vi "Monitor-BNET01.vi"() -> ()   [LabVIEW 2013]
uses:
  <vilib>/Utility/miscctls.llb/LVPoint32TypeDef.ctl
  data/ControlCAN.dll
panel:
  out "数据保存":bool
  out "强制操作":bool
  out "参数生成":bool
  out "参数配置":bool
  in  "保存间隔(S)":T1(ring)=enum."0.2"
  out "文件序号":u32
  out "dup path":path
  out "开始保存":bool
  out "BMS供电电压":dbl
  out "字符串":string="         （菜单可更改CAN设置)请连接CAN设备-------->"
  out "CAN初始化成功":bool
  out "CP":u8
  out "CC":dbl
  out "CC2":dbl
  out "AI1":dbl
  out "AI2":dbl
  out "平均电流":dbl
  out "外总压":dbl
  out "从板个数":u8
  out "Life":string="0"
  out "DO2":bool
  out "DO1":bool
  out "DI4":bool
  out "DI3":bool
  out "DI2":bool
  out "DI1":bool
  out "总正":bool
  out "总负":bool
  out "预充":bool
  out "充电":bool
  out "风机":bool
  out "加热":bool
  in  "总电压进度":u16(ring)
  in  "总电流进度":u16(ring)
  out "VCI_Receive 2":T2={"ID"=67604736, "TimeStamp"=193019994, "TimeFlag"=1, "SendType"=0, "RemoteFlag"=0, "ExternFlag"=1, "DataLen"=8, "Data1"=1, "Data2"=0, "Data3"=0, "Data4"=85, "Data5"=59, "Data6"=0, "Data7"=0, "Data8"=30, "Rsv1"=0, "Rsv2"=0, "Rsv3"=0}
  in  "动作保持时间":dbl=100000.0
  in  "故障信息":bool caption="查看高压板监控"
  in  "系统信息":bool caption="查看高压板监控"
  out "温度个数":i32
  out "大小":i32
  out "X标尺.刻度值[]":dbl[](array[numeric])
  out "坐标 2":T3 caption="坐标"
  in  "充电信息":bool caption="查看高压板监控"
  out "CAN 操作结果":bool=TRUE
  out "充电继电器 2":u16(ring) caption="风机继电器" items=["未闭合", "闭合", "故障", "保留"]
  out "加热继电器":u16(ring) caption="预充电继电器" items=["未闭合", "闭合", "故障", "保留"]
  in  "单箱信息":bool caption="查看高压板监控"
  in  "单板信息 3":bool caption="查看高压板监控"
  in  "诊断标定":bool caption="查看高压板监控"
  in  "电压温度":bool caption="查看高压板监控"
  in  "数据刷新":bool caption="全部监控"
  in  "保存数据 3":bool caption="全部监控"
  in  "CAN连接":bool caption="启动CAN"
  in  "参数设置":bool caption="启动CAN"
  in  "退出":bool caption="全部监控"
  in  "帮助":bool caption="全部监控"
  in  "Life超时":i32
  in  "模拟发送":bool
  out "充电超时2":i32
  out "充电超时1":i32
  out "P_IsInternal_B":bool
  in  "判定3":bool=TRUE
  in  "计数 2":i32
  in  "计数1":i32=26826
  out "电池故障4 4":u8
  out "电池故障3 4":u8
  out "电池故障2 4":u8
  out "电池故障 5":u8
  in  "数值":i32
  out "继电器状态":string[][](array[string])=[["", "", "", "", "", "", "", "", "", "", "", "", "", "", "", "", "", "", "", "", "", "", "", "", "", "", "", "", "", "", "0"], ["", "", "", "", "", "", "", "", "", "", "", "", "", "", "", "", "", "", "", "", "", "", "", "", "", "", "", "", "", "", "0"]]
  out "从板参数":T4(array[cluster])=[{"总电压"=0.0, "总电流"=0.0, "外总压"=0.0, "平均电流"=0.0, "SOC"=60.0, "SOH"=60.0, "最高电压"=0.0, "位置"=0.0, "最低电压"=0.0, "位置"=0.0, "压差"=0.0, "最高温度"=0.0, "位置"=0.0, "最低温度"=0.0, "位置"=0.0, "最大内阻"=0.0, "位置"=0.0, "最小内阻"=0.0, "位置"=0.0, "故障信息"="", "协议版本号"="", "应用类型"="", "波特率"="", "协议是否公开"="", "电池运行状态"="", "电池充满标志位"="", "Life:"=25.0}, {"总电压"=0.0, "总电流"=0.0, "外总压"=0.0, "平均电流"=0.0, "SOC"=60.0, "SOH"=60.0, "最高电压"=0.0, "位置"=0.0, "最低电压"=0.0, "位置"=0.0, "压差"=0.0, "最高温度"=0.0, "位置"=0.0, "最低温度"=0.0, "位置"=0.0, "最大内阻"=0.0, "位置"=0.0, "最小内阻"=0.0, "位置"=0.0, "故障信息"="", "协议版本号"="", "应用类型"="", "波特率"="", "协议是否公开"="", "电池运行状态"="", "电池充满标志位"="", "Life:"=25.0}, {"总电压"=0.0, "总电流"=0.0, "外总压"=0.0, "平均电流"=0.0, "SOC"=60.0, "SOH"=60.0, "最高电压"=0.0, "位置"=0.0, "最低电压"=0.0, "位置"=0.0, "压差"=0.0, "最高温度"=0.0, "位置"=0.0, "最低温度"=0.0, "位置"=0.0, "最大内阻"=0.0, "位置"=0.0, "最小内阻"=0.0, "位置"=0.0, "故障信息"="", "协议版本号"="", "应用类型"="", "波特率"="", "协议是否公开"="", "电池运行状态"="", "电池充满标志位"="", "Life:"=25.0}, {"总电压"=0.0, "总电流"=0.0, "外总压"=0.0, "平均电流"=0.0, "SOC"=60.0, "SOH"=60.0, "最高电压"=0.0, "位置"=0.0, "最低电压"=0.0, "位置"=0.0, "压差"=0.0, "最高温度"=0.0, "位置"=0.0, "最低温度"=0.0, "位置"=0.0, "最大内阻"=0.0, "位置"=0.0, "最小内阻"=0.0, "位置"=0.0, "故障信息"="", "协议版本号"="", "应用类型"="", "波特率"="", "协议是否公开"="", "电池运行状态"="", "电池充满标志位"="", "Life:"=25.0}, {"总电压"=0.0, "总电流"=0.0, "外总压"=0.0, "平均电流"=0.0, "SOC"=60.0, "SOH"=60.0, "最高电压"=0.0, "位置"=0.0, "最低电压"=0.0, "位置"=0.0, "压差"=0.0, "最高温度"=0.0, "位置"=0.0, "最低温度"=0.0, "位置"=0.0, "最大内阻"=0.0, "位置"=0.0, "最小内阻"=0.0, "位置"=0.0, "故障信息"="", "协议版本号"="", "应用类型"="", "波特率"="", "协议是否公开"="", "电池运行状态"="", "电池充满标志位"="", "Life:"=25.0}, {"总电压"=0.0, "总电流"=0.0, "外总压"=0.0, "平均电流"=0.0, "SOC"=60.0, "SOH"=60.0, "最高电压"=0.0, "位置"=0.0, "最低电压"=0.0, "位置"=0.0, "压差"=0.0, "最高温度"=0.0, "位置"=0.0, "最低温度"=0.0, "位置"=0.0, "最大内阻"=0.0, "位置"=0.0, "最小内阻"=0.0, "位置"=0.0, "故障信息"="", "协议版本号"="", "应用类型"="", "波特率"="", "协议是否公开"="", "电池运行状态"="", "电池充满标志位"="", "Life:"=25.0}, {"总电压"=0.0, "总电流"=0.0, "外总压"=0.0, "平均电流"=0.0, "SOC"=60.0, "SOH"=60.0, "最高电压"=0.0, "位置"=0.0, "最低电压"=0.0, "位置"=0.0, "压差"=0.0, "最高温度"=0.0, "位置"=0.0, "最低温度"=0.0, "位置"=0.0, "最大内阻"=0.0, "位置"=0.0, "最小内阻"=0.0, "位置"=0.0, "故障信息"="", "协议版本号"="", "应用类型"="", "波特率"="", "协议是否公开"="", "电池运行状态"="", "电池充满标志位"="", "Life:"=25.0}, {"总电压"=0.0, "总电流"=0.0, "外总压"=0.0, "平均电流"=0.0, "SOC"=60.0, "SOH"=60.0, "最高电压"=0.0, "位置"=0.0, "最低电压"=0.0, "位置"=0.0, "压差"=0.0, "最高温度"=0.0, "位置"=0.0, "最低温度"=0.0, "位置"=0.0, "最大内阻"=0.0, "位置"=0.0, "最小内阻"=0.0, "位置"=0.0, "故障信息"="", "协议版本号"="", "应用类型"="", "波特率"="", "协议是否公开"="", "电池运行状态"="", "电池充满标志位"="", "Life:"=25.0}, {"总电压"=0.0, "总电流"=0.0, "外总压"=0.0, "平均电流"=0.0, "SOC"=60.0, "SOH"=60.0, "最高电压"=0.0, "位置"=0.0, "最低电压"=0.0, "位置"=0.0, "压差"=0.0, "最高温度"=0.0, "位置"=0.0, "最低温度"=0.0, "位置"=0.0, "最大内阻"=0.0, "位置"=0.0, "最小内阻"=0.0, "位置"=0.0, "故障信息"="", "协议版本号"="", "应用类型"="", "波特率"="", "协议是否公开"="", "电池运行状态"="", "电池充满标志位"="", "Life:"=25.0}, {"总电压"=0.0, "总电流"=0.0, "外总压"=0.0, "平均电流"=0.0, "SOC"=60.0, "SOH"=60.0, "最高电压"=0.0, "位置"=0.0, "最低电压"=0.0, "位置"=0.0, "压差"=0.0, "最高温度"=0.0, "位置"=0.0, "最低温度"=0.0, "位置"=0.0, "最大内阻"=0.0, "位置"=0.0, "最小内阻"=0.0, "位置"=0.0, "故障信息"="", "协议版本号"="", "应用类型"="", "波特率"="", "协议是否公开"="", "电池运行状态"="", "电池充满标志位"="", "Life:"=25.0}, {"总电压"=0.0, "总电流"=0.0, "外总压"=0.0, "平均电流"=0.0, "SOC"=60.0, "SOH"=60.0, "最高电压"=0.0, "位置"=0.0, "最低电压"=0.0, "位置"=0.0, "压差"=0.0, "最高温度"=0.0, "位置"=0.0, "最低温度"=0.0, "位置"=0.0, "最大内阻"=0.0, "位置"=0.0, "最小内阻"=0.0, "位置"=0.0, "故障信息"="", "协议版本号"="", "应用类型"="", "波特率"="", "协议是否公开"="", "电池运行状态"="", "电池充满标志位"="", "Life:"=25.0}, {"总电压"=0.0, "总电流"=0.0, "外总压"=0.0, "平均电流"=0.0, "SOC"=60.0, "SOH"=60.0, "最高电压"=0.0, "位置"=0.0, "最低电压"=0.0, "位置"=0.0, "压差"=0.0, "最高温度"=0.0, "位置"=0.0, "最低温度"=0.0, "位置"=0.0, "最大内阻"=0.0, "位置"=0.0, "最小内阻"=0.0, "位置"=0.0, "故障信息"="", "协议版本号"="", "应用类型"="", "波特率"="", "协议是否公开"="", "电池运行状态"="", "电池充满标志位"="", "Life:"=25.0}, {"总电压"=0.0, "总电流"=0.0, "外总压"=0.0, "平均电流"=0.0, "SOC"=60.0, "SOH"=60.0, "最高电压"=0.0, "位置"=0.0, "最低电压"=0.0, "位置"=0.0, "压差"=0.0, "最高温度"=0.0, "位置"=0.0, "最低温度"=0.0, "位置"=0.0, "最大内阻"=0.0, "位置"=0.0, "最小内阻"=0.0, "位置"=0.0, "故障信息"="", "协议版本号"="", "应用类型"="", "波特率"="", "协议是否公开"="", "电池运行状态"="", "电池充满标志位"="", "Life:"=25.0}, {"总电压"=0.0, "总电流"=0.0, "外总压"=0.0, "平均电流"=0.0, "SOC"=60.0, "SOH"=60.0, "最高电压"=0.0, "位置"=0.0, "最低电压"=0.0, "位置"=0.0, "压差"=0.0, "最高温度"=0.0, "位置"=0.0, "最低温度"=0.0, "位置"=0.0, "最大内阻"=0.0, "位置"=0.0, "最小内阻"=0.0, "位置"=0.0, "故障信息"="", "协议版本号"="", "应用类型"="", "波特率"="", "协议是否公开"="", "电池运行状态"="", "电池充满标志位"="", "Life:"=25.0}, {"总电压"=0.0, "总电流"=0.0, "外总压"=0.0, "平均电流"=0.0, "SOC"=60.0, "SOH"=60.0, "最高电压"=0.0, "位置"=0.0, "最低电压"=0.0, "位置"=0.0, "压差"=0.0, "最高温度"=0.0, "位置"=0.0, "最低温度"=0.0, "位置"=0.0, "最大内阻"=0.0, "位置"=0.0, "最小内阻"=0.0, "位置"=0.0, "故障信息"="", "协议版本号"="", "应用类型"="", "波特率"="", "协议是否公开"="", "电池运行状态"="", "电池充满标志位"="", "Life:"=25.0}, {"总电压"=0.0, "总电流"=0.0, "外总压"=0.0, "平均电流"=0.0, "SOC"=60.0, "SOH"=60.0, "最高电压"=0.0, "位置"=0.0, "最低电压"=0.0, "位置"=0.0, "压差"=0.0, "最高温度"=0.0, "位置"=0.0, "最低温度"=0.0, "位置"=0.0, "最大内阻"=0.0, "位置"=0.0, "最小内阻"=0.0, "位置"=0.0, "故障信息"="", "协议版本号"="", "应用类型"="", "波特率"="", "协议是否公开"="", "电池运行状态"="", "电池充满标志位"="", "Life:"=25.0}, {"总电压"=0.0, "总电流"=0.0, "外总压"=0.0, "平均电流"=0.0, "SOC"=60.0, "SOH"=60.0, "最高电压"=0.0, "位置"=0.0, "最低电压"=0.0, "位置"=0.0, "压差"=0.0, "最高温度"=0.0, "位置"=0.0, "最低温度"=0.0, "位置"=0.0, "最大内阻"=0.0, "位置"=0.0, "最小内阻"=0.0, "位置"=0.0, "故障信息"="", "协议版本号"="", "应用类型"="", "波特率"="", "协议是否公开"="", "电池运行状态"="", "电池充满标志位"="", "Life:"=25.0}, {"总电压"=0.0, "总电流"=0.0, "外总压"=0.0, "平均电流"=0.0, "SOC"=60.0, "SOH"=60.0, "最高电压"=0.0, "位置"=0.0, "最低电压"=0.0, "位置"=0.0, "压差"=0.0, "最高温度"=0.0, "位置"=0.0, "最低温度"=0.0, "位置"=0.0, "最大内阻"=0.0, "位置"=0.0, "最小内阻"=0.0, "位置"=0.0, "故障信息"="", "协议版本号"="", "应用类型"="", "波特率"="", "协议是否公开"="", "电池运行状态"="", "电池充满标志位"="", "Life:"=25.0}, {"总电压"=0.0, "总电流"=0.0, "外总压"=0.0, "平均电流"=0.0, "SOC"=60.0, "SOH"=60.0, "最高电压"=0.0, "位置"=0.0, "最低电压"=0.0, "位置"=0.0, "压差"=0.0, "最高温度"=0.0, "位置"=0.0, "最低温度"=0.0, "位置"=0.0, "最大内阻"=0.0, "位置"=0.0, "最小内阻"=0.0, "位置"=0.0, "故障信息"="", "协议版本号"="", "应用类型"="", "波特率"="", "协议是否公开"="", "电池运行状态"="", "电池充满标志位"="", "Life:"=25.0}, {"总电压"=0.0, "总电流"=0.0, "外总压"=0.0, "平均电流"=0.0, "SOC"=60.0, "SOH"=60.0, "最高电压"=0.0, "位置"=0.0, "最低电压"=0.0, "位置"=0.0, "压差"=0.0, "最高温度"=0.0, "位置"=0.0, "最低温度"=0.0, "位置"=0.0, "最大内阻"=0.0, "位置"=0.0, "最小内阻"=0.0, "位置"=0.0, "故障信息"="", "协议版本号"="", "应用类型"="", "波特率"="", "协议是否公开"="", "电池运行状态"="", "电池充满标志位"="", "Life:"=25.0}, {"总电压"=0.0, "总电流"=0.0, "外总压"=0.0, "平均电流"=0.0, "SOC"=60.0, "SOH"=60.0, "最高电压"=0.0, "位置"=0.0, "最低电压"=0.0, "位置"=0.0, "压差"=0.0, "最高温度"=0.0, "位置"=0.0, "最低温度"=0.0, "位置"=0.0, "最大内阻"=0.0, "位置"=0.0, "最小内阻"=0.0, "位置"=0.0, "故障信息"="", "协议版本号"="", "应用类型"="", "波特率"="", "协议是否公开"="", "电池运行状态"="", "电池充满标志位"="", "Life:"=25.0}, {"总电压"=0.0, "总电流"=0.0, "外总压"=0.0, "平均电流"=0.0, "SOC"=60.0, "SOH"=60.0, "最高电压"=0.0, "位置"=0.0, "最低电压"=0.0, "位置"=0.0, "压差"=0.0, "最高温度"=0.0, "位置"=0.0, "最低温度"=0.0, "位置"=0.0, "最大内阻"=0.0, "位置"=0.0, "最小内阻"=0.0, "位置"=0.0, "故障信息"="", "协议版本号"="", "应用类型"="", "波特率"="", "协议是否公开"="", "电池运行状态"="", "电池充满标志位"="", "Life:"=25.0}, {"总电压"=0.0, "总电流"=0.0, "外总压"=0.0, "平均电流"=0.0, "SOC"=60.0, "SOH"=60.0, "最高电压"=0.0, "位置"=0.0, "最低电压"=0.0, "位置"=0.0, "压差"=0.0, "最高温度"=0.0, "位置"=0.0, "最低温度"=0.0, "位置"=0.0, "最大内阻"=0.0, "位置"=0.0, "最小内阻"=0.0, "位置"=0.0, "故障信息"="", "协议版本号"="", "应用类型"="", "波特率"="", "协议是否公开"="", "电池运行状态"="", "电池充满标志位"="", "Life:"=25.0}, {"总电压"=0.0, "总电流"=0.0, "外总压"=0.0, "平均电流"=0.0, "SOC"=60.0, "SOH"=60.0, "最高电压"=0.0, "位置"=0.0, "最低电压"=0.0, "位置"=0.0, "压差"=0.0, "最高温度"=0.0, "位置"=0.0, "最低温度"=0.0, "位置"=0.0, "最大内阻"=0.0, "位置"=0.0, "最小内阻"=0.0, "位置"=0.0, "故障信息"="", "协议版本号"="", "应用类型"="", "波特率"="", "协议是否公开"="", "电池运行状态"="", "电池充满标志位"="", "Life:"=25.0}, {"总电压"=0.0, "总电流"=0.0, "外总压"=0.0, "平均电流"=0.0, "SOC"=60.0, "SOH"=60.0, "最高电压"=0.0, "位置"=0.0, "最低电压"=0.0, "位置"=0.0, "压差"=0.0, "最高温度"=0.0, "位置"=0.0, "最低温度"=0.0, "位置"=0.0, "最大内阻"=0.0, "位置"=0.0, "最小内阻"=0.0, "位置"=0.0, "故障信息"="", "协议版本号"="", "应用类型"="", "波特率"="", "协议是否公开"="", "电池运行状态"="", "电池充满标志位"="", "Life:"=25.0}, {"总电压"=0.0, "总电流"=0.0, "外总压"=0.0, "平均电流"=0.0, "SOC"=60.0, "SOH"=60.0, "最高电压"=0.0, "位置"=0.0, "最低电压"=0.0, "位置"=0.0, "压差"=0.0, "最高温度"=0.0, "位置"=0.0, "最低温度"=0.0, "位置"=0.0, "最大内阻"=0.0, "位置"=0.0, "最小内阻"=0.0, "位置"=0.0, "故障信息"="", "协议版本号"="", "应用类型"="", "波特率"="", "协议是否公开"="", "电池运行状态"="", "电池充满标志位"="", "Life:"=25.0}, {"总电压"=0.0, "总电流"=0.0, "外总压"=0.0, "平均电流"=0.0, "SOC"=60.0, "SOH"=60.0, "最高电压"=0.0, "位置"=0.0, "最低电压"=0.0, "位置"=0.0, "压差"=0.0, "最高温度"=0.0, "位置"=0.0, "最低温度"=0.0, "位置"=0.0, "最大内阻"=0.0, "位置"=0.0, "最小内阻"=0.0, "位置"=0.0, "故障信息"="", "协议版本号"="", "应用类型"="", "波特率"="", "协议是否公开"="", "电池运行状态"="", "电池充满标志位"="", "Life:"=25.0}, {"总电压"=0.0, "总电流"=0.0, "外总压"=0.0, "平均电流"=0.0, "SOC"=60.0, "SOH"=60.0, "最高电压"=0.0, "位置"=0.0, "最低电压"=0.0, "位置"=0.0, "压差"=0.0, "最高温度"=0.0, "位置"=0.0, "最低温度"=0.0, "位置"=0.0, "最大内阻"=0.0, "位置"=0.0, "最小内阻"=0.0, "位置"=0.0, "故障信息"="", "协议版本号"="", "应用类型"="", "波特率"="", "协议是否公开"="", "电池运行状态"="", "电池充满标志位"="", "Life:"=25.0}, {"总电压"=0.0, "总电流"=0.0, "外总压"=0.0, "平均电流"=0.0, "SOC"=60.0, "SOH"=60.0, "最高电压"=0.0, "位置"=0.0, "最低电压"=0.0, "位置"=0.0, "压差"=0.0, "最高温度"=0.0, "位置"=0.0, "最低温度"=0.0, "位置"=0.0, "最大内阻"=0.0, "位置"=0.0, "最小内阻"=0.0, "位置"=0.0, "故障信息"="", "协议版本号"="", "应用类型"="", "波特率"="", "协议是否公开"="", "电池运行状态"="", "电池充满标志位"="", "Life:"=25.0}, {"总电压"=0.0, "总电流"=0.0, "外总压"=0.0, "平均电流"=0.0, "SOC"=60.0, "SOH"=60.0, "最高电压"=0.0, "位置"=0.0, "最低电压"=0.0, "位置"=0.0, "压差"=0.0, "最高温度"=0.0, "位置"=0.0, "最低温度"=0.0, "位置"=0.0, "最大内阻"=0.0, "位置"=0.0, "最小内阻"=0.0, "位置"=0.0, "故障信息"="", "协议版本号"="", "应用类型"="", "波特率"="", "协议是否公开"="", "电池运行状态"="", "电池充满标志位"="", "Life:"=25.0}, {"总电压"=0.0, "总电流"=0.0, "外总压"=0.0, "平均电流"=0.0, "SOC"=60.0, "SOH"=60.0, "最高电压"=0.0, "位置"=0.0, "最低电压"=0.0, "位置"=0.0, "压差"=0.0, "最高温度"=0.0, "位置"=0.0, "最低温度"=0.0, "位置"=0.0, "最大内阻"=0.0, "位置"=0.0, "最小内阻"=0.0, "位置"=0.0, "故障信息"="", "协议版本号"="", "应用类型"="", "波特率"="", "协议是否公开"="", "电池运行状态"="", "电池充满标志位"="", "Life:"=25.0}] {"SOH" scale=0.0..100.0 scale format="%#.0f"; "SOC" scale=0.0..100.0 scale format="%#.0f"}
  out "总电压(V)":dbl
  out "正级继电器":u16(ring) caption="总正继电器" items=["未闭合", "闭合", "故障", "保留"]
  out "状态":bool=TRUE
  out "SOH":sgl(slide) scale=0.0..100.0 scale format="%#.1f"
  out "充电继电器":u16(ring)=1 items=["未闭合", "闭合", "故障", "保留"]
  out "预充继电器":u16(ring) caption="预充电继电器" items=["未闭合", "闭合", "故障", "保留"]
  out "负级继电器":u16(ring) caption="总极继电器" items=["未闭合", "闭合", "故障", "保留"]
  out "LIFE":string
  out "故障信息概况":string="存在故障"
  out "BMS时间":string="2015-10-28 15:35:59" caption="BMS:"
  out "电池系统绝缘状态":string="正常"
  out "SOC":dbl(slide) scale=0.0..100.0 scale format="%0.1f%%"
  out "从板个数":dbl=3.0
  out "保存时间输入(ms)":dbl=1000.0
  out "保存数据":bool
  out "SOC(红)":sgl(slide)=100.0 caption="SOC" scale=0.0..100.0 scale format="%#_6f"
  out "SOC(黄)":sgl(slide)=100.0 caption="SOC" scale=0.0..100.0 scale format="%#.1f"
  in  "图表选项卡":enum32{"次要参数", "单体电压", "单体温度", "单体内阻"}(tab)
  out "次要参数":T5={"最高单体电压"=0.0, "最高电压位置"=0.0, "最低单体电压"=0.0, "最低电压位置"=0.0, "压差"=0.0, "最高单体温度"=0.0, "最高温度位置"=0.0, "最低单体温度"=0.0, "最低温度位置"=0.0, "温差"=0.0, "最高单体内阻"=0.0, "最高内阻位置"=0.0, "最低单体内阻"=0.0, "最低内阻位置"=0.0, "总内阻"=0.0, "协议是否公开"="Not public", "协议版本号"="V0.0", "应用类型"="", "波特率"="500Kps"} {"总内阻" format="%#.0f"; "最低内阻位置" format="%#.0f"; "最低单体内阻" format="%#.2f"; "最高内阻位置" format="%#.2f"; "最高单体内阻" format="%#.2f"; "温差" format="%#.0f"; "最低温度位置" format="%#.0f"; "最低单体温度" format="%#.0f"; "最高温度位置" format="%#.0f"; "最高单体温度" format="%#.0f"; "压差" format="%.3f"; "最低电压位置" format="%#.0f"; "最低单体电压" format="%.3f"; "最高电压位置" format="%#.3f"; "最高单体电压" format="%.3f"}
  out "System XY Graph":cluster{i32[], dbl[]}(graph)
  in  "1:":dbl caption="103"
  out "System XY Graph 3":cluster{i32[], dbl[]}(graph)
  in  "1: 2":dbl caption="11"
  out "XY图":cluster{i32[], dbl[]}(graph)
  out "Life:":dbl=25.0
  out "E-U_baud":u32(ring)=393223 items=["0x060007--500Kbps"=393223, "0x1C0008--250Kbps"=1835016, "0x1C0011--125Kbps"=1835025, "0x160023--100Kbps"=1441827, "0x1C002C--50Kbps"=1835052, "0x1600B3--20Kbps"=1441971, "0x1C00E0--10Kbps"=1835232, "0x1C01C1--5Kbps"=1835457]
  out "上电状态":T6={"主板"=TRUE, "高压板"=TRUE, "1"=FALSE, "2"=FALSE, "3"=FALSE, "4"=TRUE, "5"=FALSE, "6"=FALSE, "7"=TRUE, "8"=FALSE, "9"=FALSE, "10"=FALSE, "11"=FALSE, "12"=FALSE, "13"=FALSE, "14"=FALSE, "15"=FALSE, "16"=FALSE, "17"=FALSE, "18"=FALSE, "19"=FALSE, "20"=FALSE, "21"=FALSE, "22"=FALSE, "23"=FALSE, "24"=FALSE, "25"=FALSE}
  in  "自动识别CAN卡":bool
  in  "CAN卡类型":u32(ring)=21 items=["USBCAN1"=3, "USBCAN2"=4, "CAN_E_U"=20, "CAN_2E_U"=21]
  out "工作方式":u8(ring) items=["Normal", "Listen Only"]
  out "滤波方式":u8(ring) items=["Dual Filter", "Single Filter"]
  in  "波特率":u16(ring)=1 items=["250K", "500K"]
  in  "CAN端口":u16(ring) caption="端口" items=["0", "1"]
  in  "设备索引号":u16(ring) caption="索引号" items=["0", "1", "2", "3", "4", "5", "6", "7", "8", "9", "10", "11", "12", "13", "14", "15", ""]
  in  "选项卡控件 3":enum32{"选项卡 1", "选项卡 2"}(tab)
  in  "详细信息 4":bool caption="查看高压板监控"
  in  "中英文选择":enum32{"中文", "English"}(radio)
  in  "帮助 2":bool caption="全部监控"
  in  "保存数据 2":bool caption="全部监控"
  in  "启动CAN 2":bool caption="启动CAN"
  in  "界面刷新 2":bool caption="全部监控"
  in  "退出 2":bool caption="全部监控"
  in  "详细信息 3":bool caption="查看高压板监控"
  in  "诊断标定 3":bool caption="查看高压板监控"
  in  "参数设置 2":bool caption="启动CAN"
  out "外总压":dbl(knob) scale=0.0..800.0
  out "状态 2":string caption="状态"
  in  "主界面选项":T7(radio)
  out "总电流(A)":dbl
  out "系统运行模式":string="系统待命"
  in  "暂停 3":bool caption="温度暂停"
  in  "数值保存7":bool=TRUE
  out "充电超时4":i32
  out "充电超时3":i32
  in  "输出簇":T8
  out "电池故障 22":string="0A00000300000000"
  out "电池故障 21":string="000000000000000"
  out "电池故障 20":string="0000000000000000"
  out "电池故障 19":string="3BF0333000000000"
  out "状态":string caption="系统连接状态"
  out "上电状态":bool[](array[boolean])=[TRUE, TRUE, TRUE, TRUE, FALSE, FALSE, FALSE, FALSE, FALSE, FALSE, FALSE, FALSE, FALSE, FALSE, FALSE, FALSE, FALSE, FALSE, FALSE, FALSE, FALSE, FALSE, FALSE, FALSE, FALSE, FALSE, FALSE, FALSE, FALSE, FALSE, FALSE]
  out "数据位置":dbl[](array[numeric])
  out "输出数据":dbl[](array[numeric])
  in  "VCI_Receive":T2 {"Rsv3" max=0 format="%x"; "Rsv2" min=101 format="%x"; "Rsv1" format="%x"; "Data8" format="%x"; "Data7" format="%x"; "Data6" format="%x"; "Data5" format="%x"; "Data4" format="%x"; "Data3" format="%x"; "Data2" format="%x"; "Data1" format="%x"; "DataLen" format="%x"; "ExternFlag" format="%x"; "RemoteFlag" format="%x"; "SendType" format="%x"; "TimeFlag" format="%x"; "TimeStamp" format="%x"; "ID" format="%x"}
  out "VCI_CAN_OBJ_R":T9={"ID"=0, "TimeStamp"=0, "TimeFlag"=0, "SendType"=1, "RemoteFlag"=0, "ExternFlag"=0, "DataLen"=8, 0, 0, 0, 0, 0, 0, 0, 0, 0, 0, 0}
  out "CANStartup":bool
  # "监控上位机"
  # "PASS:1245"
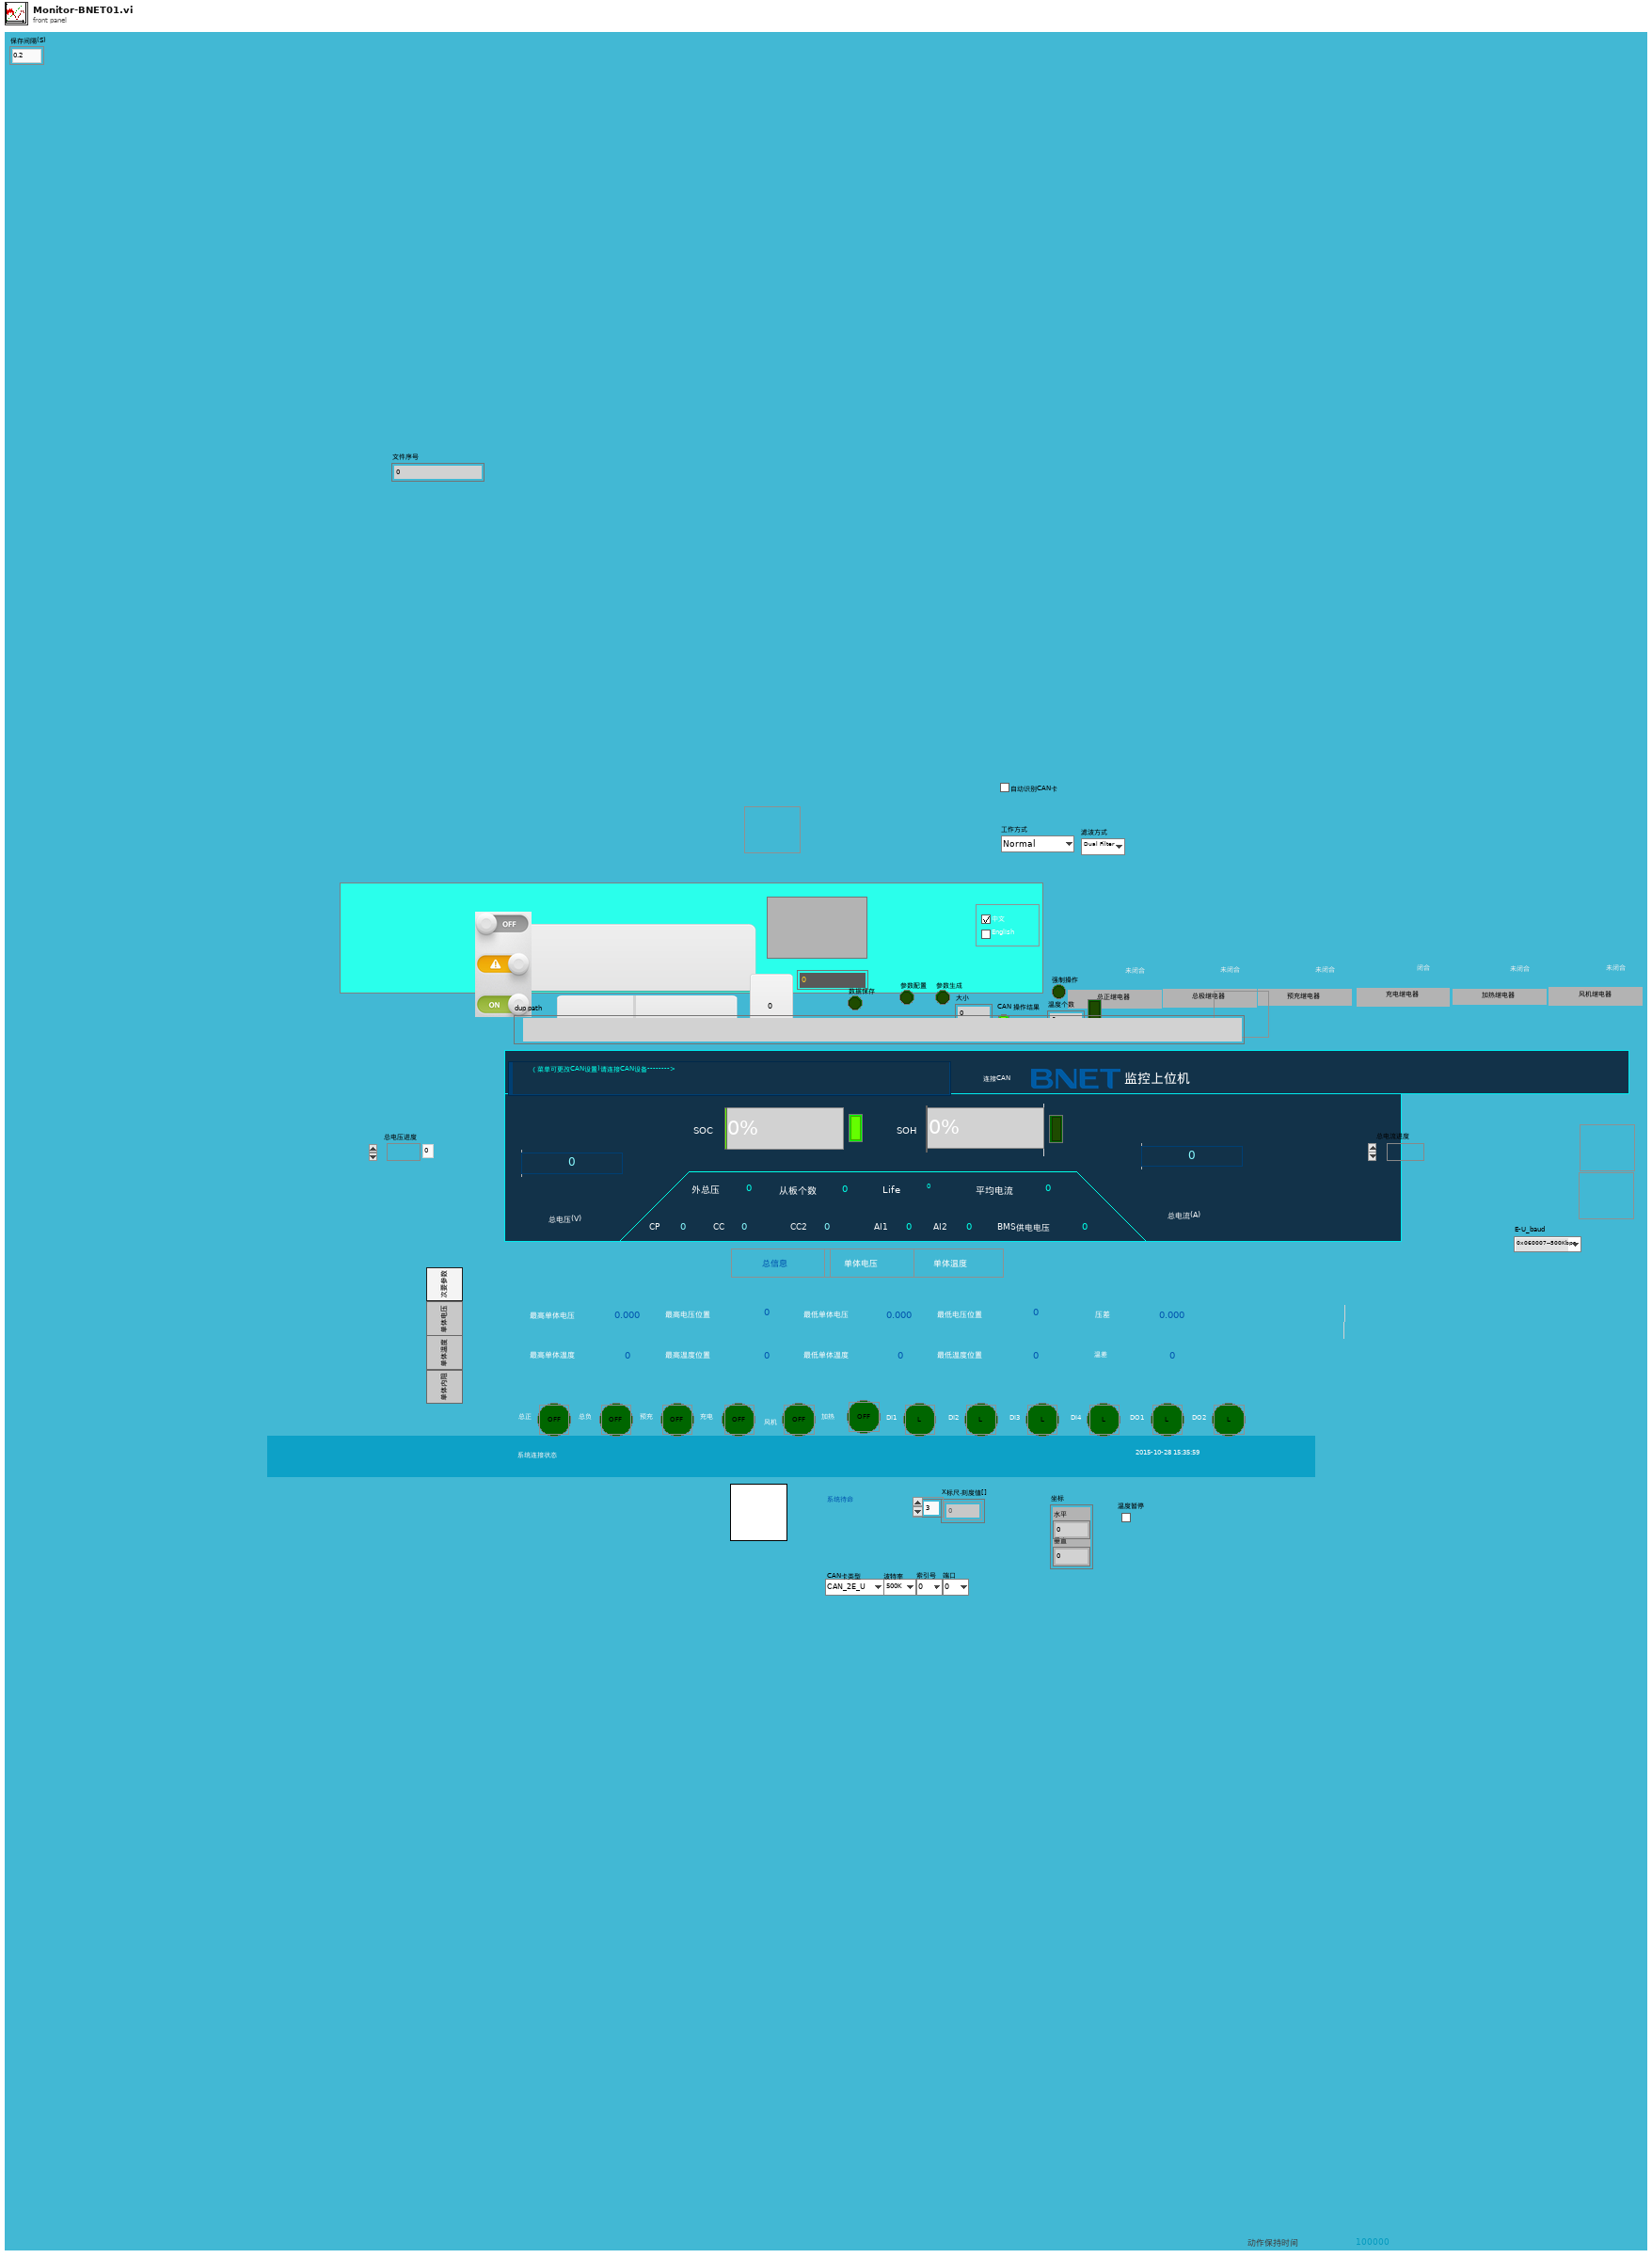
[diagram p1: front panel]
types:
  T1 = enum16{"0.1", "0.2", "0.3", "0.4", "0.5", "1", "2", "3", "4"}
  T2 = cluster{"ID":u32, "TimeStamp":u32, "TimeFlag":u8, "SendType":u8, "RemoteFlag":u8, "ExternFlag":u8, "DataLen":u8, "Data1":u8, "Data2":u8, "Data3":u8, "Data4":u8, "Data5":u8, "Data6":u8, "Data7":u8, "Data8":u8, "Rsv1":u8, "Rsv2":u8, "Rsv3":u8}
  T3 = typedef "LVPoint32TypeDef.ctl" = cluster{"Horizontal":i32, "Vertical":i32}
  T4 = cluster{"总电压":dbl, "总电流":dbl, "外总压":dbl, "平均电流":dbl, "SOC":dbl, "SOH":dbl, "最高电压":dbl, "位置":dbl, "最低电压":dbl, "位置":dbl, "压差":dbl, "最高温度":dbl, "位置":dbl, "最低温度":dbl, "位置":dbl, "最大内阻":dbl, "位置":dbl, "最小内阻":dbl, "位置":dbl, "故障信息":string, "协议版本号":string, "应用类型":string, "波特率":string, "协议是否公开":string, "电池运行状态":string, "电池充满标志位":string, "Life:":dbl}[]
  T5 = cluster{"最高单体电压":dbl, "最高电压位置":dbl, "最低单体电压":dbl, "最低电压位置":dbl, "压差":dbl, "最高单体温度":dbl, "最高温度位置":dbl, "最低单体温度":dbl, "最低温度位置":dbl, "温差":dbl, "最高单体内阻":dbl, "最高内阻位置":dbl, "最低单体内阻":dbl, "最低内阻位置":dbl, "总内阻":dbl, "协议是否公开":string, "协议版本号":string, "应用类型":string, "波特率":string}
  T6 = cluster{"主板":bool, "高压板":bool, "1":bool, "2":bool, "3":bool, "4":bool, "5":bool, "6":bool, "7":bool, "8":bool, "9":bool, "10":bool, "11":bool, "12":bool, "13":bool, "14":bool, "15":bool, "16":bool, "17":bool, "18":bool, "19":bool, "20":bool, "21":bool, "22":bool, "23":bool, "24":bool, "25":bool}
  T7 = enum32{"单选选项2 4", "单选选项2 5", "总信息卡", "单体电压卡", "单体温度卡"}
  T8 = cluster{"return type":u32, "pReceive":cluster{"ID":u32, "TimeStamp":u32, "TimeFlag":u8, "SendType":u8, "RemoteFlag":u8, "ExternFlag":u8, "DataLen":u8, u8, u8, u8, u8, u8, u8, u8, u8, u8, u8, u8}[]}
  T9 = cluster{"ID":u32, "TimeStamp":u32, "TimeFlag":u8, "SendType":u8, "RemoteFlag":u8, "ExternFlag":u8, "DataLen":u8, u8, u8, u8, u8, u8, u8, u8, u8, u8, u8, u8}
  T10 = enum32{"Invalid", "Standard", "Closed", "Hidden", "Minimized", "Maximized"}
  T11 = enum8{"Enabled", "Disabled", "Disabled and Grayed Out"}
  T12 = enum16{"5Kbps", "10Kbps", "20Kbps", "40Kbps", "50Kbps", "80Kbps", "100Kbps", "125Kbps", "200Kbps", "250Kbps", "400Kbps", "500Kbps", "666Kbps", "800Kbps", "1000Kbps"}
  T13 = enum32{"次要参数", "单体电压", "单体温度", "单体内阻", "总电压 总电流"}
  T14 = cluster{"打开CAN":bool, "初始化CAN":bool, "开始CAN":bool, "重启":bool, "关闭CAN":bool}
  T15 = typedef "LVBoundsTypeDef.ctl" = cluster{"Width":u32, "Height":u32}
  T16 = typedef "LVRectTypeDef.ctl" = cluster{"Left":i16, "Top":i16, "Right":i16, "Bottom":i16}
  T17 = cluster{"版本号":string, "应用类型":string, "波特率":string, "协议是否公开":string}
  T18 = cluster{"ID":u32, "TimeStamp":u32, "TimeFlag":u8, "SendType":u8, "RemoteFlag":u8, "ExternFlag":u8, "DataLen":u8, u8, u8, u8, u8, u8, u8, u8, u8, u8, u8, u8}[]
  T19 = cluster{"return type":u32, "pReceive":cluster{"ID":u32, "TimeStamp":u32, "TimeFlag":u8, "SendType":u8, "RemoteFlag":u8, "ExternFlag":u8, "DataLen":u8, "1":u8, "2":u8, "3":u8, "4":u8, "5":u8, "6":u8, "7":u8, "8":u8, "9":u8, "10":u8, "11":u8}[]}
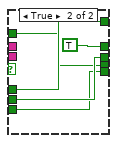
[diagram p2: hidden frame]
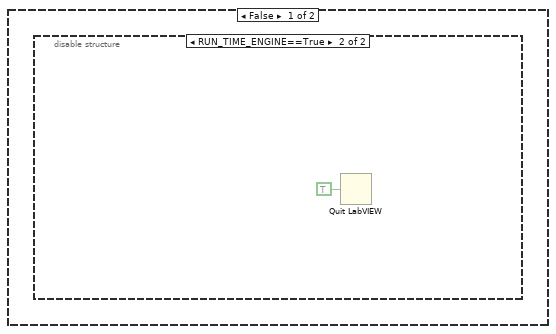
[diagram p3: hidden frame]
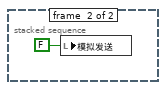
[diagram p6: hidden frame]
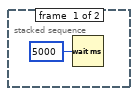
[diagram p9: hidden frame]
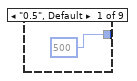
[diagram p10: hidden frame]
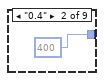
[diagram p11: hidden frame]
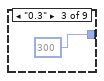
[diagram p12: hidden frame]
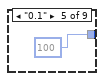
[diagram p13: hidden frame]
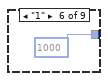
[diagram p14: hidden frame]
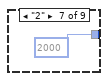
[diagram p15: hidden frame]
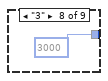
[diagram p16: hidden frame]
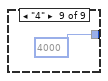
[diagram p17: hidden frame]
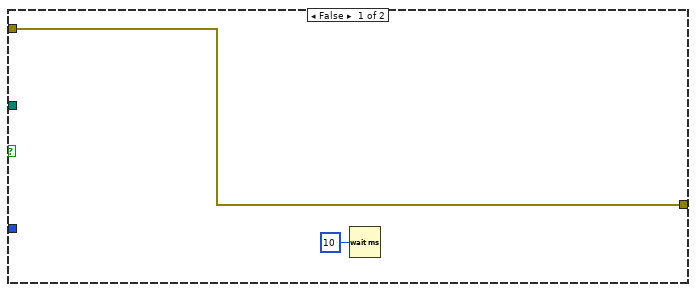
[diagram p19: hidden frame]
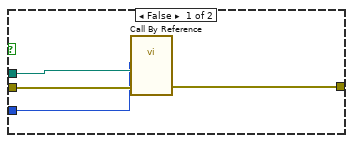
[diagram p20: hidden frame]
diagram:
  w21 = 0.0 ("外总压")
  w23 = 0.0 ("BMS供电电压")
  w48 = u32 16448250
  w49 = FALSE ("总正：")
  w50 = 0.0 ("CC")
  w51 = FALSE ("DI3")
  w53 = u16 0 ("总电压进度")
  n1 = stacked-sequence {
    frame #0 {
      w56 = u16 1 items=["250K", "500K"] ("波特率")
      w58 = u8 0 items=["Normal", "Listen Only"] ("工作方式")
      w59 = u16 0 items=["0", "1", "2", "3", "4", "5", "6", "7", "8", "9", "10", "11", "12", "13", "14", "15", ""] ("设备索引号")
      w62 = u16 0 items=["0", "1", "2", "3", "4", "5", "6", "7", "8", "9", "10", "11", "12", "13", "14", "15", ""] ("设备索引号")
      w60 = u16 0 items=["0", "1"] ("CAN端口")
      w63 = u32 393223 items=["0x060003--1000Kbps"=393219, "0x060004--800Kbps"=393220, "0x060007--500Kbps"=393223, "0x1C0008--250Kbps"=1835016, "0x1C0011--125Kbps"=1835025, "0x160023--100Kbps"=1441827, "0x1C002C--50Kbps"=1835052, "0x1600B3--20Kbps"=1441971, "0x1C00E0--10Kbps"=1835232, "0x1C01C1--5Kbps"=1835457] ("E-U_baud")
      w61 = u32 21 items=["PCI5121"=1, "PCI9810"=2, "USBCAN1"=3, "USBCAN2"=4, "PCI9820"=5, "PCI5110"=7, "CANLite(mini)"=8, "ISA9620"=9, "ISA5420"=10, "PC104CAN"=11, "DNP9810"=13, "PCI9840B"=14, "PC104C2"=15, "PCI9820I"=16, "pec9920"=18, "USBCAN_E_U"=20, "USBCAN_2E_U"=21] ("CAN卡类型")
      w64 = T11."Enabled" ("禁用")
      w77 = 0 ("索引")
      w65 = TRUE ("保存表头1")
      w66 = FALSE ("可见")
      n2 = global write "全局 1.vi" "保存停止"(w65) -> ()
      n3 = local write "数值保存7"(w65) -> ()
      n4 = local write "判定3"(w65) -> ()
      n5 = global write "EV05全局变量1.vi" "退出"(w65) -> ()
      n6 = local write "CAN卡类型"(w61) -> ()
      n7 = global write "EV05全局变量1.vi" "CAN卡类型"(w61) -> ()
      n8 = global write "EV05全局变量1.vi" "存储语言"(cluster{"English":bool, "中文":bool} {"English"=TRUE, "中文"=FALSE} ("存储语言")) -> ()
      n9 = property on="SOC" class="Slide (严格)"("Visible"=w65) -> ()  [unwired: 2 in, 2 out]
      n10 = control-ref of="单选选项2 4"() -> (w68:refnum<vi>)
      n11 = control-ref of="单选选项2 5"() -> (w67:refnum<vi>)
      n12 = control-ref of="单体温度卡"() -> (w69:refnum<vi>)
      n13 = control-ref of="单体电压卡"() -> (w70:refnum<vi>)
      n14 = control-ref of="总信息卡"() -> (w71:refnum<vi>)
      n15 = property on="系统信息" class="Bool (严格)"("Disabled"=w64) -> ()  [unwired: 2 in, 2 out]
      n16 = property on="单箱信息" class="Bool (严格)"("Disabled"=w64) -> ()  [unwired: 2 in, 2 out]
      n17 = property on="诊断标定" class="Bool (严格)"("Disabled"=w64) -> ()  [unwired: 2 in, 2 out]
      n18 = property on="电压温度" class="Bool (严格)"("Disabled"=w64) -> ()  [unwired: 2 in, 2 out]
      n19 = property on="参数设置" class="Bool (严格)"("Disabled"=w64) -> ()  [unwired: 2 in, 2 out]
      n20 = Build Array(w71, w70, w69, w68, w67) -> (w76:refnum<vi>[])
      n21 = global write "EV05全局变量1.vi" "E-U_baud"(w63) -> ()
      n22 = global write "EV05全局变量1.vi" "波特率"(T12."500Kbps" ("波特率")) -> ()
      n23 = Delete From Array(array=w76, index=w77) -> (deleted portion=w74:refnum<vi>, array with subset deleted=w75:refnum<vi>[])  [unwired: 1 in]
      n24 = local write "主界面选项"(w77) -> ()
      n25 = local write "电池故障 5"(w64) -> ()
      n26 = local write "电池故障2 4"(w64) -> ()
      n27 = local write "电池故障3 4"(w64) -> ()
      n28 = local write "电池故障4 4"(w64) -> ()
      n29 = local write "计数 2"(w64) -> ()
      n30 = local write "图表选项卡"(enum32{"次要参数", "单体电压", "单体温度", "单体内阻"}."次要参数" ("图表选项卡")) -> ()
      n31 = for {
        tunnel: w75 -> [w82] mode=indexing
        tunnel: u32 16448250 -> [w81]
        n32 = property class="Bool (严格)"(reference=w82, "BoolText.TextColor"=w81) -> ()  [unwired: 1 in, 2 out]
      }
      n33 = global write "EV05全局变量1.vi" "设备索引号"(w62) -> ()
      n34 = global write "EV05全局变量1.vi" "CAN端口"(w60) -> ()
      n35 = property class="Bool (严格)"(reference=w74, "BoolText.TextColor"=u32 87470) -> ()  [unwired: 1 in, 2 out]
      n36 = local write "CAN端口"(w60) -> ()
      n37 = property on="详细信息 4" class="Bool (严格)"("Disabled"=w64) -> ()  [unwired: 2 in, 2 out]
      n38 = property on="详细信息 3" class="Bool (严格)"("Disabled"=w64) -> ()  [unwired: 2 in, 2 out]
      n39 = property on="诊断标定 3" class="Bool (严格)"("Disabled"=w64) -> ()  [unwired: 2 in, 2 out]
      n40 = property on="单板信息 3" class="Bool (严格)"("Disabled"=w64) -> ()  [unwired: 2 in, 2 out]
      n41 = local write "CAN初始化成功"(w66) -> ()
      n42 = local write "CAN连接"(w66) -> ()
      n43 = local write "退出"(w66) -> ()
      n44 = property on="单选选项2 4" class="Bool (严格)"("Visible"=w66) -> ()  [unwired: 2 in, 2 out]
      n45 = local write "Life超时"(w64) -> ()
      n46 = property on="SOC(黄)" class="Slide (严格)"("Visible"=w66) -> ()  [unwired: 2 in, 2 out]
      n47 = property on="SOC(红)" class="Slide (严格)"("Visible"=w66) -> ()  [unwired: 2 in, 2 out]
      n48 = local write "数值"(0 ("数值")) -> ()
      n49 = local write "工作方式"(w58) -> ()
      n50 = local write "设备索引号"(w59) -> ()
      n51 = local write "波特率"(w56) -> ()
      "保存数据" <- w66
      "状态 2" <- ""
      "充电超时1" <- w64
      "充电超时2" <- w64
      "充电超时3" <- w64
      "充电超时4" <- w64
    }
  }
  n52 = property on="字符串" class="Str"("Visible"=TRUE ("可见")) -> ()  [unwired: 2 in, 2 out]
  n53 = local write "动作保持时间"(100000.0 ("动作保持时间")) -> ()
  n54 = property on="故障信息" class="Bool (严格)"("BoolText.TextColor"=w48) -> ()  [unwired: 2 in, 2 out]
  n55 = property on="CAN连接" class="Bool (严格)"("BoolText.TextColor"=u32 16448250) -> ()  [unwired: 2 in, 2 out]
  n56 = property on="充电信息" class="Bool (严格)"("BoolText.TextColor"=w48) -> ()  [unwired: 2 in, 2 out]
  n57 = property on="诊断标定" class="Bool (严格)"("BoolText.TextColor"=w48) -> ()  [unwired: 2 in, 2 out]
  n58 = property on="单箱信息" class="Bool (严格)"("BoolText.TextColor"=w48) -> ()  [unwired: 2 in, 2 out]
  n59 = property on="电压温度" class="Bool (严格)"("BoolText.TextColor"=w48) -> ()  [unwired: 2 in, 2 out]
  n60 = property on="系统信息" class="Bool (严格)"("BoolText.TextColor"=w48) -> ()  [unwired: 2 in, 2 out]
  n61 = local write "DI3"(w51) -> ()
  n62 = local write "CP"(w50) -> ()
  n63 = local write "CC2"(w50) -> ()
  n64 = local write "DI2"(w51) -> ()
  n65 = local write "DI1"(w51) -> ()
  n66 = local write "AI1"(w50) -> ()
  n67 = local write "AI2"(w50) -> ()
  n68 = local write "DI4"(w51) -> ()
  n69 = local write "CC"(w50) -> ()
  n70 = local write "加热"(w51) -> ()
  n71 = local write "DO2"(w51) -> ()
  n72 = local write "风机"(w51) -> ()
  n73 = local write "DO1"(w51) -> ()
  n74 = Current VI's Path() -> (path=w16:path)
  n75 = Open VI Reference(vi path=w16) -> (vi reference=w13:refnum<vi>)  [unwired: 5 in, 1 out]
  n76 = invoke class="VI" method="FP.Open"(reference=w13, "Activate"=TRUE ("激活？"), "State"=T10."Hidden" ("状态")) -> (reference out=w12:refnum<vi>)  [unwired: 2 in, 4 out]
  n77 = local write "保存数据"(TRUE ("保存数据")) -> ()
  n78 = local write "总电流进度"(w53) -> ()
  n79 = local write "总电压进度"(w53) -> ()
  n80 = local write "总电流(A)"(w21) -> ()
  n81 = local write "平均电流"(w21) -> ()
  n82 = local write "外总压"(w21) -> ()
  n83 = local write "总电压(V)"(w21) -> ()
  n84 = local read "VCI_Receive"() -> (w37:T2)
  n85 = call-by-ref "?"() -> ("数据保存"=w1:bool, "强制操作"=w2:bool, "LicCode"=w5:string, "机器码"=w6:string, "参数生成"=w3:bool, "参数配置"=w4:bool, "鉴权通过"=w7:bool)  [unwired: 6 in, 2 out]
  n86 = Obtain Queue(name (unnamed)="数据1" ("名称（未命名）"), element data type="VCI_Receive") -> (queue out=w41:refnum<queue>, error out=w40:errorcluster)  [unwired: 3 in, 1 out]
  n87 = call <vilib>:"Application Directory.vi"() -> ("Application Directory"=w20:path)
  n88 = Obtain Queue(element data type="输出簇") -> (queue out=w39:refnum<queue>, error out=w33:errorcluster)  [unwired: 4 in, 1 out]
  n89 = Obtain Queue(name (unnamed)="数据2" ("名称（未命名）"), element data type=w37) -> (queue out=w43:refnum<queue>, error out=w42:errorcluster)  [unwired: 3 in, 1 out]
  n90 = local write "状态"("" ("状态")) -> ()
  n91 = case shown="假" w7 {
    tunnel: [w89 TRUE ("鉴权通过")] -> w18
    tunnel: [w88 w93] -> w11
    tunnel: [w87 w92] -> w10
    tunnel: [w86 w91] -> w9
    tunnel: [w85 w90] -> w8
    tunnel: w6 -> [w84 _]
    tunnel: w5 -> [w83 _]
    tunnel: w4 -> [_ w93]
    tunnel: w3 -> [_ w92]
    tunnel: w2 -> [_ w91]
    tunnel: w1 -> [_ w90]
    frame False {
      n92 = call-by-ref "?"("机器码 2"=w84, "注册码 2"=w83) -> ("鉴权通过"=w89:bool, "参数配置"=w88:bool, "参数生成"=w87:bool, "强制操作"=w86:bool, "数据保存"=w85:bool)  [unwired: 11 in, 2 out]
    }
    frame True {
    }
  }
  "参数配置" <- w11
  "参数生成" <- w10
  "强制操作" <- w9
  "数据保存" <- w8
  n93 = Build Path(base path=w20, name or relative path="History Data\\" ("名称或相对路径")) -> (appended path=w27:path)
  n94 = call "自适应屏幕分辨率.vi"() -> ()  [unwired: 16 in]
  n95 = call <vilib>:"Check if File or Folder Exists.vi"("error in (no error)"=errorcluster {"status"=FALSE, "code"=0, "source"=""}, "path"=w27) -> ("error out"=w25:errorcluster, "file or folder exists?"=w28:bool, "dup path"=w26:path)  [unwired: 7 in]
  n96 = property on="电池系统绝缘状态" class="Str"("Visible"=FALSE ("可见")) -> ()  [unwired: 2 in, 2 out]
  n97 = case shown="假" w28 {
    tunnel: w26 -> [w95 _]
    frame False {
      n98 = Create Folder(path (use dialog)=w95) -> ()  [unwired: 2 in, 3 out]
    }
    frame True {
    }
  }
  n99 = local write "外总压"(w23) -> ()
  n100 = local write "平均电流"(w23) -> ()
  n101 = local write "Life"("0" ("Life")) -> ()
  n102 = local write "BMS供电电压"(w23) -> ()
  n103 = local write "从板个数"(w23) -> ()
  n104 = case shown="真" w18 {
    tunnel: w43 -> [_ w121]
    tunnel: w42 -> [_ w120]
    tunnel: w41 -> [_ w114]
    tunnel: w40 -> [_ w113]
    tunnel: w39 -> [_ w112]
    tunnel: w33 -> [_ w106]
    tunnel: w26 -> [_ w105]
    tunnel: w25 -> [_ w104]
    tunnel: w12 -> [_ w101]
    frame False {
      n105 = disable-structure shown="RUN_TIME_ENGINE==True" {
        frame condition #0 (active) {
        }
        frame condition #1 {
          n106 = Quit LabVIEW(quit? (T)=TRUE ("退出？(T)")) -> ()
        }
      }
    }
    frame True {
      w108 = TRUE ("强制销毁？(F)")
      # "历史数据保存:\n1.数据保存：判定用户数据保存权限\n2.CAN初始化成功：CAN连接成功后允许数据保存\n3.允许保存数据：点击刷新后5秒内不保存数据控制\n4.开始保存：CAN连接成功5秒后开始保存数据控制"
      n107 = invoke class="VI" method="FP.Open"(reference=w101, "Activate"=TRUE ("激活？"), "State"=T10."Standard" ("状态")) -> ()  [unwired: 2 in, 5 out]
      n108 = local read "数据保存"() -> (w98:bool)
      n109 = case shown="真" w98 {
        tunnel: w105 -> [_ w129]
        tunnel: w104 -> [_ w128]
        frame False {
        }
        frame True {
          # "每点一次刷新后，停止保存数据5S，5S后继续运行"
          n110 = while {
            tunnel: w128 -> [w144]
            tunnel: w129 -> [w145]
            tunnel: [w143] -> _
            stop <- w130 stop-if-true
            # "计算保存BMU个数"
            n111 = local read "开始保存"() -> (w135:bool)
            n112 = local read "开始保存"() -> (w136:bool)
            n113 = local read "CAN初始化成功"() -> (w133:bool)
            n114 = global read "电池信息全局变量.vi" "允许保存数据"() -> (w131:bool)
            n115 = global read "从板全局变量.vi" "电池节数"() -> (w139:u8[])
            n116 = Not(x=w135) -> (.not. x?=w134:bool)
            n117 = Compound Arithmetic op=AND(w134, w133) -> (w132:bool)
            n118 = for {
              tunnel: w139 -> [w152] mode=indexing
              shift-right: [w148] -> w140
              shift-left: 0 -> [w149]
              i -> [w150]
              n119 = Not Equal To 0?(x=w152) -> (x != 0?=w151:bool)
              n120 = Select(t=w150, s=w151, f=w149) -> (s? t:f=w148:i32)
            }
            n121 = case shown="真" w132 {
              frame False {
              }
              frame True {
                n122 = stacked-sequence {
                  frame #0 {
                    n123 = Wait (ms)(milliseconds to wait=u32 5000 ("等待时间（毫秒）")) -> ()  [unwired: 1 out]
                  }
                  frame #1 {
                    n124 = local write "开始保存"(TRUE ("开始保存")) -> ()
                  }
                }
              }
            }
            n125 = Compound Arithmetic op=AND(w136, w133, w131) -> (w142:bool)
            n126 = Increment(x=w140) -> (x+1=w137:i32)
            n127 = case shown="真" w142 {
              tunnel: w145 -> [_ w170]
              tunnel: w144 -> [w164 w169]
              tunnel: [w164 w168] -> w143
              tunnel: w137 -> [_ w165]
              frame False {
                n128 = Wait (ms)(milliseconds to wait=u32 10 ("等待时间（毫秒）")) -> ()  [unwired: 1 out]
              }
              frame True {
                n129 = local read "dup path"() -> (w166:path)
                n130 = Empty String/Path?(string/path=w166) -> (empty?=w167:bool)
                n131 = case shown="假" w167 {
                  tunnel: w170 -> [_ w202]
                  tunnel: w166 -> [w175 _]
                  tunnel: w169 -> [w177 w199]
                  tunnel: [w176 w200] -> w168
                  tunnel: w165 -> [w171 w197]
                  frame False {
                    n132 = Get File Size(file=w175) -> (size (in bytes)=w174:i64)  [unwired: 1 in, 2 out]
                    n133 = Greater Or Equal?(x=w174, y=i64 30000000) -> (x >= y?=w172:bool)
                    n134 = case shown="真" w172 {
                      tunnel: w175 -> [w181 w196]
                      tunnel: w177 -> [w180 w182]
                      tunnel: [w179 w187] -> w176
                      tunnel: w171 -> [w178 w183]
                      frame False {
                        n135 = call-by-ref "?"("error in (no error)"=w180, "dup path"=w181, "从板个数"=w178) -> ("error out"=w179:errorcluster)  [unwired: 10 in, 2 out]
                      }
                      frame True {
                        n136 = local read "文件序号"() -> (w185:u32)
                        n137 = Path To String(path=w196) -> (string=w193:string)
                        n138 = Increment(x=w185) -> (x+1=w184:u32)
                        n139 = Number To Decimal String(number=w184) -> (decimal integer string=w192:string)  [unwired: 1 in]
                        n140 = local write "文件序号"(w184) -> ()
                        n141 = Concatenate Strings("_" ("字符串"), w192, ".csv" ("替换字符串(\"\")")) -> (w189:string)
                        n142 = Search and Replace String(replace all?=TRUE ("替换全部？(F)"), input string=w193, search string=".csv" ("搜索字符串"), replace string=w189) -> (result string=w188:string)  [unwired: 4 in, 3 out]
                        n143 = String To Path(string=w188) -> (path=w186:path)
                        n144 = local write "dup path"(w186) -> ()
                        n145 = call-by-ref "?"("error in (no error)"=w182, "file path"=w186, "从板数"=w183) -> ("error out"=w187:errorcluster)  [unwired: 10 in, 2 out]
                      }
                    }
                  }
                  frame True {
                    n146 = Get Date/Time String(date format (0)=enum16{"short", "long", "abbreviated"}."abbreviated" ("日期格式(0)"), want seconds? (F)=TRUE ("需要秒？(F)")) -> (date string=w207:string, time string=w206:string)  [unwired: 1 in]
                    n147 = Concatenate Strings(w207, w206) -> (w210:string)
                    n148 = local write "文件序号"(u32 0 ("文件序号")) -> ()
                    n149 = Search and Replace String(replace all?=TRUE ("替换全部？(F)"), input string=w210, search string=":" ("搜索字符串"), replace string="_" ("替换字符串(\"\")")) -> (result string=w205:string)  [unwired: 4 in, 3 out]
                    n150 = Concatenate Strings(w205, ".csv" ("字符串")) -> (w203:string)
                    n151 = Build Path(base path=w202, name or relative path=w203) -> (appended path=w201:path)
                    n152 = local write "dup path"(w201) -> ()
                    n153 = call "Create Title For CSV.vi"("error in (no error)"=w199, "file path"=w201, "从板数"=w197) -> ("error out"=w200:errorcluster)  [unwired: 8 in]
                  }
                }
              }
            }
            n154 = disable-structure shown="禁用" {
              frame Disabled {
                n155 = case shown="\"0.2\"" "保存间隔(S)" {
                  tunnel: [500 400 300 200 100 1000 2000 3000 4000] -> _
                  frame "0.5", Default {
                  }
                  frame "0.4" {
                  }
                  frame "0.3" {
                  }
                  frame "0.2" {
                  }
                  frame "0.1" {
                  }
                  frame "1" {
                  }
                  frame "2" {
                  }
                  frame "3" {
                  }
                  frame "4" {
                  }
                }
              }
              frame Enabled {
              }
            }
            n156 = Wait (ms)(milliseconds to wait=u32 1000 ("等待时间（毫秒）")) -> ()  [unwired: 1 out]
            n157 = local read "退出"() -> (w130:bool)
          }
        }
      }
      n158 = while {
        tunnel: [w1550] -> w97
        stop <- w1550 stop-if-true
        n159 = event shown="[24] \"诊断标定\", \"诊断标定 3\": 值改变" {
          selector: _ -> [_ _ _ _ _ _ _ _ _ _ _ _ _ _ _ _ _ _ _ _ _ _ _ _ _ _ _]
          dyn-events: _ -> [_ _ _ _ _ _ _ _ _ _ _ _ _ _ _ _ _ _ _ _ _ _ _ _ _ _ _]
          timeout: 200 -> [_ _ _ _ _ _ _ _ _ _ _ _ _ _ _ _ _ _ _ _ _ _ _ _ _ _ _]
          tunnel: [_ _ _ _ _ _ _ _ _ _ _ _ _ _ _ _ _ _ _ _ _ _ _ _ _ w2485 w2494] -> w1550
          event "中英文选择": Value Change {
            n160 = event-data() -> ("NewVal"=w1552:enum32{"中文", "English"})  [unwired: 6 out]
            n161 = disable-structure shown="禁用" {
              disable-tunnel: w1552 -> [w1575 _]
              frame Disabled {
                n162 = global read "功能码全局.vi" "14"() -> (w1566:bool[])
                n163 = local read "数值"() -> (w1557:i32)
                n164 = control-ref of="负级继电器"() -> (w1595:refnum<vi>)
                n165 = control-ref of="充电继电器"() -> (w1593:refnum<vi>)
                n166 = control-ref of="正级继电器"() -> (w1596:refnum<vi>)
                n167 = control-ref of="预充继电器"() -> (w1594:refnum<vi>)
                n168 = Greater?(x=w1557, y=0) -> (0:w1565:bool)
                n169 = Index Array(array=w1566, index=6 ("索引")) -> (element=w1563:bool)
                n170 = And(x=w1565, y=w1563) -> (x .and. y?=w1564:bool)
                n171 = case shown="\"English\"" w1575 {
                  tunnel: [TRUE FALSE] -> w1574
                  tunnel: [FALSE TRUE] -> w1573
                  tunnel: [string[] ["正极继电器", "负极继电器", "预充电继电器", "充电继电器"] ("字符串[]") string[] ["POS_RLY", "NEG_RLY", "PRE_RLY", "CHG_RLY"] ("字符串[]")] -> w1598
                  tunnel: [string[] ["未闭合", "闭合", "故障", "保留"] ("字符串[]") string[] ["OPEN", "CLOSE", "ERROR", "RSV"] ("字符串[]")] -> w1597
                  tunnel: ["故障信息概况" ("标题.文本") "Fault_Survey" ("标题.文本")] -> w1591
                  tunnel: ["无故障" ("标题.文本") "NO_Fault" ("标题.文本")] -> w1590
                  tunnel: ["电池系统绝缘状态" ("标题.文本") "ISO_Status" ("标题.文本")] -> w1589
                  tunnel: ["中间侧" ("标题.文本") "ISO_MID" ("标题.文本")] -> w1588
                  tunnel: ["BMS时钟" ("标题.文本") "BMS_Timer" ("标题.文本")] -> w1587
                  tunnel: ["电池系统初始检测" ("标题.文本") "Start_Test" ("标题.文本")] -> w1586
                  tunnel: ["系统运行模式" ("标题.文本") "Run_Mode" ("标题.文本")] -> w1585
                  tunnel: [string[] ["次要参数", "单体电压", "单体温度", "单体内阻", "参数曲线"] ("字符串[]") string[] ["Parameter_1", "Cells", "Temp", "Bat", "Parameter_2"] ("字符串[]")] -> w1583
                  tunnel: ["状态" ("标题.文本") "Status" ("标题.文本")] -> w1582
                  tunnel: [string[] ["最高单体电压", "最高电压位置", "最低单体电压", "最低电压位置", "压差", "最高单体温度", "最高温度位置", "最低单体温度", "最低温度位置", "温差", "最高单体内阻", "最高内阻位置", "最低单体内阻", "最低内阻位置", "总内阻", "协议是否公开", "协议版本号", "应用类型", "波特率"] ("字符串[]") string[] ["MaxV(V)", "MaxV_No.", "MinV(V)", "MinV_No.", "DiffV", "MaxT(℃)", "MaxT_No.", "MinT(℃)", "MinT_No.", "DiffT", "Max_Bat", "Max_Bat_No.", "Min_Bat", "Min_Bat_No.", "Total_Bat", "Protocol_Open", "Protocol_Ver", "Application_Type", "Baudrate"] ("字符串[]")] -> w1579
                  tunnel: ["总电压(V)" ("标题.文本") "SumV(V)" ("标题.文本")] -> w1577
                  tunnel: ["总电流(A)" ("标题.文本") "SumCurr(A)" ("标题.文本")] -> w1576
                  tunnel: w1564 -> [w1607 w1627]
                  tunnel: ["暂停" ("标题.文本") "Pause" ("标题.文本")] -> w1554
                  tunnel: ["幅值" ("标题.文本") "Amp" ("标题.文本")] -> w1553
                  frame "中文", Default {
                    n172 = Not(x=w1607) -> (.not. x?=w1606:bool)
                    n173 = property on="单箱信息" class="Bool (严格)"("Visible"=w1607) -> ()  [unwired: 2 in, 2 out]
                    n174 = property on="单板信息 3" class="Bool (严格)"("Visible"=w1606) -> ()  [unwired: 2 in, 2 out]
                  }
                  frame "English" {
                    (unwired) "Pause" ("标题.文本")
                    n175 = Not(x=w1627) -> (.not. x?=w1626:bool)
                    n176 = property on="单板信息 3" class="Bool (严格)"("Visible"=w1627) -> ()  [unwired: 2 in, 2 out]
                    n177 = property on="单箱信息" class="Bool (严格)"("Visible"=w1626) -> ()  [unwired: 2 in, 2 out]
                  }
                }
                n178 = control-ref of="次要参数"() -> (w1581:refnum<vi>)
                n179 = global write "全局 1.vi" "中英文选择"(w1575) -> ()
                n180 = control-ref of="总信息卡"() -> (w1572:refnum<vi>)
                n181 = control-ref of="单体电压卡"() -> (w1571:refnum<vi>)
                n182 = control-ref of="单体温度卡"() -> (w1570:refnum<vi>)
                n183 = control-ref of="单选选项2 4"() -> (w1569:refnum<vi>)
                n184 = Build Array(w1596, w1595, w1594, w1593) -> (w1592:refnum<vi>[])
                n185 = control-ref of="单选选项2 5"() -> (w1568:refnum<vi>)
                n186 = property class="Clust (严格)"(reference=w1581) -> ("Controls[]"=w1580:refnum<vi>[])  [unwired: 1 in, 2 out]
                n187 = for {
                  tunnel: w1598 -> [w1605] mode=indexing
                  tunnel: w1597 -> [w1604]
                  tunnel: w1592 -> [w1603] mode=indexing
                  n188 = property class="Ring (严格)"(reference=w1603, "Caption.Text"=w1605, "Strings []"=w1604) -> ()  [unwired: 1 in, 2 out]
                }
                n189 = Build Array(w1572, w1571, w1570, w1569, w1568) -> (w1584:refnum<vi>[])
                n190 = local read "中英文选择"() -> (w1555:enum32{"中文", "English"})
                n191 = for {
                  tunnel: w1584 -> [w1602] mode=indexing
                  tunnel: w1583 -> [w1601] mode=indexing
                  n192 = property class="Bool (严格)"(reference=w1602, "BoolText.Text"=w1601) -> ()  [unwired: 1 in, 2 out]
                }
                n193 = for {
                  tunnel: w1580 -> [w1600] mode=indexing
                  tunnel: w1579 -> [w1599] mode=indexing
                  n194 = property class="Ctl"(reference=w1600, "Caption.Text"=w1599) -> ()  [unwired: 1 in, 2 out]
                }
                n195 = global write "中英文全局.vi" "中英文选择"(w1555) -> ()
                n196 = property on="故障信息概况" class="Str"("Caption.Text"=w1591, "Text.Text"=w1590) -> ()  [unwired: 2 in, 2 out]
                n197 = property on="详细信息 3" class="Bool (严格)"("Visible"=w1573) -> ()  [unwired: 2 in, 2 out]
                n198 = property on="诊断标定 3" class="Bool (严格)"("Visible"=w1573) -> ()  [unwired: 2 in, 2 out]
                n199 = property on="界面刷新 2" class="Bool (严格)"("Visible"=w1573) -> ()  [unwired: 2 in, 2 out]
                n200 = global read "功能码全局.vi" "主板监控预留1"() -> (w1561:bool[])
                n201 = property on="详细信息 4" class="Bool (严格)"("Visible"=w1573) -> ()  [unwired: 2 in, 2 out]
                n202 = property on="启动CAN 2" class="Bool (严格)"("Visible"=w1573) -> ()  [unwired: 2 in, 2 out]
                n203 = property on="参数设置 2" class="Bool (严格)"("Visible"=w1573) -> ()  [unwired: 2 in, 2 out]
                n204 = property on="退出 2" class="Bool (严格)"("Visible"=w1573) -> ()  [unwired: 2 in, 2 out]
                n205 = property on="帮助 2" class="Bool (严格)"("Visible"=w1573) -> ()  [unwired: 2 in, 2 out]
                n206 = property on="状态" class="Str"("Caption.Text"=w1582) -> ()  [unwired: 2 in, 2 out]
                n207 = property on="电池系统绝缘状态" class="Str"("Caption.Text"=w1589, "Text.Text"=w1588) -> ()  [unwired: 2 in, 2 out]
                n208 = property on="系统运行模式" class="Str"("Caption.Text"=w1585, "Text.Text"=w1586) -> ()  [unwired: 2 in, 2 out]
                n209 = property on="BMS时间" class="Str"("Caption.Text"=w1587) -> ()  [unwired: 2 in, 2 out]
                n210 = property on="总电压(V)" class="DigNum (严格)"("Caption.Text"=w1577) -> ()  [unwired: 2 in, 2 out]
                n211 = property on="总电流(A)" class="DigNum (严格)"("Caption.Text"=w1576) -> ()  [unwired: 2 in, 2 out]
                n212 = Index Array(array=w1561, index=7 ("索引")) -> (element=w1558:bool)
                n213 = property on="系统信息" class="Bool (严格)"("Visible"=w1574) -> ()  [unwired: 2 in, 2 out]
                n214 = property on="CAN连接" class="Bool (严格)"("Visible"=w1574) -> ()  [unwired: 2 in, 2 out]
                n215 = property on="电压温度" class="Bool (严格)"("Visible"=w1574) -> ()  [unwired: 2 in, 2 out]
                n216 = property on="帮助" class="Bool (严格)"("Visible"=w1574) -> ()  [unwired: 2 in, 2 out]
                n217 = property on="退出" class="Bool (严格)"("Visible"=w1574) -> ()  [unwired: 2 in, 2 out]
                n218 = property on="参数设置" class="Bool (严格)"("Visible"=w1574) -> ()  [unwired: 2 in, 2 out]
                n219 = property on="诊断标定" class="Bool (严格)"("Visible"=w1574) -> ()  [unwired: 2 in, 2 out]
                n220 = property on="数据刷新" class="Bool (严格)"("Visible"=w1574) -> ()  [unwired: 2 in, 2 out]
                n221 = property on="System XY Graph" class="XYGraph (严格)"("YScale.NameLbl.Text"=w1553) -> ()  [unwired: 2 in, 2 out]
                n222 = And(x=w1574, y=w1558) -> (x .and. y?=w1560:bool)
                n223 = property on="暂停 3" class="Bool (严格)"("Caption.Text"=w1554) -> ()  [unwired: 2 in, 2 out]
                n224 = And(x=w1573, y=w1558) -> (x .and. y?=w1559:bool)
                n225 = property on="保存数据 2" class="Bool (严格)"("Visible"=w1559) -> ()  [unwired: 2 in, 2 out]
                n226 = property on="保存数据 3" class="Bool (严格)"("Visible"=w1560) -> ()  [unwired: 2 in, 2 out]
                n227 = local write "状态"(" " ("状态")) -> ()
              }
              frame Enabled {
              }
            }
          }
          event "界面刷新 2", "数据刷新": Value Change {
            n228 = event-data() -> ("NewVal"=w1646:bool)  [unwired: 6 out]
            n229 = case shown="真" w1646 {
              frame False {
              }
              frame True {
                w1653 = 0.0 ("CC")
                w1654 = FALSE ("DI3")
                w1655 = 0.0 ("外总压")
                w1656 = u16 0 ("总电压进度")
                w1658 = "" ("BMS时间")
                w1659 = 0.0 ("总电压")
                n230 = global write "电池信息全局变量.vi" "允许保存数据"(FALSE ("允许保存数据")) -> ()
                n231 = local write "总电压(V)"(w1659) -> ()
                n232 = local write "总电流(A)"(w1659) -> ()
                n233 = local write "SOH"(w1659) -> ()
                n234 = local write "SOC"(w1659) -> ()
                n235 = global write "电池信息全局变量.vi" "刷新计数"(0.0 ("刷新计数")) -> ()
                n236 = local write "SOC(黄)"(w1659) -> ()
                n237 = local write "SOC(红)"(w1659) -> ()
                n238 = local write "充电继电器"(w1659) -> ()
                n239 = local write "正级继电器"(w1659) -> ()
                n240 = local write "负级继电器"(w1659) -> ()
                n241 = global write "从板全局变量.vi" "电池节数"(u8[] [0, 0, 0, 0, 0, 0, 0, 0, 0, 0, 0, 0, 0, 0, 0, 0, 0, 0, 0, 0, 0, 0, 0, 0, 0, 0, 0, 0, 0, 0] ("电池节数")) -> ()
                n242 = global write "从板全局变量.vi" "温度个数"(u8[] [0, 0, 0, 0, 0, 0, 0, 0, 0, 0, 0, 0, 0, 0, 0, 0, 0, 0, 0, 0, 0, 0, 0, 0, 0, 0, 0, 0, 0, 0] ("温度个数")) -> ()
                n243 = global write "单体信息全局.vi" "单体数据"(dbl[][] [[0.0, 0.0, 0.0, 0.0, 0.0, 0.0, 0.0, 0.0, 0.0, 0.0, 0.0, 0.0, 0.0, 0.0, 0.0, 0.0, 0.0, 0.0, 0.0, 0.0, 0.0, 0.0, 0.0, 0.0, 0.0, 0.0, 0.0, 0.0, 0.0, 0.0, 0.0, 0.0, 0.0, 0.0, 0.0, 0.0, 0.0, 0.0, 0.0, 0.0, 0.0, 0.0, 0.0, 0.0, 0.0, 0.0, 0.0, 0.0, 0.0, 0.0, 0.0, 0.0, 0.0, 0.0, 0.0, 0.0, 0.0, 0.0, 0.0, 0.0, 0.0], [0.0, 0.0, 0.0, 0.0, 0.0, 0.0, 0.0, 0.0, 0.0, 0.0, 0.0, 0.0, 0.0, 0.0, 0.0, 0.0, 0.0, 0.0, 0.0, 0.0, 0.0, 0.0, 0.0, 0.0, 0.0, 0.0, 0.0, 0.0, 0.0, 0.0, 0.0, 0.0, 0.0, 0.0, 0.0, 0.0, 0.0, 0.0, 0.0, 0.0, 0.0, 0.0, 0.0, 0.0, 0.0, 0.0, 0.0, 0.0, 0.0, 0.0, 0.0, 0.0, 0.0, 0.0, 0.0, 0.0, 0.0, 0.0, 0.0, 0.0, 0.0], [0.0, 0.0, 0.0, 0.0, 0.0, 0.0, 0.0, 0.0, 0.0, 0.0, 0.0, 0.0, 0.0, 0.0, 0.0, 0.0, 0.0, 0.0, 0.0, 0.0, 0.0, 0.0, 0.0, 0.0, 0.0, 0.0, 0.0, 0.0, 0.0, 0.0, 0.0, 0.0, 0.0, 0.0, 0.0, 0.0, 0.0, 0.0, 0.0, 0.0, 0.0, 0.0, 0.0, 0.0, 0.0, 0.0, 0.0, 0.0, 0.0, 0.0, 0.0, 0.0, 0.0, 0.0, 0.0, 0.0, 0.0, 0.0, 0.0, 0.0, 0.0], [0.0, 0.0, 0.0, 0.0, 0.0, 0.0, 0.0, 0.0, 0.0, 0.0, 0.0, 0.0, 0.0, 0.0, 0.0, 0.0, 0.0, 0.0, 0.0, 0.0, 0.0, 0.0, 0.0, 0.0, 0.0, 0.0, 0.0, 0.0, 0.0, 0.0, 0.0, 0.0, 0.0, 0.0, 0.0, 0.0, 0.0, 0.0, 0.0, 0.0, 0.0, 0.0, 0.0, 0.0, 0.0, 0.0, 0.0, 0.0, 0.0, 0.0, 0.0, 0.0, 0.0, 0.0, 0.0, 0.0, 0.0, 0.0, 0.0, 0.0, 0.0], [0.0, 0.0, 0.0, 0.0, 0.0, 0.0, 0.0, 0.0, 0.0, 0.0, 0.0, 0.0, 0.0, 0.0, 0.0, 0.0, 0.0, 0.0, 0.0, 0.0, 0.0, 0.0, 0.0, 0.0, 0.0, 0.0, 0.0, 0.0, 0.0, 0.0, 0.0, 0.0, 0.0, 0.0, 0.0, 0.0, 0.0, 0.0, 0.0, 0.0, 0.0, 0.0, 0.0, 0.0, 0.0, 0.0, 0.0, 0.0, 0.0, 0.0, 0.0, 0.0, 0.0, 0.0, 0.0, 0.0, 0.0, 0.0, 0.0, 0.0, 0.0], [0.0, 0.0, 0.0, 0.0, 0.0, 0.0, 0.0, 0.0, 0.0, 0.0, 0.0, 0.0, 0.0, 0.0, 0.0, 0.0, 0.0, 0.0, 0.0, 0.0, 0.0, 0.0, 0.0, 0.0, 0.0, 0.0, 0.0, 0.0, 0.0, 0.0, 0.0, 0.0, 0.0, 0.0, 0.0, 0.0, 0.0, 0.0, 0.0, 0.0, 0.0, 0.0, 0.0, 0.0, 0.0, 0.0, 0.0, 0.0, 0.0, 0.0, 0.0, 0.0, 0.0, 0.0, 0.0, 0.0, 0.0, 0.0, 0.0, 0.0, 0.0], [0.0, 0.0, 0.0, 0.0, 0.0, 0.0, 0.0, 0.0, 0.0, 0.0, 0.0, 0.0, 0.0, 0.0, 0.0, 0.0, 0.0, 0.0, 0.0, 0.0, 0.0, 0.0, 0.0, 0.0, 0.0, 0.0, 0.0, 0.0, 0.0, 0.0, 0.0, 0.0, 0.0, 0.0, 0.0, 0.0, 0.0, 0.0, 0.0, 0.0, 0.0, 0.0, 0.0, 0.0, 0.0, 0.0, 0.0, 0.0, 0.0, 0.0, 0.0, 0.0, 0.0, 0.0, 0.0, 0.0, 0.0, 0.0, 0.0, 0.0, 0.0], [0.0, 0.0, 0.0, 0.0, 0.0, 0.0, 0.0, 0.0, 0.0, 0.0, 0.0, 0.0, 0.0, 0.0, 0.0, 0.0, 0.0, 0.0, 0.0, 0.0, 0.0, 0.0, 0.0, 0.0, 0.0, 0.0, 0.0, 0.0, 0.0, 0.0, 0.0, 0.0, 0.0, 0.0, 0.0, 0.0, 0.0, 0.0, 0.0, 0.0, 0.0, 0.0, 0.0, 0.0, 0.0, 0.0, 0.0, 0.0, 0.0, 0.0, 0.0, 0.0, 0.0, 0.0, 0.0, 0.0, 0.0, 0.0, 0.0, 0.0, 0.0], [0.0, 0.0, 0.0, 0.0, 0.0, 0.0, 0.0, 0.0, 0.0, 0.0, 0.0, 0.0, 0.0, 0.0, 0.0, 0.0, 0.0, 0.0, 0.0, 0.0, 0.0, 0.0, 0.0, 0.0, 0.0, 0.0, 0.0, 0.0, 0.0, 0.0, 0.0, 0.0, 0.0, 0.0, 0.0, 0.0, 0.0, 0.0, 0.0, 0.0, 0.0, 0.0, 0.0, 0.0, 0.0, 0.0, 0.0, 0.0, 0.0, 0.0, 0.0, 0.0, 0.0, 0.0, 0.0, 0.0, 0.0, 0.0, 0.0, 0.0, 0.0], [0.0, 0.0, 0.0, 0.0, 0.0, 0.0, 0.0, 0.0, 0.0, 0.0, 0.0, 0.0, 0.0, 0.0, 0.0, 0.0, 0.0, 0.0, 0.0, 0.0, 0.0, 0.0, 0.0, 0.0, 0.0, 0.0, 0.0, 0.0, 0.0, 0.0, 0.0, 0.0, 0.0, 0.0, 0.0, 0.0, 0.0, 0.0, 0.0, 0.0, 0.0, 0.0, 0.0, 0.0, 0.0, 0.0, 0.0, 0.0, 0.0, 0.0, 0.0, 0.0, 0.0, 0.0, 0.0, 0.0, 0.0, 0.0, 0.0, 0.0, 0.0], [0.0, 0.0, 0.0, 0.0, 0.0, 0.0, 0.0, 0.0, 0.0, 0.0, 0.0, 0.0, 0.0, 0.0, 0.0, 0.0, 0.0, 0.0, 0.0, 0.0, 0.0, 0.0, 0.0, 0.0, 0.0, 0.0, 0.0, 0.0, 0.0, 0.0, 0.0, 0.0, 0.0, 0.0, 0.0, 0.0, 0.0, 0.0, 0.0, 0.0, 0.0, 0.0, 0.0, 0.0, 0.0, 0.0, 0.0, 0.0, 0.0, 0.0, 0.0, 0.0, 0.0, 0.0, 0.0, 0.0, 0.0, 0.0, 0.0, 0.0, 0.0], [0.0, 0.0, 0.0, 0.0, 0.0, 0.0, 0.0, 0.0, 0.0, 0.0, 0.0, 0.0, 0.0, 0.0, 0.0, 0.0, 0.0, 0.0, 0.0, 0.0, 0.0, 0.0, 0.0, 0.0, 0.0, 0.0, 0.0, 0.0, 0.0, 0.0, 0.0, 0.0, 0.0, 0.0, 0.0, 0.0, 0.0, 0.0, 0.0, 0.0, 0.0, 0.0, 0.0, 0.0, 0.0, 0.0, 0.0, 0.0, 0.0, 0.0, 0.0, 0.0, 0.0, 0.0, 0.0, 0.0, 0.0, 0.0, 0.0, 0.0, 0.0], [0.0, 0.0, 0.0, 0.0, 0.0, 0.0, 0.0, 0.0, 0.0, 0.0, 0.0, 0.0, 0.0, 0.0, 0.0, 0.0, 0.0, 0.0, 0.0, 0.0, 0.0, 0.0, 0.0, 0.0, 0.0, 0.0, 0.0, 0.0, 0.0, 0.0, 0.0, 0.0, 0.0, 0.0, 0.0, 0.0, 0.0, 0.0, 0.0, 0.0, 0.0, 0.0, 0.0, 0.0, 0.0, 0.0, 0.0, 0.0, 0.0, 0.0, 0.0, 0.0, 0.0, 0.0, 0.0, 0.0, 0.0, 0.0, 0.0, 0.0, 0.0], [0.0, 0.0, 0.0, 0.0, 0.0, 0.0, 0.0, 0.0, 0.0, 0.0, 0.0, 0.0, 0.0, 0.0, 0.0, 0.0, 0.0, 0.0, 0.0, 0.0, 0.0, 0.0, 0.0, 0.0, 0.0, 0.0, 0.0, 0.0, 0.0, 0.0, 0.0, 0.0, 0.0, 0.0, 0.0, 0.0, 0.0, 0.0, 0.0, 0.0, 0.0, 0.0, 0.0, 0.0, 0.0, 0.0, 0.0, 0.0, 0.0, 0.0, 0.0, 0.0, 0.0, 0.0, 0.0, 0.0, 0.0, 0.0, 0.0, 0.0, 0.0], [0.0, 0.0, 0.0, 0.0, 0.0, 0.0, 0.0, 0.0, 0.0, 0.0, 0.0, 0.0, 0.0, 0.0, 0.0, 0.0, 0.0, 0.0, 0.0, 0.0, 0.0, 0.0, 0.0, 0.0, 0.0, 0.0, 0.0, 0.0, 0.0, 0.0, 0.0, 0.0, 0.0, 0.0, 0.0, 0.0, 0.0, 0.0, 0.0, 0.0, 0.0, 0.0, 0.0, 0.0, 0.0, 0.0, 0.0, 0.0, 0.0, 0.0, 0.0, 0.0, 0.0, 0.0, 0.0, 0.0, 0.0, 0.0, 0.0, 0.0, 0.0], [0.0, 0.0, 0.0, 0.0, 0.0, 0.0, 0.0, 0.0, 0.0, 0.0, 0.0, 0.0, 0.0, 0.0, 0.0, 0.0, 0.0, 0.0, 0.0, 0.0, 0.0, 0.0, 0.0, 0.0, 0.0, 0.0, 0.0, 0.0, 0.0, 0.0, 0.0, 0.0, 0.0, 0.0, 0.0, 0.0, 0.0, 0.0, 0.0, 0.0, 0.0, 0.0, 0.0, 0.0, 0.0, 0.0, 0.0, 0.0, 0.0, 0.0, 0.0, 0.0, 0.0, 0.0, 0.0, 0.0, 0.0, 0.0, 0.0, 0.0, 0.0], [0.0, 0.0, 0.0, 0.0, 0.0, 0.0, 0.0, 0.0, 0.0, 0.0, 0.0, 0.0, 0.0, 0.0, 0.0, 0.0, 0.0, 0.0, 0.0, 0.0, 0.0, 0.0, 0.0, 0.0, 0.0, 0.0, 0.0, 0.0, 0.0, 0.0, 0.0, 0.0, 0.0, 0.0, 0.0, 0.0, 0.0, 0.0, 0.0, 0.0, 0.0, 0.0, 0.0, 0.0, 0.0, 0.0, 0.0, 0.0, 0.0, 0.0, 0.0, 0.0, 0.0, 0.0, 0.0, 0.0, 0.0, 0.0, 0.0, 0.0, 0.0], [0.0, 0.0, 0.0, 0.0, 0.0, 0.0, 0.0, 0.0, 0.0, 0.0, 0.0, 0.0, 0.0, 0.0, 0.0, 0.0, 0.0, 0.0, 0.0, 0.0, 0.0, 0.0, 0.0, 0.0, 0.0, 0.0, 0.0, 0.0, 0.0, 0.0, 0.0, 0.0, 0.0, 0.0, 0.0, 0.0, 0.0, 0.0, 0.0, 0.0, 0.0, 0.0, 0.0, 0.0, 0.0, 0.0, 0.0, 0.0, 0.0, 0.0, 0.0, 0.0, 0.0, 0.0, 0.0, 0.0, 0.0, 0.0, 0.0, 0.0, 0.0], [0.0, 0.0, 0.0, 0.0, 0.0, 0.0, 0.0, 0.0, 0.0, 0.0, 0.0, 0.0, 0.0, 0.0, 0.0, 0.0, 0.0, 0.0, 0.0, 0.0, 0.0, 0.0, 0.0, 0.0, 0.0, 0.0, 0.0, 0.0, 0.0, 0.0, 0.0, 0.0, 0.0, 0.0, 0.0, 0.0, 0.0, 0.0, 0.0, 0.0, 0.0, 0.0, 0.0, 0.0, 0.0, 0.0, 0.0, 0.0, 0.0, 0.0, 0.0, 0.0, 0.0, 0.0, 0.0, 0.0, 0.0, 0.0, 0.0, 0.0, 0.0], [0.0, 0.0, 0.0, 0.0, 0.0, 0.0, 0.0, 0.0, 0.0, 0.0, 0.0, 0.0, 0.0, 0.0, 0.0, 0.0, 0.0, 0.0, 0.0, 0.0, 0.0, 0.0, 0.0, 0.0, 0.0, 0.0, 0.0, 0.0, 0.0, 0.0, 0.0, 0.0, 0.0, 0.0, 0.0, 0.0, 0.0, 0.0, 0.0, 0.0, 0.0, 0.0, 0.0, 0.0, 0.0, 0.0, 0.0, 0.0, 0.0, 0.0, 0.0, 0.0, 0.0, 0.0, 0.0, 0.0, 0.0, 0.0, 0.0, 0.0, 0.0], [0.0, 0.0, 0.0, 0.0, 0.0, 0.0, 0.0, 0.0, 0.0, 0.0, 0.0, 0.0, 0.0, 0.0, 0.0, 0.0, 0.0, 0.0, 0.0, 0.0, 0.0, 0.0, 0.0, 0.0, 0.0, 0.0, 0.0, 0.0, 0.0, 0.0, 0.0, 0.0, 0.0, 0.0, 0.0, 0.0, 0.0, 0.0, 0.0, 0.0, 0.0, 0.0, 0.0, 0.0, 0.0, 0.0, 0.0, 0.0, 0.0, 0.0, 0.0, 0.0, 0.0, 0.0, 0.0, 0.0, 0.0, 0.0, 0.0, 0.0, 0.0], [0.0, 0.0, 0.0, 0.0, 0.0, 0.0, 0.0, 0.0, 0.0, 0.0, 0.0, 0.0, 0.0, 0.0, 0.0, 0.0, 0.0, 0.0, 0.0, 0.0, 0.0, 0.0, 0.0, 0.0, 0.0, 0.0, 0.0, 0.0, 0.0, 0.0, 0.0, 0.0, 0.0, 0.0, 0.0, 0.0, 0.0, 0.0, 0.0, 0.0, 0.0, 0.0, 0.0, 0.0, 0.0, 0.0, 0.0, 0.0, 0.0, 0.0, 0.0, 0.0, 0.0, 0.0, 0.0, 0.0, 0.0, 0.0, 0.0, 0.0, 0.0], [0.0, 0.0, 0.0, 0.0, 0.0, 0.0, 0.0, 0.0, 0.0, 0.0, 0.0, 0.0, 0.0, 0.0, 0.0, 0.0, 0.0, 0.0, 0.0, 0.0, 0.0, 0.0, 0.0, 0.0, 0.0, 0.0, 0.0, 0.0, 0.0, 0.0, 0.0, 0.0, 0.0, 0.0, 0.0, 0.0, 0.0, 0.0, 0.0, 0.0, 0.0, 0.0, 0.0, 0.0, 0.0, 0.0, 0.0, 0.0, 0.0, 0.0, 0.0, 0.0, 0.0, 0.0, 0.0, 0.0, 0.0, 0.0, 0.0, 0.0, 0.0], [0.0, 0.0, 0.0, 0.0, 0.0, 0.0, 0.0, 0.0, 0.0, 0.0, 0.0, 0.0, 0.0, 0.0, 0.0, 0.0, 0.0, 0.0, 0.0, 0.0, 0.0, 0.0, 0.0, 0.0, 0.0, 0.0, 0.0, 0.0, 0.0, 0.0, 0.0, 0.0, 0.0, 0.0, 0.0, 0.0, 0.0, 0.0, 0.0, 0.0, 0.0, 0.0, 0.0, 0.0, 0.0, 0.0, 0.0, 0.0, 0.0, 0.0, 0.0, 0.0, 0.0, 0.0, 0.0, 0.0, 0.0, 0.0, 0.0, 0.0, 0.0], [0.0, 0.0, 0.0, 0.0, 0.0, 0.0, 0.0, 0.0, 0.0, 0.0, 0.0, 0.0, 0.0, 0.0, 0.0, 0.0, 0.0, 0.0, 0.0, 0.0, 0.0, 0.0, 0.0, 0.0, 0.0, 0.0, 0.0, 0.0, 0.0, 0.0, 0.0, 0.0, 0.0, 0.0, 0.0, 0.0, 0.0, 0.0, 0.0, 0.0, 0.0, 0.0, 0.0, 0.0, 0.0, 0.0, 0.0, 0.0, 0.0, 0.0, 0.0, 0.0, 0.0, 0.0, 0.0, 0.0, 0.0, 0.0, 0.0, 0.0, 0.0], [0.0, 0.0, 0.0, 0.0, 0.0, 0.0, 0.0, 0.0, 0.0, 0.0, 0.0, 0.0, 0.0, 0.0, 0.0, 0.0, 0.0, 0.0, 0.0, 0.0, 0.0, 0.0, 0.0, 0.0, 0.0, 0.0, 0.0, 0.0, 0.0, 0.0, 0.0, 0.0, 0.0, 0.0, 0.0, 0.0, 0.0, 0.0, 0.0, 0.0, 0.0, 0.0, 0.0, 0.0, 0.0, 0.0, 0.0, 0.0, 0.0, 0.0, 0.0, 0.0, 0.0, 0.0, 0.0, 0.0, 0.0, 0.0, 0.0, 0.0, 0.0], [0.0, 0.0, 0.0, 0.0, 0.0, 0.0, 0.0, 0.0, 0.0, 0.0, 0.0, 0.0, 0.0, 0.0, 0.0, 0.0, 0.0, 0.0, 0.0, 0.0, 0.0, 0.0, 0.0, 0.0, 0.0, 0.0, 0.0, 0.0, 0.0, 0.0, 0.0, 0.0, 0.0, 0.0, 0.0, 0.0, 0.0, 0.0, 0.0, 0.0, 0.0, 0.0, 0.0, 0.0, 0.0, 0.0, 0.0, 0.0, 0.0, 0.0, 0.0, 0.0, 0.0, 0.0, 0.0, 0.0, 0.0, 0.0, 0.0, 0.0, 0.0], [0.0, 0.0, 0.0, 0.0, 0.0, 0.0, 0.0, 0.0, 0.0, 0.0, 0.0, 0.0, 0.0, 0.0, 0.0, 0.0, 0.0, 0.0, 0.0, 0.0, 0.0, 0.0, 0.0, 0.0, 0.0, 0.0, 0.0, 0.0, 0.0, 0.0, 0.0, 0.0, 0.0, 0.0, 0.0, 0.0, 0.0, 0.0, 0.0, 0.0, 0.0, 0.0, 0.0, 0.0, 0.0, 0.0, 0.0, 0.0, 0.0, 0.0, 0.0, 0.0, 0.0, 0.0, 0.0, 0.0, 0.0, 0.0, 0.0, 0.0, 0.0], [0.0, 0.0, 0.0, 0.0, 0.0, 0.0, 0.0, 0.0, 0.0, 0.0, 0.0, 0.0, 0.0, 0.0, 0.0, 0.0, 0.0, 0.0, 0.0, 0.0, 0.0, 0.0, 0.0, 0.0, 0.0, 0.0, 0.0, 0.0, 0.0, 0.0, 0.0, 0.0, 0.0, 0.0, 0.0, 0.0, 0.0, 0.0, 0.0, 0.0, 0.0, 0.0, 0.0, 0.0, 0.0, 0.0, 0.0, 0.0, 0.0, 0.0, 0.0, 0.0, 0.0, 0.0, 0.0, 0.0, 0.0, 0.0, 0.0, 0.0, 0.0], [0.0, 0.0, 0.0, 0.0, 0.0, 0.0, 0.0, 0.0, 0.0, 0.0, 0.0, 0.0, 0.0, 0.0, 0.0, 0.0, 0.0, 0.0, 0.0, 0.0, 0.0, 0.0, 0.0, 0.0, 0.0, 0.0, 0.0, 0.0, 0.0, 0.0, 0.0, 0.0, 0.0, 0.0, 0.0, 0.0, 0.0, 0.0, 0.0, 0.0, 0.0, 0.0, 0.0, 0.0, 0.0, 0.0, 0.0, 0.0, 0.0, 0.0, 0.0, 0.0, 0.0, 0.0, 0.0, 0.0, 0.0, 0.0, 0.0, 0.0, 0.0], [0.0, 0.0, 0.0, 0.0, 0.0, 0.0, 0.0, 0.0, 0.0, 0.0, 0.0, 0.0, 0.0, 0.0, 0.0, 0.0, 0.0, 0.0, 0.0, 0.0, 0.0, 0.0, 0.0, 0.0, 0.0, 0.0, 0.0, 0.0, 0.0, 0.0, 0.0, 0.0, 0.0, 0.0, 0.0, 0.0, 0.0, 0.0, 0.0, 0.0, 0.0, 0.0, 0.0, 0.0, 0.0, 0.0, 0.0, 0.0, 0.0, 0.0, 0.0, 0.0, 0.0, 0.0, 0.0, 0.0, 0.0, 0.0, 0.0, 0.0, 0.0]] ("单体数据")) -> ()
                n244 = local write "预充继电器"(w1659) -> ()
                n245 = global write "单体信息全局.vi" "温度数据"(sgl[][] [[0.0, 0.0, 0.0, 0.0, 0.0, 0.0, 0.0, 0.0, 0.0, 0.0, 0.0], [0.0, 0.0, 0.0, 0.0, 0.0, 0.0, 0.0, 0.0, 0.0, 0.0, 0.0], [0.0, 0.0, 0.0, 0.0, 0.0, 0.0, 0.0, 0.0, 0.0, 0.0, 0.0], [0.0, 0.0, 0.0, 0.0, 0.0, 0.0, 0.0, 0.0, 0.0, 0.0, 0.0], [0.0, 0.0, 0.0, 0.0, 0.0, 0.0, 0.0, 0.0, 0.0, 0.0, 0.0], [0.0, 0.0, 0.0, 0.0, 0.0, 0.0, 0.0, 0.0, 0.0, 0.0, 0.0], [0.0, 0.0, 0.0, 0.0, 0.0, 0.0, 0.0, 0.0, 0.0, 0.0, 0.0], [0.0, 0.0, 0.0, 0.0, 0.0, 0.0, 0.0, 0.0, 0.0, 0.0, 0.0], [0.0, 0.0, 0.0, 0.0, 0.0, 0.0, 0.0, 0.0, 0.0, 0.0, 0.0], [0.0, 0.0, 0.0, 0.0, 0.0, 0.0, 0.0, 0.0, 0.0, 0.0, 0.0], [0.0, 0.0, 0.0, 0.0, 0.0, 0.0, 0.0, 0.0, 0.0, 0.0, 0.0], [0.0, 0.0, 0.0, 0.0, 0.0, 0.0, 0.0, 0.0, 0.0, 0.0, 0.0], [0.0, 0.0, 0.0, 0.0, 0.0, 0.0, 0.0, 0.0, 0.0, 0.0, 0.0], [0.0, 0.0, 0.0, 0.0, 0.0, 0.0, 0.0, 0.0, 0.0, 0.0, 0.0], [0.0, 0.0, 0.0, 0.0, 0.0, 0.0, 0.0, 0.0, 0.0, 0.0, 0.0], [0.0, 0.0, 0.0, 0.0, 0.0, 0.0, 0.0, 0.0, 0.0, 0.0, 0.0], [0.0, 0.0, 0.0, 0.0, 0.0, 0.0, 0.0, 0.0, 0.0, 0.0, 0.0], [0.0, 0.0, 0.0, 0.0, 0.0, 0.0, 0.0, 0.0, 0.0, 0.0, 0.0], [0.0, 0.0, 0.0, 0.0, 0.0, 0.0, 0.0, 0.0, 0.0, 0.0, 0.0], [0.0, 0.0, 0.0, 0.0, 0.0, 0.0, 0.0, 0.0, 0.0, 0.0, 0.0], [0.0, 0.0, 0.0, 0.0, 0.0, 0.0, 0.0, 0.0, 0.0, 0.0, 0.0], [0.0, 0.0, 0.0, 0.0, 0.0, 0.0, 0.0, 0.0, 0.0, 0.0, 0.0], [0.0, 0.0, 0.0, 0.0, 0.0, 0.0, 0.0, 0.0, 0.0, 0.0, 0.0], [0.0, 0.0, 0.0, 0.0, 0.0, 0.0, 0.0, 0.0, 0.0, 0.0, 0.0], [0.0, 0.0, 0.0, 0.0, 0.0, 0.0, 0.0, 0.0, 0.0, 0.0, 0.0], [0.0, 0.0, 0.0, 0.0, 0.0, 0.0, 0.0, 0.0, 0.0, 0.0, 0.0], [0.0, 0.0, 0.0, 0.0, 0.0, 0.0, 0.0, 0.0, 0.0, 0.0, 0.0], [0.0, 0.0, 0.0, 0.0, 0.0, 0.0, 0.0, 0.0, 0.0, 0.0, 0.0], [0.0, 0.0, 0.0, 0.0, 0.0, 0.0, 0.0, 0.0, 0.0, 0.0, 0.0], [0.0, 0.0, 0.0, 0.0, 0.0, 0.0, 0.0, 0.0, 0.0, 0.0, 0.0], [0.0, 0.0, 0.0, 0.0, 0.0, 0.0, 0.0, 0.0, 0.0, 0.0, 0.0]] ("温度数据")) -> ()
                n246 = local write "BMS时间"(w1658) -> ()
                n247 = local write "状态"(w1658) -> ()
                n248 = local write "系统运行模式"(w1658) -> ()
                n249 = local write "故障信息概况"(w1658) -> ()
                n250 = local write "LIFE"(w1658) -> ()
                n251 = local write "电池系统绝缘状态"(w1658) -> ()
                n252 = local write "次要参数"(T5 {"最高单体电压"=0.0, "最高电压位置"=0.0, "最低单体电压"=0.0, "最低电压位置"=0.0, "压差"=0.0, "最高单体温度"=0.0, "最高温度位置"=0.0, "最低单体温度"=0.0, "最低温度位置"=0.0, "温差"=0.0, "最高单体内阻"=0.0, "最高内阻位置"=0.0, "最低单体内阻"=0.0, "最低内阻位置"=0.0, "总内阻"=0.0, "协议是否公开"="", "协议版本号"="", "应用类型"="", "波特率"=""} ("次要参数")) -> ()
                n253 = local write "DI3"(w1654) -> ()
                n254 = local write "DI2"(w1654) -> ()
                n255 = local write "DI1"(w1654) -> ()
                n256 = local write "DI4"(w1654) -> ()
                n257 = local write "加热"(w1654) -> ()
                n258 = local write "DO2"(w1654) -> ()
                n259 = local write "风机"(w1654) -> ()
                n260 = local write "DO1"(w1654) -> ()
                n261 = local write "总电流进度"(w1656) -> ()
                n262 = invoke on="System XY Graph" class="XYGraph (严格)" method="Reinit To Default"() -> ()  [unwired: 3 in, 3 out]
                n263 = invoke on="System XY Graph 3" class="XYGraph (严格)" method="Reinit To Default"() -> ()  [unwired: 3 in, 3 out]
                n264 = local write "总电压进度"(w1656) -> ()
                n265 = local write "总电流(A)"(w1655) -> ()
                n266 = local write "平均电流"(w1655) -> ()
                n267 = local write "外总压"(w1655) -> ()
                n268 = local write "总电压(V)"(w1655) -> ()
                n269 = local write "CP"(w1653) -> ()
                n270 = local write "CC2"(w1653) -> ()
                n271 = local write "AI1"(w1653) -> ()
                n272 = local write "AI2"(w1653) -> ()
                n273 = local write "CC"(w1653) -> ()
              }
            }
          }
          event Timeout {
            n274 = event-data() -> ()  [unwired: 4 out]
            n275 = global read "功能码全局.vi" "14"() -> (w1665:bool[])
            n276 = local read "数值"() -> (w1663:i32)
            n277 = local read "中英文选择"() -> (w1668:enum32{"中文", "English"})
            n278 = Greater?(x=w1663, y=0) -> (0:w1667:bool)
            n279 = Index Array(array=w1665, index=6 ("索引")) -> (element=w1664:bool)
            n280 = And(x=w1664, y=w1667) -> ()  [unwired: 1 out]
            n281 = case shown="\"中文\", 默认" w1668 {
              tunnel: TRUE -> [w1675 w1676]
              frame "中文", Default {
                n282 = property on="单箱信息" class="Bool (严格)"("Visible"=w1675) -> ()  [unwired: 2 in, 2 out]
              }
              frame "English" {
                n283 = property on="单板信息 3" class="Bool (严格)"("Visible"=w1676) -> ()  [unwired: 2 in, 2 out]
              }
            }
            n284 = local read "状态"() -> (w1669:bool)
            n285 = global write "EV05全局变量1.vi" "数据接收"(w1669) -> ()
            n286 = global read "电池信息全局变量.vi" "允许保存数据"() -> (w1660:bool)
            n287 = case shown="假" w1660 {
              frame False {
                n288 = global read "电池信息全局变量.vi" "刷新计数"() -> (w1673:dbl)
                n289 = Increment(x=w1673) -> (x+1=w1672:dbl)
                n290 = Equal?(x=w1672, y=25.0) -> (x = y?=w1670:bool)
                n291 = case shown="真" w1670 {
                  frame False {
                  }
                  frame True {
                    n292 = global write "电池信息全局变量.vi" "允许保存数据"(TRUE ("允许保存数据")) -> ()
                  }
                }
                n293 = global write "电池信息全局变量.vi" "刷新计数"(w1672) -> ()
              }
              frame True {
              }
            }
          }
          event "故障信息概况": Mouse Up {
            n294 = event-data() -> ()  [unwired: 9 out]
            n295 = local read "CAN初始化成功"() -> (w1677:bool)
            n296 = case shown="真" w1677 {
              frame False {
              }
              frame True {
                n297 = stacked-sequence {
                  frame #0 {
                    w1678 = 2
                    n298 = property on="单箱信息" class="Bool (严格)"("Disabled"=w1678) -> ()  [unwired: 2 in, 2 out]
                    n299 = property on="诊断标定" class="Bool (严格)"("Disabled"=w1678) -> ()  [unwired: 2 in, 2 out]
                    n300 = property on="电压温度" class="Bool (严格)"("Disabled"=w1678) -> ()  [unwired: 2 in, 2 out]
                    n301 = property on="详细信息 3" class="Bool (严格)"("Disabled"=w1678) -> ()  [unwired: 2 in, 2 out]
                    n302 = property on="诊断标定 3" class="Bool (严格)"("Disabled"=w1678) -> ()  [unwired: 2 in, 2 out]
                    n303 = property on="单板信息 3" class="Bool (严格)"("Disabled"=w1678) -> ()  [unwired: 2 in, 2 out]
                  }
                  frame #1 {
                    n304 = local read "设备索引号"() -> (w1681:u16)
                    n305 = local read "CAN卡类型"() -> (w1682:u32)
                    n306 = local read "CAN端口"() -> (w1680:u16)
                    n307 = call-by-ref "?"("can卡类型"=w1682, "设备索引号"=w1681, "CAN端口"=w1680, "主界面选项 3"=enum32{"单选选项1", "单选选项2 2", "单选选项2 3", "单选选项2 4"}."单选选项2 4") -> ()  [unwired: 18 in, 2 out]
                  }
                  frame #2 {
                    w1683 = 0
                    n308 = property on="单箱信息" class="Bool (严格)"("Disabled"=w1683) -> ()  [unwired: 2 in, 2 out]
                    n309 = property on="诊断标定" class="Bool (严格)"("Disabled"=w1683) -> ()  [unwired: 2 in, 2 out]
                    n310 = property on="电压温度" class="Bool (严格)"("Disabled"=w1683) -> ()  [unwired: 2 in, 2 out]
                    n311 = property on="详细信息 3" class="Bool (严格)"("Disabled"=w1683) -> ()  [unwired: 2 in, 2 out]
                    n312 = property on="诊断标定 3" class="Bool (严格)"("Disabled"=w1683) -> ()  [unwired: 2 in, 2 out]
                    n313 = property on="单板信息 3" class="Bool (严格)"("Disabled"=w1683) -> ()  [unwired: 2 in, 2 out]
                  }
                }
              }
            }
          }
          event "故障信息": Mouse Up {
            n314 = event-data() -> ()  [unwired: 9 out]
            n315 = local read "CAN初始化成功"() -> (w1684:bool)
            n316 = case shown="真" w1684 {
              frame False {
              }
              frame True {
                n317 = stacked-sequence {
                  frame #0 {
                    n318 = disable-structure shown="禁用" {
                      frame Disabled {
                        w1685 = 2
                        n319 = property on="单箱信息" class="Bool (严格)"("Disabled"=w1685) -> ()  [unwired: 2 in, 2 out]
                        n320 = property on="诊断标定" class="Bool (严格)"("Disabled"=w1685) -> ()  [unwired: 2 in, 2 out]
                        n321 = property on="电压温度" class="Bool (严格)"("Disabled"=w1685) -> ()  [unwired: 2 in, 2 out]
                        n322 = property on="充电信息" class="Bool (严格)"("DisabledEnum"=w1685) -> ()  [unwired: 2 in, 2 out]
                        n323 = property on="系统信息" class="Bool (严格)"("DisabledEnum"=w1685) -> ()  [unwired: 2 in, 2 out]
                        n324 = property on="详细信息 3" class="Bool (严格)"("Disabled"=w1685) -> ()  [unwired: 2 in, 2 out]
                        n325 = property on="诊断标定 3" class="Bool (严格)"("Disabled"=w1685) -> ()  [unwired: 2 in, 2 out]
                        n326 = property on="单板信息 3" class="Bool (严格)"("Disabled"=w1685) -> ()  [unwired: 2 in, 2 out]
                      }
                      frame Enabled {
                      }
                    }
                  }
                  frame #1 {
                    n327 = local read "设备索引号"() -> (w1688:u16)
                    n328 = local read "CAN卡类型"() -> (w1689:u32)
                    n329 = local read "CAN端口"() -> (w1687:u16)
                    n330 = call-by-ref "?"("can卡类型"=w1689, "设备索引号"=w1688, "CAN端口"=w1687, "主界面选项 3"=enum32{"单选选项1", "单选选项2 2", "单选选项2 3", "单选选项2 4"}."单选选项2 4") -> ()  [unwired: 18 in, 2 out]
                  }
                  frame #2 {
                    n331 = disable-structure shown="禁用" {
                      frame Disabled {
                        w1690 = 0
                        n332 = property on="单箱信息" class="Bool (严格)"("Disabled"=w1690) -> ()  [unwired: 2 in, 2 out]
                        n333 = property on="诊断标定" class="Bool (严格)"("Disabled"=w1690) -> ()  [unwired: 2 in, 2 out]
                        n334 = property on="电压温度" class="Bool (严格)"("Disabled"=w1690) -> ()  [unwired: 2 in, 2 out]
                        n335 = property on="充电信息" class="Bool (严格)"("DisabledEnum"=w1690) -> ()  [unwired: 2 in, 2 out]
                        n336 = property on="系统信息" class="Bool (严格)"("DisabledEnum"=w1690) -> ()  [unwired: 2 in, 2 out]
                        n337 = property on="详细信息 3" class="Bool (严格)"("Disabled"=w1690) -> ()  [unwired: 2 in, 2 out]
                        n338 = property on="诊断标定 3" class="Bool (严格)"("Disabled"=w1690) -> ()  [unwired: 2 in, 2 out]
                        n339 = property on="单板信息 3" class="Bool (严格)"("Disabled"=w1690) -> ()  [unwired: 2 in, 2 out]
                      }
                      frame Enabled {
                      }
                    }
                  }
                }
              }
            }
          }
          event "充电信息": Mouse Up {
            n340 = event-data() -> ()  [unwired: 9 out]
            n341 = local read "CAN初始化成功"() -> (w1691:bool)
            n342 = case shown="真" w1691 {
              frame False {
              }
              frame True {
                n343 = stacked-sequence {
                  frame #0 {
                    n344 = disable-structure shown="禁用" {
                      frame Disabled {
                        w1692 = 2
                        n345 = property on="诊断标定" class="Bool (严格)"("Disabled"=w1692) -> ()  [unwired: 2 in, 2 out]
                        n346 = property on="单箱信息" class="Bool (严格)"("Disabled"=w1692) -> ()  [unwired: 2 in, 2 out]
                        n347 = property on="电压温度" class="Bool (严格)"("Disabled"=w1692) -> ()  [unwired: 2 in, 2 out]
                        n348 = property on="系统信息" class="Bool (严格)"("DisabledEnum"=w1692) -> ()  [unwired: 2 in, 2 out]
                        n349 = property on="详细信息 3" class="Bool (严格)"("Disabled"=w1692) -> ()  [unwired: 2 in, 2 out]
                        n350 = property on="诊断标定 3" class="Bool (严格)"("Disabled"=w1692) -> ()  [unwired: 2 in, 2 out]
                        n351 = property on="单板信息 3" class="Bool (严格)"("Disabled"=w1692) -> ()  [unwired: 2 in, 2 out]
                        n352 = property on="故障信息" class="Bool (严格)"("DisabledEnum"=w1692) -> ()  [unwired: 2 in, 2 out]
                      }
                      frame Enabled {
                      }
                    }
                  }
                  frame #1 {
                    n353 = local read "设备索引号"() -> (w1695:u16)
                    n354 = local read "CAN卡类型"() -> (w1696:u32)
                    n355 = local read "CAN端口"() -> (w1694:u16)
                    n356 = call-by-ref "?"("can卡类型"=w1696, "设备索引号"=w1695, "CAN端口"=w1694, "主界面选项 3"=enum32{"单选选项1", "单选选项2 2", "单选选项2 3", "单选选项2 4"}."单选选项2 3") -> ()  [unwired: 18 in, 2 out]
                  }
                  frame #2 {
                    n357 = disable-structure shown="禁用" {
                      frame Disabled {
                        w1697 = 0
                        n358 = property on="单箱信息" class="Bool (严格)"("Disabled"=w1697) -> ()  [unwired: 2 in, 2 out]
                        n359 = property on="诊断标定" class="Bool (严格)"("Disabled"=w1697) -> ()  [unwired: 2 in, 2 out]
                        n360 = property on="电压温度" class="Bool (严格)"("Disabled"=w1697) -> ()  [unwired: 2 in, 2 out]
                        n361 = property on="系统信息" class="Bool (严格)"("DisabledEnum"=w1697) -> ()  [unwired: 2 in, 2 out]
                        n362 = property on="故障信息" class="Bool (严格)"("DisabledEnum"=w1697) -> ()  [unwired: 2 in, 2 out]
                        n363 = property on="详细信息 3" class="Bool (严格)"("Disabled"=w1697) -> ()  [unwired: 2 in, 2 out]
                        n364 = property on="诊断标定 3" class="Bool (严格)"("Disabled"=w1697) -> ()  [unwired: 2 in, 2 out]
                        n365 = property on="单板信息 3" class="Bool (严格)"("Disabled"=w1697) -> ()  [unwired: 2 in, 2 out]
                      }
                      frame Enabled {
                      }
                    }
                  }
                }
              }
            }
          }
          event "主界面选项": Value Change {
            n366 = event-data() -> ("NewVal"=w1702:T7)  [unwired: 6 out]
            n367 = case shown="\"总信息卡\", 默认" w1702 {
              tunnel: [T13."次要参数" ("图表选项卡") T13."单体电压" ("图表选项卡") T13."单体温度" ("图表选项卡")] -> w1703
              tunnel: [w1707 w1711 w1716] -> w1699
              tunnel: [w1706 w1714 w1718] -> w1698
              frame "总信息卡", Default {
                n368 = control-ref of="单体电压卡"() -> (w1709:refnum<vi>)
                n369 = control-ref of="单体温度卡"() -> (w1708:refnum<vi>)
                n370 = control-ref of="总信息卡"() -> (w1706:refnum<vi>)
                n371 = Build Array(w1708, w1709) -> (w1707:refnum<vi>[])
              }
              frame "单体电压卡" {
                n372 = control-ref of="单体电压卡"() -> (w1714:refnum<vi>)
                n373 = control-ref of="单体温度卡"() -> (w1712:refnum<vi>)
                n374 = control-ref of="总信息卡"() -> (w1713:refnum<vi>)
                n375 = Build Array(w1713, w1712) -> (w1711:refnum<vi>[])
              }
              frame "单体温度卡" {
                n376 = control-ref of="单体电压卡"() -> (w1717:refnum<vi>)
                n377 = control-ref of="总信息卡"() -> (w1719:refnum<vi>)
                n378 = control-ref of="单体温度卡"() -> (w1718:refnum<vi>)
                n379 = Build Array(w1719, w1717) -> (w1716:refnum<vi>[])
              }
            }
            n380 = local write "图表选项卡"(w1703) -> ()
            n381 = for {
              tunnel: u32 16448250 -> [w1705]
              tunnel: w1699 -> [w1704] mode=indexing
              n382 = property class="Bool (严格)"(reference=w1704, "BoolText.TextColor"=w1705) -> ()  [unwired: 1 in, 2 out]
            }
            n383 = property class="Bool (严格)"(reference=w1698, "BoolText.TextColor"=u32 87470) -> ()  [unwired: 1 in, 2 out]
          }
          event "启动CAN 2", "CAN连接": Value Change {
            n384 = event-data() -> ("NewVal"=w1721:bool)  [unwired: 6 out]
            n385 = case shown="真" w1721 {
              frame True {
                n386 = local read "设备索引号"() -> (w1731:u16)
                n387 = local read "CAN卡类型"() -> (w1732:u32)
                n388 = local read "工作方式"() -> (w1726:u8)
                n389 = local read "滤波方式"() -> (w1727:u8)
                n390 = local read "CAN端口"() -> (w1729:u16)
                n391 = local read "波特率"() -> (w1730:u16)
                n392 = call-by-ref "?"("设备类型"=w1732, "设备索引"=w1731, "波特率"=w1730, "CAN路数"=w1729, "操作类型"=enum16{"初始化CAN", "关闭CAN"}."初始化CAN", "滤波方式"=w1727, "工作方式"=w1726) -> ("CAN 操作结果"=w1723:bool, "error out"=w1725:errorcluster)  [unwired: 13 in, 2 out]
                n393 = call <vilib>:"Clear Errors.vi"("error in (no error)"=w1725) -> ()  [unwired: 7 out]
                n394 = Not(x=w1723) -> (.not. x?=w1724:bool)
                n395 = local write "CAN初始化成功"(w1723) -> ()
                n396 = property on="字符串" class="Str"("Visible"=w1724) -> ()  [unwired: 2 in, 2 out]
                n397 = property on="CAN连接" class="Bool (严格)"("BoolText.TextColor"=u32 65511) -> ()  [unwired: 2 in, 2 out]
              }
              frame False {
                w1746 = FALSE
                n398 = local read "工作方式"() -> (w1737:u8)
                n399 = local read "滤波方式"() -> (w1738:u8)
                n400 = local read "CAN卡类型"() -> (w1739:u32)
                n401 = local read "设备索引号"() -> (w1740:u16)
                n402 = local read "CAN端口"() -> (w1742:u16)
                n403 = local read "波特率"() -> (w1741:u16)
                n404 = local write "开始保存"(FALSE ("开始保存")) -> ()
                n405 = disable-structure shown="启用" {
                  frame Enabled {
                    n406 = Request Deallocation(TRUE ("标志")) -> ()
                  }
                  frame Disabled {
                  }
                }
                n407 = call "CAN_Init - 2013.vi"("设备类型"=w1739, "设备索引"=w1740, "波特率"=w1741, "CAN路数"=w1742, "操作类型"=enum16{"初始化CAN", "关闭CAN"}."关闭CAN", "滤波方式"=w1738, "工作方式"=w1737) -> ("CAN 操作结果"=→"CAN 操作结果":bool, "error out"=w1744:errorcluster)  [unwired: 11 in]
                n408 = call <vilib>:"Clear Errors.vi"("error in (no error)"=w1744) -> ()  [unwired: 7 out]
                n409 = local write "CAN初始化成功"(w1746) -> ()
                n410 = property on="CAN连接" class="Bool (严格)"("BoolText.TextColor"=u32 16448250) -> ()  [unwired: 2 in, 2 out]
                n411 = local write "状态"(w1746) -> ()
                n412 = local write "dup path"(path "" ("dup path")) -> ()
                n413 = property on="字符串" class="Str"("Visible"=TRUE ("可见")) -> ()  [unwired: 2 in, 2 out]
              }
            }
          }
          event "总正": Shortcut Menu Selection (User) {
            n414 = event-data() -> ("ItemTag"=w1749:string)  [unwired: 8 out]
            n415 = local read "强制操作"() -> (w1748:bool)
            n416 = case shown="真" w1748 {
              tunnel: w1749 -> [_ w1750]
              frame False {
              }
              frame True {
                n417 = case shown="\"强制闭合\"" w1750 {
                  frame "假", Default {
                  }
                  frame "强制闭合" {
                    n418 = local read "CAN卡类型"() -> (w1753:u32)
                    n419 = local read "设备索引号"() -> (w1752:u16)
                    n420 = local read "CAN端口"() -> (w1751:u16)
                    n421 = case shown="假" TRUE {
                      selector: TRUE -> [w1772 w1792]
                      tunnel: [w1771 w1791] -> _
                      tunnel: [w1759 w1779] -> _
                      tunnel: w1753 -> [w1757 w1777]
                      tunnel: w1752 -> [w1756 w1776]
                      tunnel: w1751 -> [w1755 w1775]
                      frame False {
                        w1767 = 256.0 ("y")
                        w1759 = u32 1 ("命令序号")
                        w1771 = u8 192 ("命令")
                        n422 = local read "动作保持时间"() -> (w1768:dbl)
                        n423 = Quotient & Remainder(x=w1768, y=w1767) -> (x-y*floor(x/y)=w1760:dbl, floor(x/y)=w1764:dbl)
                        n424 = Quotient & Remainder(x=w1764, y=w1767) -> (x-y*floor(x/y)=w1761:dbl, floor(x/y)=w1765:dbl)
                        n425 = Quotient & Remainder(x=w1765, y=w1767) -> (x-y*floor(x/y)=w1762:dbl, floor(x/y)=w1766:dbl)
                        n426 = Boolean To (0,1)(Boolean=w1772) -> (0, 1=w1769:i16)
                        n427 = Quotient & Remainder(x=w1766, y=w1767) -> (x-y*floor(x/y)=w1763:dbl)  [unwired: 1 out]
                        n428 = Build Array(i16 1 ("元素"), w1769, w1763, w1762, w1761, w1760, 0.0 ("元素")) -> (w1773:dbl[])
                        n429 = call "多帧发送机制(EV05).vi"("can卡类型"=w1757, "设备索引号"=w1756, "CAN端口"=w1755, "命令"=w1771, "板号"=u8 0, "命令序号"=w1759, "输入数据"=w1773) -> ()  [unwired: 1 in, 12 out]
                      }
                      frame True {
                        w1787 = 256.0 ("y")
                        w1779 = u32 1 ("命令序号")
                        w1791 = u8 192 ("命令")
                        n430 = local read "动作保持时间"() -> (w1788:dbl)
                        n431 = Quotient & Remainder(x=w1788, y=w1787) -> (x-y*floor(x/y)=w1780:dbl, floor(x/y)=w1784:dbl)
                        n432 = Quotient & Remainder(x=w1784, y=w1787) -> (x-y*floor(x/y)=w1781:dbl, floor(x/y)=w1785:dbl)
                        n433 = Quotient & Remainder(x=w1785, y=w1787) -> (x-y*floor(x/y)=w1782:dbl, floor(x/y)=w1786:dbl)
                        n434 = Boolean To (0,1)(Boolean=w1792) -> (0, 1=w1789:i16)
                        n435 = Quotient & Remainder(x=w1786, y=w1787) -> (x-y*floor(x/y)=w1783:dbl)  [unwired: 1 out]
                        n436 = Build Array(i16 1 ("元素"), w1789, w1783, w1782, w1781, w1780, 0.0 ("元素")) -> (w1793:dbl[])
                        n437 = call "多帧发送机制(EV05).vi"("can卡类型"=w1777, "设备索引号"=w1776, "CAN端口"=w1775, "命令"=w1791, "板号"=u8 0, "命令序号"=w1779, "输入数据"=w1793) -> ()  [unwired: 1 in, 12 out]
                      }
                    }
                  }
                  frame "强制断开" {
                    n438 = local read "CAN卡类型"() -> (w1797:u32)
                    n439 = local read "设备索引号"() -> (w1796:u16)
                    n440 = local read "CAN端口"() -> (w1795:u16)
                    n441 = case shown="假" FALSE {
                      selector: FALSE -> [w1816 w1836]
                      tunnel: [w1815 w1835] -> _
                      tunnel: [w1803 w1823] -> _
                      tunnel: w1797 -> [w1801 w1821]
                      tunnel: w1796 -> [w1800 w1820]
                      tunnel: w1795 -> [w1799 w1819]
                      frame False {
                        w1811 = 256.0 ("y")
                        w1803 = u32 1 ("命令序号")
                        w1815 = u8 192 ("命令")
                        n442 = local read "动作保持时间"() -> (w1812:dbl)
                        n443 = Quotient & Remainder(x=w1812, y=w1811) -> (x-y*floor(x/y)=w1804:dbl, floor(x/y)=w1808:dbl)
                        n444 = Quotient & Remainder(x=w1808, y=w1811) -> (x-y*floor(x/y)=w1805:dbl, floor(x/y)=w1809:dbl)
                        n445 = Quotient & Remainder(x=w1809, y=w1811) -> (x-y*floor(x/y)=w1806:dbl, floor(x/y)=w1810:dbl)
                        n446 = Boolean To (0,1)(Boolean=w1816) -> (0, 1=w1813:i16)
                        n447 = Quotient & Remainder(x=w1810, y=w1811) -> (x-y*floor(x/y)=w1807:dbl)  [unwired: 1 out]
                        n448 = Build Array(i16 1 ("元素"), w1813, w1807, w1806, w1805, w1804, 0.0 ("元素")) -> (w1817:dbl[])
                        n449 = call "多帧发送机制(EV05).vi"("can卡类型"=w1801, "设备索引号"=w1800, "CAN端口"=w1799, "命令"=w1815, "板号"=u8 0, "命令序号"=w1803, "输入数据"=w1817) -> ()  [unwired: 1 in, 12 out]
                      }
                      frame True {
                        w1831 = 256.0 ("y")
                        w1823 = u32 1 ("命令序号")
                        w1835 = u8 192 ("命令")
                        n450 = local read "动作保持时间"() -> (w1832:dbl)
                        n451 = Quotient & Remainder(x=w1832, y=w1831) -> (x-y*floor(x/y)=w1824:dbl, floor(x/y)=w1828:dbl)
                        n452 = Quotient & Remainder(x=w1828, y=w1831) -> (x-y*floor(x/y)=w1825:dbl, floor(x/y)=w1829:dbl)
                        n453 = Quotient & Remainder(x=w1829, y=w1831) -> (x-y*floor(x/y)=w1826:dbl, floor(x/y)=w1830:dbl)
                        n454 = Boolean To (0,1)(Boolean=w1836) -> (0, 1=w1833:i16)
                        n455 = Quotient & Remainder(x=w1830, y=w1831) -> (x-y*floor(x/y)=w1827:dbl)  [unwired: 1 out]
                        n456 = Build Array(i16 1 ("元素"), w1833, w1827, w1826, w1825, w1824, 0.0 ("元素")) -> (w1837:dbl[])
                        n457 = call "多帧发送机制(EV05).vi"("can卡类型"=w1821, "设备索引号"=w1820, "CAN端口"=w1819, "命令"=w1835, "板号"=u8 0, "命令序号"=w1823, "输入数据"=w1837) -> ()  [unwired: 1 in, 12 out]
                      }
                    }
                  }
                }
              }
            }
          }
          event "总负": Shortcut Menu Selection (User) {
            n458 = event-data() -> ("ItemTag"=w1840:string)  [unwired: 8 out]
            n459 = local read "强制操作"() -> (w1839:bool)
            n460 = case shown="真" w1839 {
              tunnel: w1840 -> [_ w1841]
              frame False {
              }
              frame True {
                n461 = case shown="\"强制断开\"" w1841 {
                  frame "假", Default {
                  }
                  frame "强制闭合" {
                    n462 = local read "CAN卡类型"() -> (w1844:u32)
                    n463 = local read "设备索引号"() -> (w1843:u16)
                    n464 = local read "CAN端口"() -> (w1842:u16)
                    n465 = case shown="真" TRUE {
                      selector: TRUE -> [w1863 w1883]
                      tunnel: [w1862 w1882] -> _
                      tunnel: [w1850 w1870] -> _
                      tunnel: w1844 -> [w1848 w1868]
                      tunnel: w1843 -> [w1847 w1867]
                      tunnel: w1842 -> [w1846 w1866]
                      frame False {
                        w1858 = 256.0 ("y")
                        w1850 = u32 1 ("命令序号")
                        w1862 = u8 192 ("命令")
                        n466 = local read "动作保持时间"() -> (w1859:dbl)
                        n467 = Quotient & Remainder(x=w1859, y=w1858) -> (x-y*floor(x/y)=w1851:dbl, floor(x/y)=w1855:dbl)
                        n468 = Quotient & Remainder(x=w1855, y=w1858) -> (x-y*floor(x/y)=w1852:dbl, floor(x/y)=w1856:dbl)
                        n469 = Quotient & Remainder(x=w1856, y=w1858) -> (x-y*floor(x/y)=w1853:dbl, floor(x/y)=w1857:dbl)
                        n470 = Boolean To (0,1)(Boolean=w1863) -> (0, 1=w1860:i16)
                        n471 = Quotient & Remainder(x=w1857, y=w1858) -> (x-y*floor(x/y)=w1854:dbl)  [unwired: 1 out]
                        n472 = Build Array(i16 2 ("元素"), w1860, w1854, w1853, w1852, w1851, 0.0 ("元素")) -> (w1864:dbl[])
                        n473 = call "多帧发送机制(EV05).vi"("can卡类型"=w1848, "设备索引号"=w1847, "CAN端口"=w1846, "命令"=w1862, "板号"=u8 0, "命令序号"=w1850, "输入数据"=w1864) -> ()  [unwired: 1 in, 12 out]
                      }
                      frame True {
                        w1878 = 256.0 ("y")
                        w1870 = u32 1 ("命令序号")
                        w1882 = u8 192 ("命令")
                        n474 = local read "动作保持时间"() -> (w1879:dbl)
                        n475 = Quotient & Remainder(x=w1879, y=w1878) -> (x-y*floor(x/y)=w1871:dbl, floor(x/y)=w1875:dbl)
                        n476 = Quotient & Remainder(x=w1875, y=w1878) -> (x-y*floor(x/y)=w1872:dbl, floor(x/y)=w1876:dbl)
                        n477 = Quotient & Remainder(x=w1876, y=w1878) -> (x-y*floor(x/y)=w1873:dbl, floor(x/y)=w1877:dbl)
                        n478 = Boolean To (0,1)(Boolean=w1883) -> (0, 1=w1880:i16)
                        n479 = Quotient & Remainder(x=w1877, y=w1878) -> (x-y*floor(x/y)=w1874:dbl)  [unwired: 1 out]
                        n480 = Build Array(i16 2 ("元素"), w1880, w1874, w1873, w1872, w1871, 0.0 ("元素")) -> (w1884:dbl[])
                        n481 = call "多帧发送机制(EV05).vi"("can卡类型"=w1868, "设备索引号"=w1867, "CAN端口"=w1866, "命令"=w1882, "板号"=u8 0, "命令序号"=w1870, "输入数据"=w1884) -> ()  [unwired: 1 in, 12 out]
                      }
                    }
                  }
                  frame "强制断开" {
                    n482 = local read "CAN卡类型"() -> (w1888:u32)
                    n483 = local read "设备索引号"() -> (w1887:u16)
                    n484 = local read "CAN端口"() -> (w1886:u16)
                    n485 = case shown="真" FALSE {
                      selector: FALSE -> [w1907 w1927]
                      tunnel: [w1906 w1926] -> _
                      tunnel: [w1894 w1914] -> _
                      tunnel: w1888 -> [w1892 w1912]
                      tunnel: w1887 -> [w1891 w1911]
                      tunnel: w1886 -> [w1890 w1910]
                      frame False {
                        w1902 = 256.0 ("y")
                        w1894 = u32 1 ("命令序号")
                        w1906 = u8 192 ("命令")
                        n486 = local read "动作保持时间"() -> (w1903:dbl)
                        n487 = Quotient & Remainder(x=w1903, y=w1902) -> (x-y*floor(x/y)=w1895:dbl, floor(x/y)=w1899:dbl)
                        n488 = Quotient & Remainder(x=w1899, y=w1902) -> (x-y*floor(x/y)=w1896:dbl, floor(x/y)=w1900:dbl)
                        n489 = Quotient & Remainder(x=w1900, y=w1902) -> (x-y*floor(x/y)=w1897:dbl, floor(x/y)=w1901:dbl)
                        n490 = Boolean To (0,1)(Boolean=w1907) -> (0, 1=w1904:i16)
                        n491 = Quotient & Remainder(x=w1901, y=w1902) -> (x-y*floor(x/y)=w1898:dbl)  [unwired: 1 out]
                        n492 = Build Array(i16 2 ("元素"), w1904, w1898, w1897, w1896, w1895, 0.0 ("元素")) -> (w1908:dbl[])
                        n493 = call "多帧发送机制(EV05).vi"("can卡类型"=w1892, "设备索引号"=w1891, "CAN端口"=w1890, "命令"=w1906, "板号"=u8 0, "命令序号"=w1894, "输入数据"=w1908) -> ()  [unwired: 1 in, 12 out]
                      }
                      frame True {
                        w1922 = 256.0 ("y")
                        w1914 = u32 1 ("命令序号")
                        w1926 = u8 192 ("命令")
                        n494 = local read "动作保持时间"() -> (w1923:dbl)
                        n495 = Quotient & Remainder(x=w1923, y=w1922) -> (x-y*floor(x/y)=w1915:dbl, floor(x/y)=w1919:dbl)
                        n496 = Quotient & Remainder(x=w1919, y=w1922) -> (x-y*floor(x/y)=w1916:dbl, floor(x/y)=w1920:dbl)
                        n497 = Quotient & Remainder(x=w1920, y=w1922) -> (x-y*floor(x/y)=w1917:dbl, floor(x/y)=w1921:dbl)
                        n498 = Boolean To (0,1)(Boolean=w1927) -> (0, 1=w1924:i16)
                        n499 = Quotient & Remainder(x=w1921, y=w1922) -> (x-y*floor(x/y)=w1918:dbl)  [unwired: 1 out]
                        n500 = Build Array(i16 2 ("元素"), w1924, w1918, w1917, w1916, w1915, 0.0 ("元素")) -> (w1928:dbl[])
                        n501 = call "多帧发送机制(EV05).vi"("can卡类型"=w1912, "设备索引号"=w1911, "CAN端口"=w1910, "命令"=w1926, "板号"=u8 0, "命令序号"=w1914, "输入数据"=w1928) -> ()  [unwired: 1 in, 12 out]
                      }
                    }
                  }
                }
              }
            }
          }
          event "预充": Shortcut Menu Selection (User) {
            n502 = event-data() -> ("ItemTag"=w1931:string)  [unwired: 8 out]
            n503 = local read "强制操作"() -> (w1930:bool)
            n504 = case shown="真" w1930 {
              tunnel: w1931 -> [_ w1932]
              frame False {
              }
              frame True {
                n505 = case shown="\"强制闭合\"" w1932 {
                  frame "假", Default {
                  }
                  frame "强制闭合" {
                    n506 = local read "CAN卡类型"() -> (w1935:u32)
                    n507 = local read "设备索引号"() -> (w1934:u16)
                    n508 = local read "CAN端口"() -> (w1933:u16)
                    n509 = case shown="假" TRUE {
                      selector: TRUE -> [w1954 w1974]
                      tunnel: [w1953 w1973] -> _
                      tunnel: [w1941 w1961] -> _
                      tunnel: w1935 -> [w1939 w1959]
                      tunnel: w1934 -> [w1938 w1958]
                      tunnel: w1933 -> [w1937 w1957]
                      frame False {
                        w1949 = 256.0 ("y")
                        w1941 = u32 1 ("命令序号")
                        w1953 = u8 192 ("命令")
                        n510 = local read "动作保持时间"() -> (w1950:dbl)
                        n511 = Quotient & Remainder(x=w1950, y=w1949) -> (x-y*floor(x/y)=w1942:dbl, floor(x/y)=w1946:dbl)
                        n512 = Quotient & Remainder(x=w1946, y=w1949) -> (x-y*floor(x/y)=w1943:dbl, floor(x/y)=w1947:dbl)
                        n513 = Quotient & Remainder(x=w1947, y=w1949) -> (x-y*floor(x/y)=w1944:dbl, floor(x/y)=w1948:dbl)
                        n514 = Boolean To (0,1)(Boolean=w1954) -> (0, 1=w1951:i16)
                        n515 = Quotient & Remainder(x=w1948, y=w1949) -> (x-y*floor(x/y)=w1945:dbl)  [unwired: 1 out]
                        n516 = Build Array(i16 3 ("元素"), w1951, w1945, w1944, w1943, w1942, 0.0 ("元素")) -> (w1955:dbl[])
                        n517 = call "多帧发送机制(EV05).vi"("can卡类型"=w1939, "设备索引号"=w1938, "CAN端口"=w1937, "命令"=w1953, "板号"=u8 0, "命令序号"=w1941, "输入数据"=w1955) -> ()  [unwired: 1 in, 12 out]
                      }
                      frame True {
                        w1969 = 256.0 ("y")
                        w1961 = u32 1 ("命令序号")
                        w1973 = u8 192 ("命令")
                        n518 = local read "动作保持时间"() -> (w1970:dbl)
                        n519 = Quotient & Remainder(x=w1970, y=w1969) -> (x-y*floor(x/y)=w1962:dbl, floor(x/y)=w1966:dbl)
                        n520 = Quotient & Remainder(x=w1966, y=w1969) -> (x-y*floor(x/y)=w1963:dbl, floor(x/y)=w1967:dbl)
                        n521 = Quotient & Remainder(x=w1967, y=w1969) -> (x-y*floor(x/y)=w1964:dbl, floor(x/y)=w1968:dbl)
                        n522 = Boolean To (0,1)(Boolean=w1974) -> (0, 1=w1971:i16)
                        n523 = Quotient & Remainder(x=w1968, y=w1969) -> (x-y*floor(x/y)=w1965:dbl)  [unwired: 1 out]
                        n524 = Build Array(i16 3 ("元素"), w1971, w1965, w1964, w1963, w1962, 0.0 ("元素")) -> (w1975:dbl[])
                        n525 = call "多帧发送机制(EV05).vi"("can卡类型"=w1959, "设备索引号"=w1958, "CAN端口"=w1957, "命令"=w1973, "板号"=u8 0, "命令序号"=w1961, "输入数据"=w1975) -> ()  [unwired: 1 in, 12 out]
                      }
                    }
                  }
                  frame "强制断开" {
                    n526 = local read "CAN卡类型"() -> (w1979:u32)
                    n527 = local read "设备索引号"() -> (w1978:u16)
                    n528 = local read "CAN端口"() -> (w1977:u16)
                    n529 = case shown="假" FALSE {
                      selector: FALSE -> [w1998 w2018]
                      tunnel: [w1997 w2017] -> _
                      tunnel: [w1985 w2005] -> _
                      tunnel: w1979 -> [w1983 w2003]
                      tunnel: w1978 -> [w1982 w2002]
                      tunnel: w1977 -> [w1981 w2001]
                      frame False {
                        w1993 = 256.0 ("y")
                        w1985 = u32 1 ("命令序号")
                        w1997 = u8 192 ("命令")
                        n530 = local read "动作保持时间"() -> (w1994:dbl)
                        n531 = Quotient & Remainder(x=w1994, y=w1993) -> (x-y*floor(x/y)=w1986:dbl, floor(x/y)=w1990:dbl)
                        n532 = Quotient & Remainder(x=w1990, y=w1993) -> (x-y*floor(x/y)=w1987:dbl, floor(x/y)=w1991:dbl)
                        n533 = Quotient & Remainder(x=w1991, y=w1993) -> (x-y*floor(x/y)=w1988:dbl, floor(x/y)=w1992:dbl)
                        n534 = Boolean To (0,1)(Boolean=w1998) -> (0, 1=w1995:i16)
                        n535 = Quotient & Remainder(x=w1992, y=w1993) -> (x-y*floor(x/y)=w1989:dbl)  [unwired: 1 out]
                        n536 = Build Array(i16 3 ("元素"), w1995, w1989, w1988, w1987, w1986, 0.0 ("元素")) -> (w1999:dbl[])
                        n537 = call "多帧发送机制(EV05).vi"("can卡类型"=w1983, "设备索引号"=w1982, "CAN端口"=w1981, "命令"=w1997, "板号"=u8 0, "命令序号"=w1985, "输入数据"=w1999) -> ()  [unwired: 1 in, 12 out]
                      }
                      frame True {
                        w2013 = 256.0 ("y")
                        w2005 = u32 1 ("命令序号")
                        w2017 = u8 192 ("命令")
                        n538 = local read "动作保持时间"() -> (w2014:dbl)
                        n539 = Quotient & Remainder(x=w2014, y=w2013) -> (x-y*floor(x/y)=w2006:dbl, floor(x/y)=w2010:dbl)
                        n540 = Quotient & Remainder(x=w2010, y=w2013) -> (x-y*floor(x/y)=w2007:dbl, floor(x/y)=w2011:dbl)
                        n541 = Quotient & Remainder(x=w2011, y=w2013) -> (x-y*floor(x/y)=w2008:dbl, floor(x/y)=w2012:dbl)
                        n542 = Boolean To (0,1)(Boolean=w2018) -> (0, 1=w2015:i16)
                        n543 = Quotient & Remainder(x=w2012, y=w2013) -> (x-y*floor(x/y)=w2009:dbl)  [unwired: 1 out]
                        n544 = Build Array(i16 3 ("元素"), w2015, w2009, w2008, w2007, w2006, 0.0 ("元素")) -> (w2019:dbl[])
                        n545 = call "多帧发送机制(EV05).vi"("can卡类型"=w2003, "设备索引号"=w2002, "CAN端口"=w2001, "命令"=w2017, "板号"=u8 0, "命令序号"=w2005, "输入数据"=w2019) -> ()  [unwired: 1 in, 12 out]
                      }
                    }
                  }
                }
              }
            }
          }
          event "加热": Shortcut Menu Selection (User) {
            n546 = event-data() -> ("ItemTag"=w2022:string)  [unwired: 8 out]
            n547 = local read "强制操作"() -> (w2021:bool)
            n548 = case shown="真" w2021 {
              tunnel: w2022 -> [_ w2023]
              frame False {
              }
              frame True {
                n549 = case shown="\"强制断开\"" w2023 {
                  frame "假", Default {
                  }
                  frame "强制闭合" {
                    n550 = local read "CAN卡类型"() -> (w2026:u32)
                    n551 = local read "设备索引号"() -> (w2025:u16)
                    n552 = local read "CAN端口"() -> (w2024:u16)
                    n553 = case shown="真" TRUE {
                      selector: TRUE -> [w2045 w2065]
                      tunnel: [w2044 w2064] -> _
                      tunnel: [w2032 w2052] -> _
                      tunnel: w2026 -> [w2030 w2050]
                      tunnel: w2025 -> [w2029 w2049]
                      tunnel: w2024 -> [w2028 w2048]
                      frame False {
                        w2040 = 256.0 ("y")
                        w2032 = u32 1 ("命令序号")
                        w2044 = u8 192 ("命令")
                        n554 = local read "动作保持时间"() -> (w2041:dbl)
                        n555 = Quotient & Remainder(x=w2041, y=w2040) -> (x-y*floor(x/y)=w2033:dbl, floor(x/y)=w2037:dbl)
                        n556 = Quotient & Remainder(x=w2037, y=w2040) -> (x-y*floor(x/y)=w2034:dbl, floor(x/y)=w2038:dbl)
                        n557 = Quotient & Remainder(x=w2038, y=w2040) -> (x-y*floor(x/y)=w2035:dbl, floor(x/y)=w2039:dbl)
                        n558 = Boolean To (0,1)(Boolean=w2045) -> (0, 1=w2042:i16)
                        n559 = Quotient & Remainder(x=w2039, y=w2040) -> (x-y*floor(x/y)=w2036:dbl)  [unwired: 1 out]
                        n560 = Build Array(i16 4 ("元素"), w2042, w2036, w2035, w2034, w2033, 0.0 ("元素")) -> (w2046:dbl[])
                        n561 = call "多帧发送机制(EV05).vi"("can卡类型"=w2030, "设备索引号"=w2029, "CAN端口"=w2028, "命令"=w2044, "板号"=u8 0, "命令序号"=w2032, "输入数据"=w2046) -> ()  [unwired: 1 in, 12 out]
                      }
                      frame True {
                        w2060 = 256.0 ("y")
                        w2052 = u32 1 ("命令序号")
                        w2064 = u8 192 ("命令")
                        n562 = local read "动作保持时间"() -> (w2061:dbl)
                        n563 = Quotient & Remainder(x=w2061, y=w2060) -> (x-y*floor(x/y)=w2053:dbl, floor(x/y)=w2057:dbl)
                        n564 = Quotient & Remainder(x=w2057, y=w2060) -> (x-y*floor(x/y)=w2054:dbl, floor(x/y)=w2058:dbl)
                        n565 = Quotient & Remainder(x=w2058, y=w2060) -> (x-y*floor(x/y)=w2055:dbl, floor(x/y)=w2059:dbl)
                        n566 = Boolean To (0,1)(Boolean=w2065) -> (0, 1=w2062:i16)
                        n567 = Quotient & Remainder(x=w2059, y=w2060) -> (x-y*floor(x/y)=w2056:dbl)  [unwired: 1 out]
                        n568 = Build Array(i16 4 ("元素"), w2062, w2056, w2055, w2054, w2053, 0.0 ("元素")) -> (w2066:dbl[])
                        n569 = call "多帧发送机制(EV05).vi"("can卡类型"=w2050, "设备索引号"=w2049, "CAN端口"=w2048, "命令"=w2064, "板号"=u8 0, "命令序号"=w2052, "输入数据"=w2066) -> ()  [unwired: 1 in, 12 out]
                      }
                    }
                  }
                  frame "强制断开" {
                    n570 = local read "CAN卡类型"() -> (w2070:u32)
                    n571 = local read "设备索引号"() -> (w2069:u16)
                    n572 = local read "CAN端口"() -> (w2068:u16)
                    n573 = case shown="真" FALSE {
                      selector: FALSE -> [w2089 w2109]
                      tunnel: [w2088 w2108] -> _
                      tunnel: [w2076 w2096] -> _
                      tunnel: w2070 -> [w2074 w2094]
                      tunnel: w2069 -> [w2073 w2093]
                      tunnel: w2068 -> [w2072 w2092]
                      frame False {
                        w2084 = 256.0 ("y")
                        w2076 = u32 1 ("命令序号")
                        w2088 = u8 192 ("命令")
                        n574 = local read "动作保持时间"() -> (w2085:dbl)
                        n575 = Quotient & Remainder(x=w2085, y=w2084) -> (x-y*floor(x/y)=w2077:dbl, floor(x/y)=w2081:dbl)
                        n576 = Quotient & Remainder(x=w2081, y=w2084) -> (x-y*floor(x/y)=w2078:dbl, floor(x/y)=w2082:dbl)
                        n577 = Quotient & Remainder(x=w2082, y=w2084) -> (x-y*floor(x/y)=w2079:dbl, floor(x/y)=w2083:dbl)
                        n578 = Boolean To (0,1)(Boolean=w2089) -> (0, 1=w2086:i16)
                        n579 = Quotient & Remainder(x=w2083, y=w2084) -> (x-y*floor(x/y)=w2080:dbl)  [unwired: 1 out]
                        n580 = Build Array(i16 4 ("元素"), w2086, w2080, w2079, w2078, w2077, 0.0 ("元素")) -> (w2090:dbl[])
                        n581 = call "多帧发送机制(EV05).vi"("can卡类型"=w2074, "设备索引号"=w2073, "CAN端口"=w2072, "命令"=w2088, "板号"=u8 0, "命令序号"=w2076, "输入数据"=w2090) -> ()  [unwired: 1 in, 12 out]
                      }
                      frame True {
                        w2104 = 256.0 ("y")
                        w2096 = u32 1 ("命令序号")
                        w2108 = u8 192 ("命令")
                        n582 = local read "动作保持时间"() -> (w2105:dbl)
                        n583 = Quotient & Remainder(x=w2105, y=w2104) -> (x-y*floor(x/y)=w2097:dbl, floor(x/y)=w2101:dbl)
                        n584 = Quotient & Remainder(x=w2101, y=w2104) -> (x-y*floor(x/y)=w2098:dbl, floor(x/y)=w2102:dbl)
                        n585 = Quotient & Remainder(x=w2102, y=w2104) -> (x-y*floor(x/y)=w2099:dbl, floor(x/y)=w2103:dbl)
                        n586 = Boolean To (0,1)(Boolean=w2109) -> (0, 1=w2106:i16)
                        n587 = Quotient & Remainder(x=w2103, y=w2104) -> (x-y*floor(x/y)=w2100:dbl)  [unwired: 1 out]
                        n588 = Build Array(i16 4 ("元素"), w2106, w2100, w2099, w2098, w2097, 0.0 ("元素")) -> (w2110:dbl[])
                        n589 = call "多帧发送机制(EV05).vi"("can卡类型"=w2094, "设备索引号"=w2093, "CAN端口"=w2092, "命令"=w2108, "板号"=u8 0, "命令序号"=w2096, "输入数据"=w2110) -> ()  [unwired: 1 in, 12 out]
                      }
                    }
                  }
                }
              }
            }
          }
          event "风机": Shortcut Menu Selection (User) {
            n590 = event-data() -> ("ItemTag"=w2113:string)  [unwired: 8 out]
            n591 = local read "强制操作"() -> (w2112:bool)
            n592 = case shown="真" w2112 {
              tunnel: w2113 -> [_ w2114]
              frame False {
              }
              frame True {
                n593 = case shown="\"强制闭合\"" w2114 {
                  frame "假", Default {
                  }
                  frame "强制闭合" {
                    n594 = local read "CAN卡类型"() -> (w2117:u32)
                    n595 = local read "设备索引号"() -> (w2116:u16)
                    n596 = local read "CAN端口"() -> (w2115:u16)
                    n597 = case shown="假" TRUE {
                      selector: TRUE -> [w2136 w2156]
                      tunnel: [w2135 w2155] -> _
                      tunnel: [w2123 w2143] -> _
                      tunnel: w2117 -> [w2121 w2141]
                      tunnel: w2116 -> [w2120 w2140]
                      tunnel: w2115 -> [w2119 w2139]
                      frame False {
                        w2131 = 256.0 ("y")
                        w2123 = u32 1 ("命令序号")
                        w2135 = u8 192 ("命令")
                        n598 = local read "动作保持时间"() -> (w2132:dbl)
                        n599 = Quotient & Remainder(x=w2132, y=w2131) -> (x-y*floor(x/y)=w2124:dbl, floor(x/y)=w2128:dbl)
                        n600 = Quotient & Remainder(x=w2128, y=w2131) -> (x-y*floor(x/y)=w2125:dbl, floor(x/y)=w2129:dbl)
                        n601 = Quotient & Remainder(x=w2129, y=w2131) -> (x-y*floor(x/y)=w2126:dbl, floor(x/y)=w2130:dbl)
                        n602 = Boolean To (0,1)(Boolean=w2136) -> (0, 1=w2133:i16)
                        n603 = Quotient & Remainder(x=w2130, y=w2131) -> (x-y*floor(x/y)=w2127:dbl)  [unwired: 1 out]
                        n604 = Build Array(i16 6 ("元素"), w2133, w2127, w2126, w2125, w2124, 0.0 ("元素")) -> (w2137:dbl[])
                        n605 = call "多帧发送机制(EV05).vi"("can卡类型"=w2121, "设备索引号"=w2120, "CAN端口"=w2119, "命令"=w2135, "板号"=u8 0, "命令序号"=w2123, "输入数据"=w2137) -> ()  [unwired: 1 in, 12 out]
                      }
                      frame True {
                        w2151 = 256.0 ("y")
                        w2143 = u32 1 ("命令序号")
                        w2155 = u8 192 ("命令")
                        n606 = local read "动作保持时间"() -> (w2152:dbl)
                        n607 = Quotient & Remainder(x=w2152, y=w2151) -> (x-y*floor(x/y)=w2144:dbl, floor(x/y)=w2148:dbl)
                        n608 = Quotient & Remainder(x=w2148, y=w2151) -> (x-y*floor(x/y)=w2145:dbl, floor(x/y)=w2149:dbl)
                        n609 = Quotient & Remainder(x=w2149, y=w2151) -> (x-y*floor(x/y)=w2146:dbl, floor(x/y)=w2150:dbl)
                        n610 = Boolean To (0,1)(Boolean=w2156) -> (0, 1=w2153:i16)
                        n611 = Quotient & Remainder(x=w2150, y=w2151) -> (x-y*floor(x/y)=w2147:dbl)  [unwired: 1 out]
                        n612 = Build Array(i16 6 ("元素"), w2153, w2147, w2146, w2145, w2144, 0.0 ("元素")) -> (w2157:dbl[])
                        n613 = call "多帧发送机制(EV05).vi"("can卡类型"=w2141, "设备索引号"=w2140, "CAN端口"=w2139, "命令"=w2155, "板号"=u8 0, "命令序号"=w2143, "输入数据"=w2157) -> ()  [unwired: 1 in, 12 out]
                      }
                    }
                  }
                  frame "强制断开" {
                    n614 = local read "CAN卡类型"() -> (w2161:u32)
                    n615 = local read "设备索引号"() -> (w2160:u16)
                    n616 = local read "CAN端口"() -> (w2159:u16)
                    n617 = case shown="假" FALSE {
                      selector: FALSE -> [w2180 w2200]
                      tunnel: [w2179 w2199] -> _
                      tunnel: [w2167 w2187] -> _
                      tunnel: w2161 -> [w2165 w2185]
                      tunnel: w2160 -> [w2164 w2184]
                      tunnel: w2159 -> [w2163 w2183]
                      frame False {
                        w2175 = 256.0 ("y")
                        w2167 = u32 1 ("命令序号")
                        w2179 = u8 192 ("命令")
                        n618 = local read "动作保持时间"() -> (w2176:dbl)
                        n619 = Quotient & Remainder(x=w2176, y=w2175) -> (x-y*floor(x/y)=w2168:dbl, floor(x/y)=w2172:dbl)
                        n620 = Quotient & Remainder(x=w2172, y=w2175) -> (x-y*floor(x/y)=w2169:dbl, floor(x/y)=w2173:dbl)
                        n621 = Quotient & Remainder(x=w2173, y=w2175) -> (x-y*floor(x/y)=w2170:dbl, floor(x/y)=w2174:dbl)
                        n622 = Boolean To (0,1)(Boolean=w2180) -> (0, 1=w2177:i16)
                        n623 = Quotient & Remainder(x=w2174, y=w2175) -> (x-y*floor(x/y)=w2171:dbl)  [unwired: 1 out]
                        n624 = Build Array(i16 6 ("元素"), w2177, w2171, w2170, w2169, w2168, 0.0 ("元素")) -> (w2181:dbl[])
                        n625 = call "多帧发送机制(EV05).vi"("can卡类型"=w2165, "设备索引号"=w2164, "CAN端口"=w2163, "命令"=w2179, "板号"=u8 0, "命令序号"=w2167, "输入数据"=w2181) -> ()  [unwired: 1 in, 12 out]
                      }
                      frame True {
                        w2195 = 256.0 ("y")
                        w2187 = u32 1 ("命令序号")
                        w2199 = u8 192 ("命令")
                        n626 = local read "动作保持时间"() -> (w2196:dbl)
                        n627 = Quotient & Remainder(x=w2196, y=w2195) -> (x-y*floor(x/y)=w2188:dbl, floor(x/y)=w2192:dbl)
                        n628 = Quotient & Remainder(x=w2192, y=w2195) -> (x-y*floor(x/y)=w2189:dbl, floor(x/y)=w2193:dbl)
                        n629 = Quotient & Remainder(x=w2193, y=w2195) -> (x-y*floor(x/y)=w2190:dbl, floor(x/y)=w2194:dbl)
                        n630 = Boolean To (0,1)(Boolean=w2200) -> (0, 1=w2197:i16)
                        n631 = Quotient & Remainder(x=w2194, y=w2195) -> (x-y*floor(x/y)=w2191:dbl)  [unwired: 1 out]
                        n632 = Build Array(i16 6 ("元素"), w2197, w2191, w2190, w2189, w2188, 0.0 ("元素")) -> (w2201:dbl[])
                        n633 = call "多帧发送机制(EV05).vi"("can卡类型"=w2185, "设备索引号"=w2184, "CAN端口"=w2183, "命令"=w2199, "板号"=u8 0, "命令序号"=w2187, "输入数据"=w2201) -> ()  [unwired: 1 in, 12 out]
                      }
                    }
                  }
                }
              }
            }
          }
          event "充电": Shortcut Menu Selection (User) {
            n634 = event-data() -> ("ItemTag"=w2204:string)  [unwired: 8 out]
            n635 = local read "强制操作"() -> (w2203:bool)
            n636 = case shown="真" w2203 {
              tunnel: w2204 -> [_ w2205]
              frame False {
              }
              frame True {
                n637 = case shown="\"强制断开\"" w2205 {
                  frame "假", Default {
                  }
                  frame "强制闭合" {
                    n638 = local read "CAN卡类型"() -> (w2208:u32)
                    n639 = local read "设备索引号"() -> (w2207:u16)
                    n640 = local read "CAN端口"() -> (w2206:u16)
                    n641 = case shown="真" TRUE {
                      selector: TRUE -> [w2227 w2247]
                      tunnel: [w2226 w2246] -> _
                      tunnel: [w2214 w2234] -> _
                      tunnel: w2208 -> [w2212 w2232]
                      tunnel: w2207 -> [w2211 w2231]
                      tunnel: w2206 -> [w2210 w2230]
                      frame False {
                        w2222 = 256.0 ("y")
                        w2214 = u32 1 ("命令序号")
                        w2226 = u8 192 ("命令")
                        n642 = local read "动作保持时间"() -> (w2223:dbl)
                        n643 = Quotient & Remainder(x=w2223, y=w2222) -> (x-y*floor(x/y)=w2215:dbl, floor(x/y)=w2219:dbl)
                        n644 = Quotient & Remainder(x=w2219, y=w2222) -> (x-y*floor(x/y)=w2216:dbl, floor(x/y)=w2220:dbl)
                        n645 = Quotient & Remainder(x=w2220, y=w2222) -> (x-y*floor(x/y)=w2217:dbl, floor(x/y)=w2221:dbl)
                        n646 = Boolean To (0,1)(Boolean=w2227) -> (0, 1=w2224:i16)
                        n647 = Quotient & Remainder(x=w2221, y=w2222) -> (x-y*floor(x/y)=w2218:dbl)  [unwired: 1 out]
                        n648 = Build Array(i16 5 ("元素"), w2224, w2218, w2217, w2216, w2215, 0.0 ("元素")) -> (w2228:dbl[])
                        n649 = call "多帧发送机制(EV05).vi"("can卡类型"=w2212, "设备索引号"=w2211, "CAN端口"=w2210, "命令"=w2226, "板号"=u8 0, "命令序号"=w2214, "输入数据"=w2228) -> ()  [unwired: 1 in, 12 out]
                      }
                      frame True {
                        w2242 = 256.0 ("y")
                        w2234 = u32 1 ("命令序号")
                        w2246 = u8 192 ("命令")
                        n650 = local read "动作保持时间"() -> (w2243:dbl)
                        n651 = Quotient & Remainder(x=w2243, y=w2242) -> (x-y*floor(x/y)=w2235:dbl, floor(x/y)=w2239:dbl)
                        n652 = Quotient & Remainder(x=w2239, y=w2242) -> (x-y*floor(x/y)=w2236:dbl, floor(x/y)=w2240:dbl)
                        n653 = Quotient & Remainder(x=w2240, y=w2242) -> (x-y*floor(x/y)=w2237:dbl, floor(x/y)=w2241:dbl)
                        n654 = Boolean To (0,1)(Boolean=w2247) -> (0, 1=w2244:i16)
                        n655 = Quotient & Remainder(x=w2241, y=w2242) -> (x-y*floor(x/y)=w2238:dbl)  [unwired: 1 out]
                        n656 = Build Array(i16 5 ("元素"), w2244, w2238, w2237, w2236, w2235, 0.0 ("元素")) -> (w2248:dbl[])
                        n657 = call "多帧发送机制(EV05).vi"("can卡类型"=w2232, "设备索引号"=w2231, "CAN端口"=w2230, "命令"=w2246, "板号"=u8 0, "命令序号"=w2234, "输入数据"=w2248) -> ()  [unwired: 1 in, 12 out]
                      }
                    }
                  }
                  frame "强制断开" {
                    n658 = local read "CAN卡类型"() -> (w2252:u32)
                    n659 = local read "设备索引号"() -> (w2251:u16)
                    n660 = local read "CAN端口"() -> (w2250:u16)
                    n661 = case shown="真" FALSE {
                      selector: FALSE -> [w2271 w2291]
                      tunnel: [w2270 w2290] -> _
                      tunnel: [w2258 w2278] -> _
                      tunnel: w2252 -> [w2256 w2276]
                      tunnel: w2251 -> [w2255 w2275]
                      tunnel: w2250 -> [w2254 w2274]
                      frame False {
                        w2266 = 256.0 ("y")
                        w2258 = u32 1 ("命令序号")
                        w2270 = u8 192 ("命令")
                        n662 = local read "动作保持时间"() -> (w2267:dbl)
                        n663 = Quotient & Remainder(x=w2267, y=w2266) -> (x-y*floor(x/y)=w2259:dbl, floor(x/y)=w2263:dbl)
                        n664 = Quotient & Remainder(x=w2263, y=w2266) -> (x-y*floor(x/y)=w2260:dbl, floor(x/y)=w2264:dbl)
                        n665 = Quotient & Remainder(x=w2264, y=w2266) -> (x-y*floor(x/y)=w2261:dbl, floor(x/y)=w2265:dbl)
                        n666 = Boolean To (0,1)(Boolean=w2271) -> (0, 1=w2268:i16)
                        n667 = Quotient & Remainder(x=w2265, y=w2266) -> (x-y*floor(x/y)=w2262:dbl)  [unwired: 1 out]
                        n668 = Build Array(i16 5 ("元素"), w2268, w2262, w2261, w2260, w2259, 0.0 ("元素")) -> (w2272:dbl[])
                        n669 = call "多帧发送机制(EV05).vi"("can卡类型"=w2256, "设备索引号"=w2255, "CAN端口"=w2254, "命令"=w2270, "板号"=u8 0, "命令序号"=w2258, "输入数据"=w2272) -> ()  [unwired: 1 in, 12 out]
                      }
                      frame True {
                        w2286 = 256.0 ("y")
                        w2278 = u32 1 ("命令序号")
                        w2290 = u8 192 ("命令")
                        n670 = local read "动作保持时间"() -> (w2287:dbl)
                        n671 = Quotient & Remainder(x=w2287, y=w2286) -> (x-y*floor(x/y)=w2279:dbl, floor(x/y)=w2283:dbl)
                        n672 = Quotient & Remainder(x=w2283, y=w2286) -> (x-y*floor(x/y)=w2280:dbl, floor(x/y)=w2284:dbl)
                        n673 = Quotient & Remainder(x=w2284, y=w2286) -> (x-y*floor(x/y)=w2281:dbl, floor(x/y)=w2285:dbl)
                        n674 = Boolean To (0,1)(Boolean=w2291) -> (0, 1=w2288:i16)
                        n675 = Quotient & Remainder(x=w2285, y=w2286) -> (x-y*floor(x/y)=w2282:dbl)  [unwired: 1 out]
                        n676 = Build Array(i16 5 ("元素"), w2288, w2282, w2281, w2280, w2279, 0.0 ("元素")) -> (w2292:dbl[])
                        n677 = call "多帧发送机制(EV05).vi"("can卡类型"=w2276, "设备索引号"=w2275, "CAN端口"=w2274, "命令"=w2290, "板号"=u8 0, "命令序号"=w2278, "输入数据"=w2292) -> ()  [unwired: 1 in, 12 out]
                      }
                    }
                  }
                }
              }
            }
          }
          event "System XY Graph": Mouse Move {
            n678 = event-data() -> ("Coords"=w2321:T3)  [unwired: 5 out]
            n679 = global read "从板全局变量.vi" "电池节数"() -> (w2295:u8[])
            n680 = global read "单体信息全局.vi" "单体数据"() -> (w2297:dbl[][])
            n681 = for {
              tunnel: w2295 -> [w2325] mode=indexing
              tunnel: w2297 -> [w2328]
              shift-right: [w2323] -> w2296
              shift-left: dbl[] [] -> [w2324]
              tunnel: w2295 -> [w2322]
              i -> [w2327]
              n682 = Greater Than 0?(x=w2325) -> (x > 0?=w2326:bool)
              n683 = case shown="真" w2326 {
                tunnel: w2328 -> [_ w2339]
                tunnel: w2327 -> [_ w2331]
                tunnel: w2325 -> [_ w2330]
                tunnel: w2324 -> [w2329 w2336]
                tunnel: [w2329 w2337] -> w2323
                tunnel: w2322 -> [_ w2334]
                frame False {
                }
                frame True {
                  n684 = Index Array(array=w2339, index (row)=w2331) -> (element=w2338:dbl[])  [unwired: 1 in]
                  n685 = Array Subset(array=w2338, length=w2330) -> (w2335:dbl[])  [unwired: 1 in]
                  n686 = Array Subset(array=w2334, length=w2331) -> (w2333:u8[])  [unwired: 1 in]
                  n687 = Add Array Elements(numeric array=w2333) -> (sum=w2332:u8)
                  n688 = Insert Into Array(array=w2336, index=w2332, new element=w2335) -> (w2337:dbl[])
                }
              }
            }
            n689 = property on="System XY Graph" class="XYGraph (严格)"() -> ("Plot Area Size"=w2315:T15, "Plot Bounds"=w2320:T16)  [unwired: 2 in, 2 out]
            n690 = Unbundle By Name(w2321) -> ("Horizontal"=w2312:i32)
            n691 = Unbundle By Name(w2320) -> ("Left"=w2313:i16)
            n692 = Unbundle By Name(w2315) -> ("Width"=w2314:u32)
            n693 = local read "大小"() -> (w2319:i32)
            n694 = Array Subset(array=w2296) -> (w2294:dbl[])  [unwired: 2 in]
            n695 = Subtract(x=w2312, y=w2313) -> (x-y=w2310:i32)
            n696 = Divide(x=w2314, y=w2319) -> (x/y=w2309:dbl)
            n697 = Multiply(x=w2309, y=0.6) -> (x*y=w2317:dbl)
            n698 = Divide(x=w2310, y=w2309) -> (x/y=w2304:dbl)
            n699 = Quotient & Remainder(x=w2310, y=w2309) -> (x-y*floor(x/y)=w2308:dbl, floor(x/y)=w2306:dbl)
            n700 = Round Toward -Infinity(1:w2304) -> (0:w2303:dbl)
            n701 = Divide(x=w2317, y=2.0) -> (x/y=w2307:dbl)
            n702 = Less Or Equal?(x=w2310, y=w2307) -> (x <= y?=w2311:bool)
            n703 = Increment(x=w2303) -> (x+1=w2301:dbl)
            n704 = Greater Or Equal?(x=w2308, y=w2307) -> ()  [unwired: 1 out]
            n705 = Decrement(x=w2301) -> (x-1=w2300:dbl)
            n706 = Number To Decimal String(number=w2301) -> (decimal integer string=w2302:string)  [unwired: 1 in]
            n707 = Increment(x=w2306) -> (x+1=w2305:dbl)
            n708 = case shown="假" w2311 {
              tunnel: w2305 -> [_ _]
              frame False {
              }
              frame True {
              }
            }
            n709 = property on="1:" class="DigNum (严格)"("Caption.Text"=w2302) -> ()  [unwired: 2 in, 2 out]
            n710 = Index Array(array=w2294, index=w2300) -> (element=w2299:dbl)
            n711 = local write "1:"(w2299) -> ()
          }
          event "System XY Graph 3": Mouse Move {
            w2347 = 20 ("y")
            n712 = event-data() -> ("Coords"=w2371:T3)  [unwired: 5 out]
            n713 = global read "从板全局变量.vi" "温度个数"() -> (w2342:u8[])
            n714 = global read "单体信息全局.vi" "温度数据"() -> (w2345:sgl[][])
            n715 = property on="System XY Graph 3" class="XYGraph (严格)"() -> ("Plot Area Size"=w2353:T15, "Plot Bounds"=w2352:T16)  [unwired: 2 in, 2 out]
            n716 = for {
              tunnel: w2342 -> [w2375] mode=indexing
              tunnel: w2345 -> [w2378]
              shift-right: [w2373] -> w2343
              shift-left: dbl[] [] -> [w2374]
              tunnel: w2342 -> [w2372]
              i -> [w2377]
              n717 = Greater Than 0?(x=w2375) -> (x > 0?=w2376:bool)
              n718 = case shown="假" w2376 {
                tunnel: w2378 -> [_ w2389]
                tunnel: w2377 -> [_ w2381]
                tunnel: w2375 -> [_ w2380]
                tunnel: w2374 -> [w2379 w2386]
                tunnel: [w2379 w2387] -> w2373
                tunnel: w2372 -> [_ w2384]
                frame False {
                }
                frame True {
                  n719 = Index Array(array=w2389, index (row)=w2381) -> (element=w2388:sgl[])  [unwired: 1 in]
                  n720 = Array Subset(array=w2388, length=w2380) -> (w2385:sgl[])  [unwired: 1 in]
                  n721 = Array Subset(array=w2384, length=w2381) -> (w2383:u8[])  [unwired: 1 in]
                  n722 = Add Array Elements(numeric array=w2383) -> (sum=w2382:u8)
                  n723 = Insert Into Array(array=w2386, index=w2382, new element=w2385) -> (w2387:dbl[])
                }
              }
            }
            n724 = local read "温度个数"() -> (w2348:i32)
            n725 = Unbundle By Name(w2371) -> ("Horizontal"=w2365:i32)
            n726 = Add Array Elements(numeric array=w2342) -> (sum=w2341:u8)
            n727 = Unbundle By Name(w2352) -> ("Left"=w2366:i16)
            n728 = Unbundle By Name(w2353) -> ("Width"=w2367:u32)
            n729 = Greater?(x=w2348, y=w2347) -> (0:w2349:bool)
            n730 = Select(t=w2348, s=w2349, f=w2347) -> (s? t:f=w2346:i32)
            n731 = Array Subset(array=w2343, length=w2341) -> (w2340:dbl[])  [unwired: 1 in]
            n732 = Subtract(x=w2365, y=w2366) -> (x-y=w2363:i32)
            n733 = Divide(x=w2367, y=w2346) -> (x/y=w2362:dbl)
            n734 = Multiply(x=w2362, y=0.6) -> (x*y=w2369:dbl)
            n735 = Divide(x=w2363, y=w2362) -> (x/y=w2357:dbl)
            n736 = Quotient & Remainder(x=w2363, y=w2362) -> (x-y*floor(x/y)=w2361:dbl, floor(x/y)=w2359:dbl)
            n737 = Round Toward -Infinity(1:w2357) -> (0:w2356:dbl)
            n738 = Divide(x=w2369, y=2.0) -> (x/y=w2360:dbl)
            n739 = Less Or Equal?(x=w2363, y=w2360) -> (x <= y?=w2364:bool)
            n740 = Increment(x=w2356) -> (x+1=w2355:dbl)
            n741 = Greater Or Equal?(x=w2361, y=w2360) -> ()  [unwired: 1 out]
            n742 = Decrement(x=w2355) -> (x-1=w2354:dbl)
            n743 = Number To Decimal String(number=w2355) -> (decimal integer string=w2351:string)  [unwired: 1 in]
            n744 = Increment(x=w2359) -> (x+1=w2358:dbl)
            n745 = case shown="真" w2364 {
              tunnel: w2358 -> [_ _]
              frame False {
              }
              frame True {
              }
            }
            n746 = property on="1:" class="DigNum (严格)"("Caption.Text"=w2351) -> ()  [unwired: 2 in, 2 out]
            n747 = property on="1: 2" class="DigNum (严格)"("Caption.Text"=w2351) -> ()  [unwired: 2 in, 2 out]
            n748 = Index Array(array=w2340, index=w2354) -> (element=w2350:dbl)
            n749 = local write "1: 2"(w2350) -> ()
          }
          event "System XY Graph 3": Shortcut Menu Selection (User) {
            n750 = event-data() -> ("ItemPath"=w2390:string)  [unwired: 8 out]
            n751 = case shown="\"查看温度详细信息\"" w2390 {
              frame "假", Default {
              }
              frame "查看温度详细信息" {
                n752 = stacked-sequence {
                  frame #0 {
                    w2391 = 2
                    n753 = property on="系统信息" class="Bool (严格)"("Disabled"=w2391) -> ()  [unwired: 2 in, 2 out]
                    n754 = property on="单箱信息" class="Bool (严格)"("Disabled"=w2391) -> ()  [unwired: 2 in, 2 out]
                    n755 = property on="诊断标定" class="Bool (严格)"("Disabled"=w2391) -> ()  [unwired: 2 in, 2 out]
                    n756 = property on="详细信息 4" class="Bool (严格)"("Disabled"=w2391) -> ()  [unwired: 2 in, 2 out]
                    n757 = property on="诊断标定 3" class="Bool (严格)"("Disabled"=w2391) -> ()  [unwired: 2 in, 2 out]
                    n758 = property on="单板信息 3" class="Bool (严格)"("Disabled"=w2391) -> ()  [unwired: 2 in, 2 out]
                  }
                  frame #1 {
                    n759 = local read "设备索引号"() -> (w2393:u16)
                    n760 = local read "CAN卡类型"() -> (w2394:u32)
                    n761 = local read "CAN端口"() -> (w2392:u16)
                    n762 = call "单体采集信息-new.vi"("can卡类型"=w2394, "设备索引号"=w2393, "CAN端口"=w2392) -> ()  [unwired: 3 in, 14 out]
                  }
                  frame #2 {
                    w2395 = 0
                    n763 = property on="系统信息" class="Bool (严格)"("Disabled"=w2395) -> ()  [unwired: 2 in, 2 out]
                    n764 = property on="单箱信息" class="Bool (严格)"("Disabled"=w2395) -> ()  [unwired: 2 in, 2 out]
                    n765 = property on="诊断标定" class="Bool (严格)"("Disabled"=w2395) -> ()  [unwired: 2 in, 2 out]
                    n766 = property on="详细信息 4" class="Bool (严格)"("Disabled"=w2395) -> ()  [unwired: 2 in, 2 out]
                    n767 = property on="诊断标定 3" class="Bool (严格)"("Disabled"=w2395) -> ()  [unwired: 2 in, 2 out]
                    n768 = property on="单板信息 3" class="Bool (严格)"("Disabled"=w2395) -> ()  [unwired: 2 in, 2 out]
                  }
                }
              }
            }
          }
          event "System XY Graph 3": Mouse Down {
            n769 = event-data() -> ("Coords"=→"坐标 2":T3)  [unwired: 8 out]
            n770 = property on="System XY Graph 3" class="XYGraph (严格)"() -> ("XScale.MarkerVals[]"=→"X标尺.刻度值[]":dbl[])  [unwired: 2 in, 2 out]
          }
          event "电压温度", "详细信息 3": Value Change {
            n771 = event-data() -> ("NewVal"=w2398:bool)  [unwired: 6 out]
            n772 = case shown="真" w2398 {
              frame False {
              }
              frame True {
                n773 = stacked-sequence {
                  frame #0 {
                    n774 = disable-structure shown="禁用" {
                      frame Disabled {
                        w2399 = 2
                        n775 = property on="系统信息" class="Bool (严格)"("Disabled"=w2399) -> ()  [unwired: 2 in, 2 out]
                        n776 = property on="单箱信息" class="Bool (严格)"("Disabled"=w2399) -> ()  [unwired: 2 in, 2 out]
                        n777 = property on="诊断标定" class="Bool (严格)"("Disabled"=w2399) -> ()  [unwired: 2 in, 2 out]
                        n778 = property on="详细信息 4" class="Bool (严格)"("Disabled"=w2399) -> ()  [unwired: 2 in, 2 out]
                        n779 = property on="诊断标定 3" class="Bool (严格)"("Disabled"=w2399) -> ()  [unwired: 2 in, 2 out]
                        n780 = property on="单板信息 3" class="Bool (严格)"("Disabled"=w2399) -> ()  [unwired: 2 in, 2 out]
                      }
                      frame Enabled {
                      }
                    }
                  }
                  frame #1 {
                    n781 = local read "设备索引号"() -> (w2401:u16)
                    n782 = local read "CAN卡类型"() -> (w2402:u32)
                    n783 = local read "CAN端口"() -> (w2400:u16)
                    n784 = call-by-ref "?"("can卡类型"=w2402, "设备索引号"=w2401, "CAN端口"=w2400) -> ()  [unwired: 19 in, 2 out]
                  }
                  frame #2 {
                    n785 = disable-structure shown="禁用" {
                      frame Disabled {
                        w2403 = 0
                        n786 = property on="系统信息" class="Bool (严格)"("Disabled"=w2403) -> ()  [unwired: 2 in, 2 out]
                        n787 = property on="单箱信息" class="Bool (严格)"("Disabled"=w2403) -> ()  [unwired: 2 in, 2 out]
                        n788 = property on="诊断标定" class="Bool (严格)"("Disabled"=w2403) -> ()  [unwired: 2 in, 2 out]
                        n789 = property on="详细信息 4" class="Bool (严格)"("Disabled"=w2403) -> ()  [unwired: 2 in, 2 out]
                        n790 = property on="诊断标定 3" class="Bool (严格)"("Disabled"=w2403) -> ()  [unwired: 2 in, 2 out]
                        n791 = property on="单板信息 3" class="Bool (严格)"("Disabled"=w2403) -> ()  [unwired: 2 in, 2 out]
                      }
                      frame Enabled {
                      }
                    }
                  }
                }
              }
            }
          }
          event "系统信息", "详细信息 4": Value Change {
            n792 = event-data() -> ("NewVal"=w2404:bool)  [unwired: 6 out]
            n793 = case shown="真" w2404 {
              frame False {
              }
              frame True {
                n794 = stacked-sequence {
                  frame #0 {
                    n795 = disable-structure shown="禁用" {
                      frame Disabled {
                        w2405 = 2
                        n796 = property on="单箱信息" class="Bool (严格)"("Disabled"=w2405) -> ()  [unwired: 2 in, 2 out]
                        n797 = property on="诊断标定" class="Bool (严格)"("Disabled"=w2405) -> ()  [unwired: 2 in, 2 out]
                        n798 = property on="电压温度" class="Bool (严格)"("Disabled"=w2405) -> ()  [unwired: 2 in, 2 out]
                        n799 = property on="详细信息 3" class="Bool (严格)"("Disabled"=w2405) -> ()  [unwired: 2 in, 2 out]
                        n800 = property on="诊断标定 3" class="Bool (严格)"("Disabled"=w2405) -> ()  [unwired: 2 in, 2 out]
                        n801 = property on="单板信息 3" class="Bool (严格)"("Disabled"=w2405) -> ()  [unwired: 2 in, 2 out]
                      }
                      frame Enabled {
                      }
                    }
                  }
                  frame #1 {
                    n802 = local read "设备索引号"() -> (w2408:u16)
                    n803 = local read "CAN卡类型"() -> (w2409:u32)
                    n804 = local read "CAN端口"() -> (w2407:u16)
                    n805 = call-by-ref "?"("can卡类型"=w2409, "设备索引号"=w2408, "CAN端口"=w2407, "主界面选项 3"=enum32{"单选选项1", "单选选项2 2", "单选选项2 3", "单选选项2 4"}."单选选项1") -> ()  [unwired: 18 in, 2 out]
                  }
                  frame #2 {
                    n806 = disable-structure shown="禁用" {
                      frame Disabled {
                        w2410 = 0
                        n807 = property on="单箱信息" class="Bool (严格)"("Disabled"=w2410) -> ()  [unwired: 2 in, 2 out]
                        n808 = property on="诊断标定" class="Bool (严格)"("Disabled"=w2410) -> ()  [unwired: 2 in, 2 out]
                        n809 = property on="电压温度" class="Bool (严格)"("Disabled"=w2410) -> ()  [unwired: 2 in, 2 out]
                        n810 = property on="详细信息 3" class="Bool (严格)"("Disabled"=w2410) -> ()  [unwired: 2 in, 2 out]
                        n811 = property on="诊断标定 3" class="Bool (严格)"("Disabled"=w2410) -> ()  [unwired: 2 in, 2 out]
                        n812 = property on="单板信息 3" class="Bool (严格)"("Disabled"=w2410) -> ()  [unwired: 2 in, 2 out]
                      }
                      frame Enabled {
                      }
                    }
                  }
                }
              }
            }
          }
          event Menu Selection (User) {
            n813 = event-data() -> ("ItemTag"=w2411:string)  [unwired: 7 out]
            n814 = case shown="\"软件注册\"" w2411 {
              frame "假", Default {
              }
              frame "参数生成器" {
                n815 = local read "参数生成"() -> (w2412:bool)
                n816 = case shown="真" w2412 {
                  frame False {
                  }
                  frame True {
                    n817 = stacked-sequence {
                      frame #0 {
                        n818 = property class="VI"("FP.State"=T10."Standard" ("前面板窗口:状态")) -> ()  [unwired: 2 in, 2 out]
                      }
                      frame #1 {
                        n819 = call-by-ref "?"() -> ()  [unwired: 14 in, 2 out]
                      }
                      frame #2 {
                        n820 = property class="VI"("FP.State"=T10."Standard" ("前面板窗口:状态")) -> ()  [unwired: 2 in, 2 out]
                      }
                    }
                  }
                }
              }
              frame "CAN设置" {
                n821 = call-by-ref "?"() -> ("取消"=w2415:bool, "工作方式 2"=w2416:u8, "CAN卡类型 2"=w2422:u32, "设备索引号 2"=w2421:u16, "波特率 2"=w2420:T12, "CAN端口 2"=w2419:u16, "E-U_baud 2"=w2418:u32, "滤波方式 2"=w2417:u8)  [unwired: 13 in, 3 out]
                n822 = case shown="假" w2415 {
                  tunnel: w2417 -> [w2429 _]
                  tunnel: w2416 -> [w2428 _]
                  tunnel: w2420 -> [w2427 _]
                  tunnel: w2418 -> [w2426 _]
                  tunnel: w2422 -> [w2425 _]
                  tunnel: w2421 -> [w2424 _]
                  tunnel: w2419 -> [w2423 _]
                  frame False {
                    n823 = local write "CAN端口"(w2423) -> ()
                    n824 = local write "E-U_baud"(w2426) -> ()
                    n825 = local write "CAN卡类型"(w2425) -> ()
                    n826 = local write "滤波方式"(w2429) -> ()
                    n827 = local write "工作方式"(w2428) -> ()
                    n828 = local write "设备索引号"(w2424) -> ()
                    n829 = local write "波特率"(w2427) -> ()
                    n830 = global write "EV05全局变量1.vi" "设备索引号"(w2424) -> ()
                    n831 = global write "EV05全局变量1.vi" "CAN卡类型"(w2425) -> ()
                    n832 = global write "EV05全局变量1.vi" "波特率"(w2427) -> ()
                    n833 = global write "EV05全局变量1.vi" "CAN端口"(w2423) -> ()
                    n834 = global write "EV05全局变量1.vi" "E-U_baud"(w2426) -> ()
                  }
                  frame True {
                  }
                }
              }
              frame "测试配置生成" {
                n835 = call-by-ref "?"() -> ()  [unwired: 14 in, 2 out]
              }
              frame "模拟发送" {
                n836 = local write "模拟发送"(TRUE ("模拟发送")) -> ()
              }
              frame "刷新界面" {
                w2435 = 0.0 ("CC")
                w2436 = FALSE ("DI3")
                w2437 = 0.0 ("外总压")
                w2438 = u16 0 ("总电压进度")
                w2440 = "" ("BMS时间")
                w2441 = 0.0 ("总电压")
                n837 = global write "电池信息全局变量.vi" "允许保存数据"(FALSE ("允许保存数据")) -> ()
                n838 = local write "总电压(V)"(w2441) -> ()
                n839 = local write "总电流(A)"(w2441) -> ()
                n840 = local write "SOH"(w2441) -> ()
                n841 = local write "SOC"(w2441) -> ()
                n842 = global write "电池信息全局变量.vi" "刷新计数"(0.0 ("刷新计数")) -> ()
                n843 = local write "SOC(黄)"(w2441) -> ()
                n844 = local write "SOC(红)"(w2441) -> ()
                n845 = local write "充电继电器"(w2441) -> ()
                n846 = local write "正级继电器"(w2441) -> ()
                n847 = local write "负级继电器"(w2441) -> ()
                n848 = local write "预充继电器"(w2441) -> ()
                n849 = local write "BMS时间"(w2440) -> ()
                n850 = local write "状态"(w2440) -> ()
                n851 = local write "系统运行模式"(w2440) -> ()
                n852 = local write "故障信息概况"(w2440) -> ()
                n853 = local write "LIFE"(w2440) -> ()
                n854 = local write "电池系统绝缘状态"(w2440) -> ()
                n855 = local write "次要参数"(T5 {"最高单体电压"=0.0, "最高电压位置"=0.0, "最低单体电压"=0.0, "最低电压位置"=0.0, "压差"=0.0, "最高单体温度"=0.0, "最高温度位置"=0.0, "最低单体温度"=0.0, "最低温度位置"=0.0, "温差"=0.0, "最高单体内阻"=0.0, "最高内阻位置"=0.0, "最低单体内阻"=0.0, "最低内阻位置"=0.0, "总内阻"=0.0, "协议是否公开"="", "协议版本号"="", "应用类型"="", "波特率"=""} ("次要参数")) -> ()
                n856 = local write "DI3"(w2436) -> ()
                n857 = local write "DI2"(w2436) -> ()
                n858 = local write "DI1"(w2436) -> ()
                n859 = local write "DI4"(w2436) -> ()
                n860 = local write "加热"(w2436) -> ()
                n861 = local write "DO2"(w2436) -> ()
                n862 = local write "风机"(w2436) -> ()
                n863 = local write "DO1"(w2436) -> ()
                n864 = local write "总电流进度"(w2438) -> ()
                n865 = local write "总电压进度"(w2438) -> ()
                n866 = local write "总电流(A)"(w2437) -> ()
                n867 = local write "平均电流"(w2437) -> ()
                n868 = local write "外总压"(w2437) -> ()
                n869 = local write "总电压(V)"(w2437) -> ()
                n870 = local write "CP"(w2435) -> ()
                n871 = local write "CC2"(w2435) -> ()
                n872 = local write "AI1"(w2435) -> ()
                n873 = local write "AI2"(w2435) -> ()
                n874 = local write "CC"(w2435) -> ()
                n875 = global write "单体信息全局.vi" "单体数据"(dbl[][] [[0.0, 0.0, 0.0, 0.0, 0.0, 0.0, 0.0, 0.0, 0.0, 0.0, 0.0, 0.0, 0.0, 0.0, 0.0, 0.0, 0.0, 0.0, 0.0, 0.0, 0.0, 0.0, 0.0, 0.0, 0.0, 0.0, 0.0, 0.0, 0.0, 0.0, 0.0, 0.0, 0.0, 0.0, 0.0, 0.0, 0.0, 0.0, 0.0, 0.0, 0.0, 0.0, 0.0, 0.0, 0.0, 0.0, 0.0, 0.0, 0.0, 0.0, 0.0, 0.0, 0.0, 0.0, 0.0, 0.0, 0.0, 0.0, 0.0, 0.0, 0.0], [0.0, 0.0, 0.0, 0.0, 0.0, 0.0, 0.0, 0.0, 0.0, 0.0, 0.0, 0.0, 0.0, 0.0, 0.0, 0.0, 0.0, 0.0, 0.0, 0.0, 0.0, 0.0, 0.0, 0.0, 0.0, 0.0, 0.0, 0.0, 0.0, 0.0, 0.0, 0.0, 0.0, 0.0, 0.0, 0.0, 0.0, 0.0, 0.0, 0.0, 0.0, 0.0, 0.0, 0.0, 0.0, 0.0, 0.0, 0.0, 0.0, 0.0, 0.0, 0.0, 0.0, 0.0, 0.0, 0.0, 0.0, 0.0, 0.0, 0.0, 0.0], [0.0, 0.0, 0.0, 0.0, 0.0, 0.0, 0.0, 0.0, 0.0, 0.0, 0.0, 0.0, 0.0, 0.0, 0.0, 0.0, 0.0, 0.0, 0.0, 0.0, 0.0, 0.0, 0.0, 0.0, 0.0, 0.0, 0.0, 0.0, 0.0, 0.0, 0.0, 0.0, 0.0, 0.0, 0.0, 0.0, 0.0, 0.0, 0.0, 0.0, 0.0, 0.0, 0.0, 0.0, 0.0, 0.0, 0.0, 0.0, 0.0, 0.0, 0.0, 0.0, 0.0, 0.0, 0.0, 0.0, 0.0, 0.0, 0.0, 0.0, 0.0], [0.0, 0.0, 0.0, 0.0, 0.0, 0.0, 0.0, 0.0, 0.0, 0.0, 0.0, 0.0, 0.0, 0.0, 0.0, 0.0, 0.0, 0.0, 0.0, 0.0, 0.0, 0.0, 0.0, 0.0, 0.0, 0.0, 0.0, 0.0, 0.0, 0.0, 0.0, 0.0, 0.0, 0.0, 0.0, 0.0, 0.0, 0.0, 0.0, 0.0, 0.0, 0.0, 0.0, 0.0, 0.0, 0.0, 0.0, 0.0, 0.0, 0.0, 0.0, 0.0, 0.0, 0.0, 0.0, 0.0, 0.0, 0.0, 0.0, 0.0, 0.0], [0.0, 0.0, 0.0, 0.0, 0.0, 0.0, 0.0, 0.0, 0.0, 0.0, 0.0, 0.0, 0.0, 0.0, 0.0, 0.0, 0.0, 0.0, 0.0, 0.0, 0.0, 0.0, 0.0, 0.0, 0.0, 0.0, 0.0, 0.0, 0.0, 0.0, 0.0, 0.0, 0.0, 0.0, 0.0, 0.0, 0.0, 0.0, 0.0, 0.0, 0.0, 0.0, 0.0, 0.0, 0.0, 0.0, 0.0, 0.0, 0.0, 0.0, 0.0, 0.0, 0.0, 0.0, 0.0, 0.0, 0.0, 0.0, 0.0, 0.0, 0.0], [0.0, 0.0, 0.0, 0.0, 0.0, 0.0, 0.0, 0.0, 0.0, 0.0, 0.0, 0.0, 0.0, 0.0, 0.0, 0.0, 0.0, 0.0, 0.0, 0.0, 0.0, 0.0, 0.0, 0.0, 0.0, 0.0, 0.0, 0.0, 0.0, 0.0, 0.0, 0.0, 0.0, 0.0, 0.0, 0.0, 0.0, 0.0, 0.0, 0.0, 0.0, 0.0, 0.0, 0.0, 0.0, 0.0, 0.0, 0.0, 0.0, 0.0, 0.0, 0.0, 0.0, 0.0, 0.0, 0.0, 0.0, 0.0, 0.0, 0.0, 0.0], [0.0, 0.0, 0.0, 0.0, 0.0, 0.0, 0.0, 0.0, 0.0, 0.0, 0.0, 0.0, 0.0, 0.0, 0.0, 0.0, 0.0, 0.0, 0.0, 0.0, 0.0, 0.0, 0.0, 0.0, 0.0, 0.0, 0.0, 0.0, 0.0, 0.0, 0.0, 0.0, 0.0, 0.0, 0.0, 0.0, 0.0, 0.0, 0.0, 0.0, 0.0, 0.0, 0.0, 0.0, 0.0, 0.0, 0.0, 0.0, 0.0, 0.0, 0.0, 0.0, 0.0, 0.0, 0.0, 0.0, 0.0, 0.0, 0.0, 0.0, 0.0], [0.0, 0.0, 0.0, 0.0, 0.0, 0.0, 0.0, 0.0, 0.0, 0.0, 0.0, 0.0, 0.0, 0.0, 0.0, 0.0, 0.0, 0.0, 0.0, 0.0, 0.0, 0.0, 0.0, 0.0, 0.0, 0.0, 0.0, 0.0, 0.0, 0.0, 0.0, 0.0, 0.0, 0.0, 0.0, 0.0, 0.0, 0.0, 0.0, 0.0, 0.0, 0.0, 0.0, 0.0, 0.0, 0.0, 0.0, 0.0, 0.0, 0.0, 0.0, 0.0, 0.0, 0.0, 0.0, 0.0, 0.0, 0.0, 0.0, 0.0, 0.0], [0.0, 0.0, 0.0, 0.0, 0.0, 0.0, 0.0, 0.0, 0.0, 0.0, 0.0, 0.0, 0.0, 0.0, 0.0, 0.0, 0.0, 0.0, 0.0, 0.0, 0.0, 0.0, 0.0, 0.0, 0.0, 0.0, 0.0, 0.0, 0.0, 0.0, 0.0, 0.0, 0.0, 0.0, 0.0, 0.0, 0.0, 0.0, 0.0, 0.0, 0.0, 0.0, 0.0, 0.0, 0.0, 0.0, 0.0, 0.0, 0.0, 0.0, 0.0, 0.0, 0.0, 0.0, 0.0, 0.0, 0.0, 0.0, 0.0, 0.0, 0.0], [0.0, 0.0, 0.0, 0.0, 0.0, 0.0, 0.0, 0.0, 0.0, 0.0, 0.0, 0.0, 0.0, 0.0, 0.0, 0.0, 0.0, 0.0, 0.0, 0.0, 0.0, 0.0, 0.0, 0.0, 0.0, 0.0, 0.0, 0.0, 0.0, 0.0, 0.0, 0.0, 0.0, 0.0, 0.0, 0.0, 0.0, 0.0, 0.0, 0.0, 0.0, 0.0, 0.0, 0.0, 0.0, 0.0, 0.0, 0.0, 0.0, 0.0, 0.0, 0.0, 0.0, 0.0, 0.0, 0.0, 0.0, 0.0, 0.0, 0.0, 0.0], [0.0, 0.0, 0.0, 0.0, 0.0, 0.0, 0.0, 0.0, 0.0, 0.0, 0.0, 0.0, 0.0, 0.0, 0.0, 0.0, 0.0, 0.0, 0.0, 0.0, 0.0, 0.0, 0.0, 0.0, 0.0, 0.0, 0.0, 0.0, 0.0, 0.0, 0.0, 0.0, 0.0, 0.0, 0.0, 0.0, 0.0, 0.0, 0.0, 0.0, 0.0, 0.0, 0.0, 0.0, 0.0, 0.0, 0.0, 0.0, 0.0, 0.0, 0.0, 0.0, 0.0, 0.0, 0.0, 0.0, 0.0, 0.0, 0.0, 0.0, 0.0], [0.0, 0.0, 0.0, 0.0, 0.0, 0.0, 0.0, 0.0, 0.0, 0.0, 0.0, 0.0, 0.0, 0.0, 0.0, 0.0, 0.0, 0.0, 0.0, 0.0, 0.0, 0.0, 0.0, 0.0, 0.0, 0.0, 0.0, 0.0, 0.0, 0.0, 0.0, 0.0, 0.0, 0.0, 0.0, 0.0, 0.0, 0.0, 0.0, 0.0, 0.0, 0.0, 0.0, 0.0, 0.0, 0.0, 0.0, 0.0, 0.0, 0.0, 0.0, 0.0, 0.0, 0.0, 0.0, 0.0, 0.0, 0.0, 0.0, 0.0, 0.0], [0.0, 0.0, 0.0, 0.0, 0.0, 0.0, 0.0, 0.0, 0.0, 0.0, 0.0, 0.0, 0.0, 0.0, 0.0, 0.0, 0.0, 0.0, 0.0, 0.0, 0.0, 0.0, 0.0, 0.0, 0.0, 0.0, 0.0, 0.0, 0.0, 0.0, 0.0, 0.0, 0.0, 0.0, 0.0, 0.0, 0.0, 0.0, 0.0, 0.0, 0.0, 0.0, 0.0, 0.0, 0.0, 0.0, 0.0, 0.0, 0.0, 0.0, 0.0, 0.0, 0.0, 0.0, 0.0, 0.0, 0.0, 0.0, 0.0, 0.0, 0.0], [0.0, 0.0, 0.0, 0.0, 0.0, 0.0, 0.0, 0.0, 0.0, 0.0, 0.0, 0.0, 0.0, 0.0, 0.0, 0.0, 0.0, 0.0, 0.0, 0.0, 0.0, 0.0, 0.0, 0.0, 0.0, 0.0, 0.0, 0.0, 0.0, 0.0, 0.0, 0.0, 0.0, 0.0, 0.0, 0.0, 0.0, 0.0, 0.0, 0.0, 0.0, 0.0, 0.0, 0.0, 0.0, 0.0, 0.0, 0.0, 0.0, 0.0, 0.0, 0.0, 0.0, 0.0, 0.0, 0.0, 0.0, 0.0, 0.0, 0.0, 0.0], [0.0, 0.0, 0.0, 0.0, 0.0, 0.0, 0.0, 0.0, 0.0, 0.0, 0.0, 0.0, 0.0, 0.0, 0.0, 0.0, 0.0, 0.0, 0.0, 0.0, 0.0, 0.0, 0.0, 0.0, 0.0, 0.0, 0.0, 0.0, 0.0, 0.0, 0.0, 0.0, 0.0, 0.0, 0.0, 0.0, 0.0, 0.0, 0.0, 0.0, 0.0, 0.0, 0.0, 0.0, 0.0, 0.0, 0.0, 0.0, 0.0, 0.0, 0.0, 0.0, 0.0, 0.0, 0.0, 0.0, 0.0, 0.0, 0.0, 0.0, 0.0], [0.0, 0.0, 0.0, 0.0, 0.0, 0.0, 0.0, 0.0, 0.0, 0.0, 0.0, 0.0, 0.0, 0.0, 0.0, 0.0, 0.0, 0.0, 0.0, 0.0, 0.0, 0.0, 0.0, 0.0, 0.0, 0.0, 0.0, 0.0, 0.0, 0.0, 0.0, 0.0, 0.0, 0.0, 0.0, 0.0, 0.0, 0.0, 0.0, 0.0, 0.0, 0.0, 0.0, 0.0, 0.0, 0.0, 0.0, 0.0, 0.0, 0.0, 0.0, 0.0, 0.0, 0.0, 0.0, 0.0, 0.0, 0.0, 0.0, 0.0, 0.0], [0.0, 0.0, 0.0, 0.0, 0.0, 0.0, 0.0, 0.0, 0.0, 0.0, 0.0, 0.0, 0.0, 0.0, 0.0, 0.0, 0.0, 0.0, 0.0, 0.0, 0.0, 0.0, 0.0, 0.0, 0.0, 0.0, 0.0, 0.0, 0.0, 0.0, 0.0, 0.0, 0.0, 0.0, 0.0, 0.0, 0.0, 0.0, 0.0, 0.0, 0.0, 0.0, 0.0, 0.0, 0.0, 0.0, 0.0, 0.0, 0.0, 0.0, 0.0, 0.0, 0.0, 0.0, 0.0, 0.0, 0.0, 0.0, 0.0, 0.0, 0.0], [0.0, 0.0, 0.0, 0.0, 0.0, 0.0, 0.0, 0.0, 0.0, 0.0, 0.0, 0.0, 0.0, 0.0, 0.0, 0.0, 0.0, 0.0, 0.0, 0.0, 0.0, 0.0, 0.0, 0.0, 0.0, 0.0, 0.0, 0.0, 0.0, 0.0, 0.0, 0.0, 0.0, 0.0, 0.0, 0.0, 0.0, 0.0, 0.0, 0.0, 0.0, 0.0, 0.0, 0.0, 0.0, 0.0, 0.0, 0.0, 0.0, 0.0, 0.0, 0.0, 0.0, 0.0, 0.0, 0.0, 0.0, 0.0, 0.0, 0.0, 0.0], [0.0, 0.0, 0.0, 0.0, 0.0, 0.0, 0.0, 0.0, 0.0, 0.0, 0.0, 0.0, 0.0, 0.0, 0.0, 0.0, 0.0, 0.0, 0.0, 0.0, 0.0, 0.0, 0.0, 0.0, 0.0, 0.0, 0.0, 0.0, 0.0, 0.0, 0.0, 0.0, 0.0, 0.0, 0.0, 0.0, 0.0, 0.0, 0.0, 0.0, 0.0, 0.0, 0.0, 0.0, 0.0, 0.0, 0.0, 0.0, 0.0, 0.0, 0.0, 0.0, 0.0, 0.0, 0.0, 0.0, 0.0, 0.0, 0.0, 0.0, 0.0], [0.0, 0.0, 0.0, 0.0, 0.0, 0.0, 0.0, 0.0, 0.0, 0.0, 0.0, 0.0, 0.0, 0.0, 0.0, 0.0, 0.0, 0.0, 0.0, 0.0, 0.0, 0.0, 0.0, 0.0, 0.0, 0.0, 0.0, 0.0, 0.0, 0.0, 0.0, 0.0, 0.0, 0.0, 0.0, 0.0, 0.0, 0.0, 0.0, 0.0, 0.0, 0.0, 0.0, 0.0, 0.0, 0.0, 0.0, 0.0, 0.0, 0.0, 0.0, 0.0, 0.0, 0.0, 0.0, 0.0, 0.0, 0.0, 0.0, 0.0, 0.0], [0.0, 0.0, 0.0, 0.0, 0.0, 0.0, 0.0, 0.0, 0.0, 0.0, 0.0, 0.0, 0.0, 0.0, 0.0, 0.0, 0.0, 0.0, 0.0, 0.0, 0.0, 0.0, 0.0, 0.0, 0.0, 0.0, 0.0, 0.0, 0.0, 0.0, 0.0, 0.0, 0.0, 0.0, 0.0, 0.0, 0.0, 0.0, 0.0, 0.0, 0.0, 0.0, 0.0, 0.0, 0.0, 0.0, 0.0, 0.0, 0.0, 0.0, 0.0, 0.0, 0.0, 0.0, 0.0, 0.0, 0.0, 0.0, 0.0, 0.0, 0.0], [0.0, 0.0, 0.0, 0.0, 0.0, 0.0, 0.0, 0.0, 0.0, 0.0, 0.0, 0.0, 0.0, 0.0, 0.0, 0.0, 0.0, 0.0, 0.0, 0.0, 0.0, 0.0, 0.0, 0.0, 0.0, 0.0, 0.0, 0.0, 0.0, 0.0, 0.0, 0.0, 0.0, 0.0, 0.0, 0.0, 0.0, 0.0, 0.0, 0.0, 0.0, 0.0, 0.0, 0.0, 0.0, 0.0, 0.0, 0.0, 0.0, 0.0, 0.0, 0.0, 0.0, 0.0, 0.0, 0.0, 0.0, 0.0, 0.0, 0.0, 0.0], [0.0, 0.0, 0.0, 0.0, 0.0, 0.0, 0.0, 0.0, 0.0, 0.0, 0.0, 0.0, 0.0, 0.0, 0.0, 0.0, 0.0, 0.0, 0.0, 0.0, 0.0, 0.0, 0.0, 0.0, 0.0, 0.0, 0.0, 0.0, 0.0, 0.0, 0.0, 0.0, 0.0, 0.0, 0.0, 0.0, 0.0, 0.0, 0.0, 0.0, 0.0, 0.0, 0.0, 0.0, 0.0, 0.0, 0.0, 0.0, 0.0, 0.0, 0.0, 0.0, 0.0, 0.0, 0.0, 0.0, 0.0, 0.0, 0.0, 0.0, 0.0], [0.0, 0.0, 0.0, 0.0, 0.0, 0.0, 0.0, 0.0, 0.0, 0.0, 0.0, 0.0, 0.0, 0.0, 0.0, 0.0, 0.0, 0.0, 0.0, 0.0, 0.0, 0.0, 0.0, 0.0, 0.0, 0.0, 0.0, 0.0, 0.0, 0.0, 0.0, 0.0, 0.0, 0.0, 0.0, 0.0, 0.0, 0.0, 0.0, 0.0, 0.0, 0.0, 0.0, 0.0, 0.0, 0.0, 0.0, 0.0, 0.0, 0.0, 0.0, 0.0, 0.0, 0.0, 0.0, 0.0, 0.0, 0.0, 0.0, 0.0, 0.0], [0.0, 0.0, 0.0, 0.0, 0.0, 0.0, 0.0, 0.0, 0.0, 0.0, 0.0, 0.0, 0.0, 0.0, 0.0, 0.0, 0.0, 0.0, 0.0, 0.0, 0.0, 0.0, 0.0, 0.0, 0.0, 0.0, 0.0, 0.0, 0.0, 0.0, 0.0, 0.0, 0.0, 0.0, 0.0, 0.0, 0.0, 0.0, 0.0, 0.0, 0.0, 0.0, 0.0, 0.0, 0.0, 0.0, 0.0, 0.0, 0.0, 0.0, 0.0, 0.0, 0.0, 0.0, 0.0, 0.0, 0.0, 0.0, 0.0, 0.0, 0.0], [0.0, 0.0, 0.0, 0.0, 0.0, 0.0, 0.0, 0.0, 0.0, 0.0, 0.0, 0.0, 0.0, 0.0, 0.0, 0.0, 0.0, 0.0, 0.0, 0.0, 0.0, 0.0, 0.0, 0.0, 0.0, 0.0, 0.0, 0.0, 0.0, 0.0, 0.0, 0.0, 0.0, 0.0, 0.0, 0.0, 0.0, 0.0, 0.0, 0.0, 0.0, 0.0, 0.0, 0.0, 0.0, 0.0, 0.0, 0.0, 0.0, 0.0, 0.0, 0.0, 0.0, 0.0, 0.0, 0.0, 0.0, 0.0, 0.0, 0.0, 0.0], [0.0, 0.0, 0.0, 0.0, 0.0, 0.0, 0.0, 0.0, 0.0, 0.0, 0.0, 0.0, 0.0, 0.0, 0.0, 0.0, 0.0, 0.0, 0.0, 0.0, 0.0, 0.0, 0.0, 0.0, 0.0, 0.0, 0.0, 0.0, 0.0, 0.0, 0.0, 0.0, 0.0, 0.0, 0.0, 0.0, 0.0, 0.0, 0.0, 0.0, 0.0, 0.0, 0.0, 0.0, 0.0, 0.0, 0.0, 0.0, 0.0, 0.0, 0.0, 0.0, 0.0, 0.0, 0.0, 0.0, 0.0, 0.0, 0.0, 0.0, 0.0], [0.0, 0.0, 0.0, 0.0, 0.0, 0.0, 0.0, 0.0, 0.0, 0.0, 0.0, 0.0, 0.0, 0.0, 0.0, 0.0, 0.0, 0.0, 0.0, 0.0, 0.0, 0.0, 0.0, 0.0, 0.0, 0.0, 0.0, 0.0, 0.0, 0.0, 0.0, 0.0, 0.0, 0.0, 0.0, 0.0, 0.0, 0.0, 0.0, 0.0, 0.0, 0.0, 0.0, 0.0, 0.0, 0.0, 0.0, 0.0, 0.0, 0.0, 0.0, 0.0, 0.0, 0.0, 0.0, 0.0, 0.0, 0.0, 0.0, 0.0, 0.0], [0.0, 0.0, 0.0, 0.0, 0.0, 0.0, 0.0, 0.0, 0.0, 0.0, 0.0, 0.0, 0.0, 0.0, 0.0, 0.0, 0.0, 0.0, 0.0, 0.0, 0.0, 0.0, 0.0, 0.0, 0.0, 0.0, 0.0, 0.0, 0.0, 0.0, 0.0, 0.0, 0.0, 0.0, 0.0, 0.0, 0.0, 0.0, 0.0, 0.0, 0.0, 0.0, 0.0, 0.0, 0.0, 0.0, 0.0, 0.0, 0.0, 0.0, 0.0, 0.0, 0.0, 0.0, 0.0, 0.0, 0.0, 0.0, 0.0, 0.0, 0.0], [0.0, 0.0, 0.0, 0.0, 0.0, 0.0, 0.0, 0.0, 0.0, 0.0, 0.0, 0.0, 0.0, 0.0, 0.0, 0.0, 0.0, 0.0, 0.0, 0.0, 0.0, 0.0, 0.0, 0.0, 0.0, 0.0, 0.0, 0.0, 0.0, 0.0, 0.0, 0.0, 0.0, 0.0, 0.0, 0.0, 0.0, 0.0, 0.0, 0.0, 0.0, 0.0, 0.0, 0.0, 0.0, 0.0, 0.0, 0.0, 0.0, 0.0, 0.0, 0.0, 0.0, 0.0, 0.0, 0.0, 0.0, 0.0, 0.0, 0.0, 0.0], [0.0, 0.0, 0.0, 0.0, 0.0, 0.0, 0.0, 0.0, 0.0, 0.0, 0.0, 0.0, 0.0, 0.0, 0.0, 0.0, 0.0, 0.0, 0.0, 0.0, 0.0, 0.0, 0.0, 0.0, 0.0, 0.0, 0.0, 0.0, 0.0, 0.0, 0.0, 0.0, 0.0, 0.0, 0.0, 0.0, 0.0, 0.0, 0.0, 0.0, 0.0, 0.0, 0.0, 0.0, 0.0, 0.0, 0.0, 0.0, 0.0, 0.0, 0.0, 0.0, 0.0, 0.0, 0.0, 0.0, 0.0, 0.0, 0.0, 0.0, 0.0]] ("单体数据")) -> ()
                n876 = global write "单体信息全局.vi" "温度数据"(dbl[][] [[0.0, 0.0, 0.0, 0.0, 0.0, 0.0, 0.0, 0.0, 0.0, 0.0, 0.0, 0.0, 0.0, 0.0, 0.0, 0.0, 0.0, 0.0, 0.0, 0.0, 0.0, 0.0, 0.0, 0.0, 0.0, 0.0, 0.0, 0.0, 0.0, 0.0, 0.0, 0.0, 0.0, 0.0, 0.0, 0.0, 0.0, 0.0, 0.0, 0.0, 0.0, 0.0, 0.0, 0.0, 0.0, 0.0, 0.0, 0.0, 0.0, 0.0, 0.0, 0.0, 0.0, 0.0, 0.0, 0.0, 0.0, 0.0, 0.0, 0.0, 0.0], [0.0, 0.0, 0.0, 0.0, 0.0, 0.0, 0.0, 0.0, 0.0, 0.0, 0.0, 0.0, 0.0, 0.0, 0.0, 0.0, 0.0, 0.0, 0.0, 0.0, 0.0, 0.0, 0.0, 0.0, 0.0, 0.0, 0.0, 0.0, 0.0, 0.0, 0.0, 0.0, 0.0, 0.0, 0.0, 0.0, 0.0, 0.0, 0.0, 0.0, 0.0, 0.0, 0.0, 0.0, 0.0, 0.0, 0.0, 0.0, 0.0, 0.0, 0.0, 0.0, 0.0, 0.0, 0.0, 0.0, 0.0, 0.0, 0.0, 0.0, 0.0], [0.0, 0.0, 0.0, 0.0, 0.0, 0.0, 0.0, 0.0, 0.0, 0.0, 0.0, 0.0, 0.0, 0.0, 0.0, 0.0, 0.0, 0.0, 0.0, 0.0, 0.0, 0.0, 0.0, 0.0, 0.0, 0.0, 0.0, 0.0, 0.0, 0.0, 0.0, 0.0, 0.0, 0.0, 0.0, 0.0, 0.0, 0.0, 0.0, 0.0, 0.0, 0.0, 0.0, 0.0, 0.0, 0.0, 0.0, 0.0, 0.0, 0.0, 0.0, 0.0, 0.0, 0.0, 0.0, 0.0, 0.0, 0.0, 0.0, 0.0, 0.0], [0.0, 0.0, 0.0, 0.0, 0.0, 0.0, 0.0, 0.0, 0.0, 0.0, 0.0, 0.0, 0.0, 0.0, 0.0, 0.0, 0.0, 0.0, 0.0, 0.0, 0.0, 0.0, 0.0, 0.0, 0.0, 0.0, 0.0, 0.0, 0.0, 0.0, 0.0, 0.0, 0.0, 0.0, 0.0, 0.0, 0.0, 0.0, 0.0, 0.0, 0.0, 0.0, 0.0, 0.0, 0.0, 0.0, 0.0, 0.0, 0.0, 0.0, 0.0, 0.0, 0.0, 0.0, 0.0, 0.0, 0.0, 0.0, 0.0, 0.0, 0.0], [0.0, 0.0, 0.0, 0.0, 0.0, 0.0, 0.0, 0.0, 0.0, 0.0, 0.0, 0.0, 0.0, 0.0, 0.0, 0.0, 0.0, 0.0, 0.0, 0.0, 0.0, 0.0, 0.0, 0.0, 0.0, 0.0, 0.0, 0.0, 0.0, 0.0, 0.0, 0.0, 0.0, 0.0, 0.0, 0.0, 0.0, 0.0, 0.0, 0.0, 0.0, 0.0, 0.0, 0.0, 0.0, 0.0, 0.0, 0.0, 0.0, 0.0, 0.0, 0.0, 0.0, 0.0, 0.0, 0.0, 0.0, 0.0, 0.0, 0.0, 0.0], [0.0, 0.0, 0.0, 0.0, 0.0, 0.0, 0.0, 0.0, 0.0, 0.0, 0.0, 0.0, 0.0, 0.0, 0.0, 0.0, 0.0, 0.0, 0.0, 0.0, 0.0, 0.0, 0.0, 0.0, 0.0, 0.0, 0.0, 0.0, 0.0, 0.0, 0.0, 0.0, 0.0, 0.0, 0.0, 0.0, 0.0, 0.0, 0.0, 0.0, 0.0, 0.0, 0.0, 0.0, 0.0, 0.0, 0.0, 0.0, 0.0, 0.0, 0.0, 0.0, 0.0, 0.0, 0.0, 0.0, 0.0, 0.0, 0.0, 0.0, 0.0], [0.0, 0.0, 0.0, 0.0, 0.0, 0.0, 0.0, 0.0, 0.0, 0.0, 0.0, 0.0, 0.0, 0.0, 0.0, 0.0, 0.0, 0.0, 0.0, 0.0, 0.0, 0.0, 0.0, 0.0, 0.0, 0.0, 0.0, 0.0, 0.0, 0.0, 0.0, 0.0, 0.0, 0.0, 0.0, 0.0, 0.0, 0.0, 0.0, 0.0, 0.0, 0.0, 0.0, 0.0, 0.0, 0.0, 0.0, 0.0, 0.0, 0.0, 0.0, 0.0, 0.0, 0.0, 0.0, 0.0, 0.0, 0.0, 0.0, 0.0, 0.0], [0.0, 0.0, 0.0, 0.0, 0.0, 0.0, 0.0, 0.0, 0.0, 0.0, 0.0, 0.0, 0.0, 0.0, 0.0, 0.0, 0.0, 0.0, 0.0, 0.0, 0.0, 0.0, 0.0, 0.0, 0.0, 0.0, 0.0, 0.0, 0.0, 0.0, 0.0, 0.0, 0.0, 0.0, 0.0, 0.0, 0.0, 0.0, 0.0, 0.0, 0.0, 0.0, 0.0, 0.0, 0.0, 0.0, 0.0, 0.0, 0.0, 0.0, 0.0, 0.0, 0.0, 0.0, 0.0, 0.0, 0.0, 0.0, 0.0, 0.0, 0.0], [0.0, 0.0, 0.0, 0.0, 0.0, 0.0, 0.0, 0.0, 0.0, 0.0, 0.0, 0.0, 0.0, 0.0, 0.0, 0.0, 0.0, 0.0, 0.0, 0.0, 0.0, 0.0, 0.0, 0.0, 0.0, 0.0, 0.0, 0.0, 0.0, 0.0, 0.0, 0.0, 0.0, 0.0, 0.0, 0.0, 0.0, 0.0, 0.0, 0.0, 0.0, 0.0, 0.0, 0.0, 0.0, 0.0, 0.0, 0.0, 0.0, 0.0, 0.0, 0.0, 0.0, 0.0, 0.0, 0.0, 0.0, 0.0, 0.0, 0.0, 0.0], [0.0, 0.0, 0.0, 0.0, 0.0, 0.0, 0.0, 0.0, 0.0, 0.0, 0.0, 0.0, 0.0, 0.0, 0.0, 0.0, 0.0, 0.0, 0.0, 0.0, 0.0, 0.0, 0.0, 0.0, 0.0, 0.0, 0.0, 0.0, 0.0, 0.0, 0.0, 0.0, 0.0, 0.0, 0.0, 0.0, 0.0, 0.0, 0.0, 0.0, 0.0, 0.0, 0.0, 0.0, 0.0, 0.0, 0.0, 0.0, 0.0, 0.0, 0.0, 0.0, 0.0, 0.0, 0.0, 0.0, 0.0, 0.0, 0.0, 0.0, 0.0], [0.0, 0.0, 0.0, 0.0, 0.0, 0.0, 0.0, 0.0, 0.0, 0.0, 0.0, 0.0, 0.0, 0.0, 0.0, 0.0, 0.0, 0.0, 0.0, 0.0, 0.0, 0.0, 0.0, 0.0, 0.0, 0.0, 0.0, 0.0, 0.0, 0.0, 0.0, 0.0, 0.0, 0.0, 0.0, 0.0, 0.0, 0.0, 0.0, 0.0, 0.0, 0.0, 0.0, 0.0, 0.0, 0.0, 0.0, 0.0, 0.0, 0.0, 0.0, 0.0, 0.0, 0.0, 0.0, 0.0, 0.0, 0.0, 0.0, 0.0, 0.0], [0.0, 0.0, 0.0, 0.0, 0.0, 0.0, 0.0, 0.0, 0.0, 0.0, 0.0, 0.0, 0.0, 0.0, 0.0, 0.0, 0.0, 0.0, 0.0, 0.0, 0.0, 0.0, 0.0, 0.0, 0.0, 0.0, 0.0, 0.0, 0.0, 0.0, 0.0, 0.0, 0.0, 0.0, 0.0, 0.0, 0.0, 0.0, 0.0, 0.0, 0.0, 0.0, 0.0, 0.0, 0.0, 0.0, 0.0, 0.0, 0.0, 0.0, 0.0, 0.0, 0.0, 0.0, 0.0, 0.0, 0.0, 0.0, 0.0, 0.0, 0.0], [0.0, 0.0, 0.0, 0.0, 0.0, 0.0, 0.0, 0.0, 0.0, 0.0, 0.0, 0.0, 0.0, 0.0, 0.0, 0.0, 0.0, 0.0, 0.0, 0.0, 0.0, 0.0, 0.0, 0.0, 0.0, 0.0, 0.0, 0.0, 0.0, 0.0, 0.0, 0.0, 0.0, 0.0, 0.0, 0.0, 0.0, 0.0, 0.0, 0.0, 0.0, 0.0, 0.0, 0.0, 0.0, 0.0, 0.0, 0.0, 0.0, 0.0, 0.0, 0.0, 0.0, 0.0, 0.0, 0.0, 0.0, 0.0, 0.0, 0.0, 0.0], [0.0, 0.0, 0.0, 0.0, 0.0, 0.0, 0.0, 0.0, 0.0, 0.0, 0.0, 0.0, 0.0, 0.0, 0.0, 0.0, 0.0, 0.0, 0.0, 0.0, 0.0, 0.0, 0.0, 0.0, 0.0, 0.0, 0.0, 0.0, 0.0, 0.0, 0.0, 0.0, 0.0, 0.0, 0.0, 0.0, 0.0, 0.0, 0.0, 0.0, 0.0, 0.0, 0.0, 0.0, 0.0, 0.0, 0.0, 0.0, 0.0, 0.0, 0.0, 0.0, 0.0, 0.0, 0.0, 0.0, 0.0, 0.0, 0.0, 0.0, 0.0], [0.0, 0.0, 0.0, 0.0, 0.0, 0.0, 0.0, 0.0, 0.0, 0.0, 0.0, 0.0, 0.0, 0.0, 0.0, 0.0, 0.0, 0.0, 0.0, 0.0, 0.0, 0.0, 0.0, 0.0, 0.0, 0.0, 0.0, 0.0, 0.0, 0.0, 0.0, 0.0, 0.0, 0.0, 0.0, 0.0, 0.0, 0.0, 0.0, 0.0, 0.0, 0.0, 0.0, 0.0, 0.0, 0.0, 0.0, 0.0, 0.0, 0.0, 0.0, 0.0, 0.0, 0.0, 0.0, 0.0, 0.0, 0.0, 0.0, 0.0, 0.0], [0.0, 0.0, 0.0, 0.0, 0.0, 0.0, 0.0, 0.0, 0.0, 0.0, 0.0, 0.0, 0.0, 0.0, 0.0, 0.0, 0.0, 0.0, 0.0, 0.0, 0.0, 0.0, 0.0, 0.0, 0.0, 0.0, 0.0, 0.0, 0.0, 0.0, 0.0, 0.0, 0.0, 0.0, 0.0, 0.0, 0.0, 0.0, 0.0, 0.0, 0.0, 0.0, 0.0, 0.0, 0.0, 0.0, 0.0, 0.0, 0.0, 0.0, 0.0, 0.0, 0.0, 0.0, 0.0, 0.0, 0.0, 0.0, 0.0, 0.0, 0.0], [0.0, 0.0, 0.0, 0.0, 0.0, 0.0, 0.0, 0.0, 0.0, 0.0, 0.0, 0.0, 0.0, 0.0, 0.0, 0.0, 0.0, 0.0, 0.0, 0.0, 0.0, 0.0, 0.0, 0.0, 0.0, 0.0, 0.0, 0.0, 0.0, 0.0, 0.0, 0.0, 0.0, 0.0, 0.0, 0.0, 0.0, 0.0, 0.0, 0.0, 0.0, 0.0, 0.0, 0.0, 0.0, 0.0, 0.0, 0.0, 0.0, 0.0, 0.0, 0.0, 0.0, 0.0, 0.0, 0.0, 0.0, 0.0, 0.0, 0.0, 0.0], [0.0, 0.0, 0.0, 0.0, 0.0, 0.0, 0.0, 0.0, 0.0, 0.0, 0.0, 0.0, 0.0, 0.0, 0.0, 0.0, 0.0, 0.0, 0.0, 0.0, 0.0, 0.0, 0.0, 0.0, 0.0, 0.0, 0.0, 0.0, 0.0, 0.0, 0.0, 0.0, 0.0, 0.0, 0.0, 0.0, 0.0, 0.0, 0.0, 0.0, 0.0, 0.0, 0.0, 0.0, 0.0, 0.0, 0.0, 0.0, 0.0, 0.0, 0.0, 0.0, 0.0, 0.0, 0.0, 0.0, 0.0, 0.0, 0.0, 0.0, 0.0], [0.0, 0.0, 0.0, 0.0, 0.0, 0.0, 0.0, 0.0, 0.0, 0.0, 0.0, 0.0, 0.0, 0.0, 0.0, 0.0, 0.0, 0.0, 0.0, 0.0, 0.0, 0.0, 0.0, 0.0, 0.0, 0.0, 0.0, 0.0, 0.0, 0.0, 0.0, 0.0, 0.0, 0.0, 0.0, 0.0, 0.0, 0.0, 0.0, 0.0, 0.0, 0.0, 0.0, 0.0, 0.0, 0.0, 0.0, 0.0, 0.0, 0.0, 0.0, 0.0, 0.0, 0.0, 0.0, 0.0, 0.0, 0.0, 0.0, 0.0, 0.0], [0.0, 0.0, 0.0, 0.0, 0.0, 0.0, 0.0, 0.0, 0.0, 0.0, 0.0, 0.0, 0.0, 0.0, 0.0, 0.0, 0.0, 0.0, 0.0, 0.0, 0.0, 0.0, 0.0, 0.0, 0.0, 0.0, 0.0, 0.0, 0.0, 0.0, 0.0, 0.0, 0.0, 0.0, 0.0, 0.0, 0.0, 0.0, 0.0, 0.0, 0.0, 0.0, 0.0, 0.0, 0.0, 0.0, 0.0, 0.0, 0.0, 0.0, 0.0, 0.0, 0.0, 0.0, 0.0, 0.0, 0.0, 0.0, 0.0, 0.0, 0.0], [0.0, 0.0, 0.0, 0.0, 0.0, 0.0, 0.0, 0.0, 0.0, 0.0, 0.0, 0.0, 0.0, 0.0, 0.0, 0.0, 0.0, 0.0, 0.0, 0.0, 0.0, 0.0, 0.0, 0.0, 0.0, 0.0, 0.0, 0.0, 0.0, 0.0, 0.0, 0.0, 0.0, 0.0, 0.0, 0.0, 0.0, 0.0, 0.0, 0.0, 0.0, 0.0, 0.0, 0.0, 0.0, 0.0, 0.0, 0.0, 0.0, 0.0, 0.0, 0.0, 0.0, 0.0, 0.0, 0.0, 0.0, 0.0, 0.0, 0.0, 0.0], [0.0, 0.0, 0.0, 0.0, 0.0, 0.0, 0.0, 0.0, 0.0, 0.0, 0.0, 0.0, 0.0, 0.0, 0.0, 0.0, 0.0, 0.0, 0.0, 0.0, 0.0, 0.0, 0.0, 0.0, 0.0, 0.0, 0.0, 0.0, 0.0, 0.0, 0.0, 0.0, 0.0, 0.0, 0.0, 0.0, 0.0, 0.0, 0.0, 0.0, 0.0, 0.0, 0.0, 0.0, 0.0, 0.0, 0.0, 0.0, 0.0, 0.0, 0.0, 0.0, 0.0, 0.0, 0.0, 0.0, 0.0, 0.0, 0.0, 0.0, 0.0], [0.0, 0.0, 0.0, 0.0, 0.0, 0.0, 0.0, 0.0, 0.0, 0.0, 0.0, 0.0, 0.0, 0.0, 0.0, 0.0, 0.0, 0.0, 0.0, 0.0, 0.0, 0.0, 0.0, 0.0, 0.0, 0.0, 0.0, 0.0, 0.0, 0.0, 0.0, 0.0, 0.0, 0.0, 0.0, 0.0, 0.0, 0.0, 0.0, 0.0, 0.0, 0.0, 0.0, 0.0, 0.0, 0.0, 0.0, 0.0, 0.0, 0.0, 0.0, 0.0, 0.0, 0.0, 0.0, 0.0, 0.0, 0.0, 0.0, 0.0, 0.0], [0.0, 0.0, 0.0, 0.0, 0.0, 0.0, 0.0, 0.0, 0.0, 0.0, 0.0, 0.0, 0.0, 0.0, 0.0, 0.0, 0.0, 0.0, 0.0, 0.0, 0.0, 0.0, 0.0, 0.0, 0.0, 0.0, 0.0, 0.0, 0.0, 0.0, 0.0, 0.0, 0.0, 0.0, 0.0, 0.0, 0.0, 0.0, 0.0, 0.0, 0.0, 0.0, 0.0, 0.0, 0.0, 0.0, 0.0, 0.0, 0.0, 0.0, 0.0, 0.0, 0.0, 0.0, 0.0, 0.0, 0.0, 0.0, 0.0, 0.0, 0.0], [0.0, 0.0, 0.0, 0.0, 0.0, 0.0, 0.0, 0.0, 0.0, 0.0, 0.0, 0.0, 0.0, 0.0, 0.0, 0.0, 0.0, 0.0, 0.0, 0.0, 0.0, 0.0, 0.0, 0.0, 0.0, 0.0, 0.0, 0.0, 0.0, 0.0, 0.0, 0.0, 0.0, 0.0, 0.0, 0.0, 0.0, 0.0, 0.0, 0.0, 0.0, 0.0, 0.0, 0.0, 0.0, 0.0, 0.0, 0.0, 0.0, 0.0, 0.0, 0.0, 0.0, 0.0, 0.0, 0.0, 0.0, 0.0, 0.0, 0.0, 0.0], [0.0, 0.0, 0.0, 0.0, 0.0, 0.0, 0.0, 0.0, 0.0, 0.0, 0.0, 0.0, 0.0, 0.0, 0.0, 0.0, 0.0, 0.0, 0.0, 0.0, 0.0, 0.0, 0.0, 0.0, 0.0, 0.0, 0.0, 0.0, 0.0, 0.0, 0.0, 0.0, 0.0, 0.0, 0.0, 0.0, 0.0, 0.0, 0.0, 0.0, 0.0, 0.0, 0.0, 0.0, 0.0, 0.0, 0.0, 0.0, 0.0, 0.0, 0.0, 0.0, 0.0, 0.0, 0.0, 0.0, 0.0, 0.0, 0.0, 0.0, 0.0], [0.0, 0.0, 0.0, 0.0, 0.0, 0.0, 0.0, 0.0, 0.0, 0.0, 0.0, 0.0, 0.0, 0.0, 0.0, 0.0, 0.0, 0.0, 0.0, 0.0, 0.0, 0.0, 0.0, 0.0, 0.0, 0.0, 0.0, 0.0, 0.0, 0.0, 0.0, 0.0, 0.0, 0.0, 0.0, 0.0, 0.0, 0.0, 0.0, 0.0, 0.0, 0.0, 0.0, 0.0, 0.0, 0.0, 0.0, 0.0, 0.0, 0.0, 0.0, 0.0, 0.0, 0.0, 0.0, 0.0, 0.0, 0.0, 0.0, 0.0, 0.0], [0.0, 0.0, 0.0, 0.0, 0.0, 0.0, 0.0, 0.0, 0.0, 0.0, 0.0, 0.0, 0.0, 0.0, 0.0, 0.0, 0.0, 0.0, 0.0, 0.0, 0.0, 0.0, 0.0, 0.0, 0.0, 0.0, 0.0, 0.0, 0.0, 0.0, 0.0, 0.0, 0.0, 0.0, 0.0, 0.0, 0.0, 0.0, 0.0, 0.0, 0.0, 0.0, 0.0, 0.0, 0.0, 0.0, 0.0, 0.0, 0.0, 0.0, 0.0, 0.0, 0.0, 0.0, 0.0, 0.0, 0.0, 0.0, 0.0, 0.0, 0.0], [0.0, 0.0, 0.0, 0.0, 0.0, 0.0, 0.0, 0.0, 0.0, 0.0, 0.0, 0.0, 0.0, 0.0, 0.0, 0.0, 0.0, 0.0, 0.0, 0.0, 0.0, 0.0, 0.0, 0.0, 0.0, 0.0, 0.0, 0.0, 0.0, 0.0, 0.0, 0.0, 0.0, 0.0, 0.0, 0.0, 0.0, 0.0, 0.0, 0.0, 0.0, 0.0, 0.0, 0.0, 0.0, 0.0, 0.0, 0.0, 0.0, 0.0, 0.0, 0.0, 0.0, 0.0, 0.0, 0.0, 0.0, 0.0, 0.0, 0.0, 0.0], [0.0, 0.0, 0.0, 0.0, 0.0, 0.0, 0.0, 0.0, 0.0, 0.0, 0.0, 0.0, 0.0, 0.0, 0.0, 0.0, 0.0, 0.0, 0.0, 0.0, 0.0, 0.0, 0.0, 0.0, 0.0, 0.0, 0.0, 0.0, 0.0, 0.0, 0.0, 0.0, 0.0, 0.0, 0.0, 0.0, 0.0, 0.0, 0.0, 0.0, 0.0, 0.0, 0.0, 0.0, 0.0, 0.0, 0.0, 0.0, 0.0, 0.0, 0.0, 0.0, 0.0, 0.0, 0.0, 0.0, 0.0, 0.0, 0.0, 0.0, 0.0], [0.0, 0.0, 0.0, 0.0, 0.0, 0.0, 0.0, 0.0, 0.0, 0.0, 0.0, 0.0, 0.0, 0.0, 0.0, 0.0, 0.0, 0.0, 0.0, 0.0, 0.0, 0.0, 0.0, 0.0, 0.0, 0.0, 0.0, 0.0, 0.0, 0.0, 0.0, 0.0, 0.0, 0.0, 0.0, 0.0, 0.0, 0.0, 0.0, 0.0, 0.0, 0.0, 0.0, 0.0, 0.0, 0.0, 0.0, 0.0, 0.0, 0.0, 0.0, 0.0, 0.0, 0.0, 0.0, 0.0, 0.0, 0.0, 0.0, 0.0, 0.0]] ("单体数据")) -> ()
              }
              frame "软件注册" {
                n877 = call-by-ref "?"() -> ()  [unwired: 13 in, 2 out]
              }
              frame "退出" {
                n878 = local read "设备索引号"() -> (w2443:u16)
                n879 = local read "CAN卡类型"() -> (w2444:u32)
                n880 = local read "工作方式"() -> (w2446:u8)
                n881 = local read "滤波方式"() -> (w2445:u8)
                n882 = local read "CAN端口"() -> (w2442:u16)
                n883 = call-by-ref "?"("CAN卡类型"=w2444, "设备索引号"=w2443, "CAN端口"=w2442, "操作类型"=enum16{"初始化CAN", "关闭CAN"}."关闭CAN", "滤波方式"=w2445, "簇"=T14 {"打开CAN"=FALSE, "初始化CAN"=FALSE, "开始CAN"=FALSE, "重启"=FALSE, "关闭CAN"=TRUE}, "工作方式"=w2446) -> ()  [unwired: 12 in, 5 out]
              }
            }
          }
          event "CAN连接": Shortcut Menu Selection (User) {
            n884 = event-data() -> ()  [unwired: 9 out]
            n885 = call "CAN参数设置.vi"() -> ("取消"=w2449:bool, "工作方式 2"=w2450:u8, "CAN卡类型 2"=w2456:u32, "设备索引号 2"=w2455:u16, "波特率 2"=w2454:T12, "CAN端口 2"=w2453:u16, "E-U_baud 2"=w2452:u32, "滤波方式 2"=w2451:u8)  [unwired: 11 in, 1 out]
            n886 = case shown="假" w2449 {
              tunnel: w2451 -> [w2463 _]
              tunnel: w2450 -> [w2462 _]
              tunnel: w2454 -> [w2461 _]
              tunnel: w2452 -> [w2460 _]
              tunnel: w2456 -> [w2459 _]
              tunnel: w2455 -> [w2458 _]
              tunnel: w2453 -> [w2457 _]
              frame False {
                n887 = local write "CAN端口"(w2457) -> ()
                n888 = local write "E-U_baud"(w2460) -> ()
                n889 = local write "CAN卡类型"(w2459) -> ()
                n890 = local write "滤波方式"(w2463) -> ()
                n891 = local write "工作方式"(w2462) -> ()
                n892 = local write "设备索引号"(w2458) -> ()
                n893 = local write "波特率"(w2461) -> ()
                n894 = global write "EV05全局变量1.vi" "设备索引号"(w2458) -> ()
                n895 = global write "EV05全局变量1.vi" "CAN卡类型"(w2459) -> ()
                n896 = global write "EV05全局变量1.vi" "波特率"(w2461) -> ()
                n897 = global write "EV05全局变量1.vi" "CAN端口"(w2457) -> ()
                n898 = global write "EV05全局变量1.vi" "E-U_baud"(w2460) -> ()
              }
              frame True {
              }
            }
          }
          event "System XY Graph": Shortcut Menu Selection (User) {
            n899 = event-data() -> ("ItemTag"=w2464:string)  [unwired: 8 out]
            n900 = case shown="\"查看单体详细信息\"" w2464 {
              frame "假", Default {
              }
              frame "查看单体详细信息" {
                n901 = stacked-sequence {
                  frame #0 {
                    w2465 = 2
                    n902 = property on="系统信息" class="Bool (严格)"("Disabled"=w2465) -> ()  [unwired: 2 in, 2 out]
                    n903 = property on="单箱信息" class="Bool (严格)"("Disabled"=w2465) -> ()  [unwired: 2 in, 2 out]
                    n904 = property on="诊断标定" class="Bool (严格)"("Disabled"=w2465) -> ()  [unwired: 2 in, 2 out]
                    n905 = property on="详细信息 4" class="Bool (严格)"("Disabled"=w2465) -> ()  [unwired: 2 in, 2 out]
                    n906 = property on="诊断标定 3" class="Bool (严格)"("Disabled"=w2465) -> ()  [unwired: 2 in, 2 out]
                    n907 = property on="单板信息 3" class="Bool (严格)"("Disabled"=w2465) -> ()  [unwired: 2 in, 2 out]
                  }
                  frame #1 {
                    n908 = local read "设备索引号"() -> (w2467:u16)
                    n909 = local read "CAN卡类型"() -> (w2468:u32)
                    n910 = local read "CAN端口"() -> (w2466:u16)
                    n911 = call "单体采集信息-new.vi"("can卡类型"=w2468, "设备索引号"=w2467, "CAN端口"=w2466) -> ()  [unwired: 3 in, 14 out]
                  }
                  frame #2 {
                    w2469 = 0
                    n912 = property on="系统信息" class="Bool (严格)"("Disabled"=w2469) -> ()  [unwired: 2 in, 2 out]
                    n913 = property on="单箱信息" class="Bool (严格)"("Disabled"=w2469) -> ()  [unwired: 2 in, 2 out]
                    n914 = property on="诊断标定" class="Bool (严格)"("Disabled"=w2469) -> ()  [unwired: 2 in, 2 out]
                    n915 = property on="详细信息 4" class="Bool (严格)"("Disabled"=w2469) -> ()  [unwired: 2 in, 2 out]
                    n916 = property on="诊断标定 3" class="Bool (严格)"("Disabled"=w2469) -> ()  [unwired: 2 in, 2 out]
                    n917 = property on="单板信息 3" class="Bool (严格)"("Disabled"=w2469) -> ()  [unwired: 2 in, 2 out]
                  }
                }
              }
            }
          }
          event "单箱信息", "单板信息 3": Value Change {
            n918 = event-data() -> ("NewVal"=w2470:bool)  [unwired: 6 out]
            n919 = case shown="真" w2470 {
              frame False {
              }
              frame True {
                n920 = stacked-sequence {
                  frame #0 {
                    n921 = disable-structure shown="禁用" {
                      frame Disabled {
                        w2472 = 2
                        n922 = property on="电压温度" class="Bool (严格)"("Disabled"=w2472) -> ()  [unwired: 2 in, 2 out]
                        n923 = property on="系统信息" class="Bool (严格)"("Disabled"=w2472) -> ()  [unwired: 2 in, 2 out]
                        n924 = property on="诊断标定" class="Bool (严格)"("Disabled"=w2472) -> ()  [unwired: 2 in, 2 out]
                        n925 = property on="详细信息 4" class="Bool (严格)"("Disabled"=w2472) -> ()  [unwired: 2 in, 2 out]
                        n926 = property on="详细信息 3" class="Bool (严格)"("Disabled"=w2472) -> ()  [unwired: 2 in, 2 out]
                        n927 = property on="诊断标定 3" class="Bool (严格)"("Disabled"=w2472) -> ()  [unwired: 2 in, 2 out]
                      }
                      frame Enabled {
                      }
                    }
                    n928 = property class="VI"("FP.State"=T10."Standard" ("前面板窗口:状态")) -> ()  [unwired: 2 in, 2 out]
                  }
                  frame #1 {
                    n929 = local read "状态"() -> (w2473:string)
                    n930 = call-by-ref "?"("状态 2"=w2473) -> ()  [unwired: 13 in, 2 out]
                  }
                  frame #2 {
                    n931 = disable-structure shown="禁用" {
                      frame Disabled {
                        w2475 = 0
                        n932 = property on="电压温度" class="Bool (严格)"("Disabled"=w2475) -> ()  [unwired: 2 in, 2 out]
                        n933 = property on="系统信息" class="Bool (严格)"("Disabled"=w2475) -> ()  [unwired: 2 in, 2 out]
                        n934 = property on="诊断标定" class="Bool (严格)"("Disabled"=w2475) -> ()  [unwired: 2 in, 2 out]
                        n935 = property on="详细信息 4" class="Bool (严格)"("Disabled"=w2475) -> ()  [unwired: 2 in, 2 out]
                        n936 = property on="详细信息 3" class="Bool (严格)"("Disabled"=w2475) -> ()  [unwired: 2 in, 2 out]
                        n937 = property on="诊断标定 3" class="Bool (严格)"("Disabled"=w2475) -> ()  [unwired: 2 in, 2 out]
                      }
                      frame Enabled {
                      }
                    }
                    n938 = property class="VI"("FP.State"=T10."Standard" ("前面板窗口:状态")) -> ()  [unwired: 2 in, 2 out]
                  }
                }
              }
            }
          }
          event "诊断标定", "诊断标定 3": Value Change {
            n939 = event-data() -> ("NewVal"=w2476:bool)  [unwired: 6 out]
            n940 = case shown="真" w2476 {
              frame False {
              }
              frame True {
                n941 = local read "参数配置"() -> (w2477:bool)
                n942 = case shown="真" w2477 {
                  frame False {
                  }
                  frame True {
                    n943 = stacked-sequence {
                      frame #0 {
                        n944 = property class="VI"("FP.State"=T10."Standard" ("前面板窗口:状态")) -> ()  [unwired: 2 in, 2 out]
                        n945 = local write "CAN初始化成功"(FALSE ("故障信息")) -> ()
                      }
                      frame #1 {
                        n946 = local read "设备索引号"() -> (w2481:u16)
                        n947 = local read "CAN卡类型"() -> (w2482:u32)
                        n948 = local read "CAN端口"() -> (w2480:u16)
                        n949 = call-by-ref "?"("CAN端口"=w2480, "设备索引号"=w2481, "CAN卡类型"=w2482) -> ()  [unwired: 11 in, 2 out]
                      }
                      frame #2 {
                        n950 = local write "CAN初始化成功"(TRUE ("CAN初始化成功")) -> ()
                        n951 = property class="VI"("FP.State"=T10."Standard" ("前面板窗口:状态")) -> ()  [unwired: 2 in, 2 out]
                      }
                    }
                  }
                }
              }
            }
          }
          event "退出", "退出 2": Value Change {
            n952 = event-data() -> ("NewVal"=w2485:bool)  [unwired: 6 out]
            n953 = stacked-sequence {
              tunnel: w2485 -> [_ w2493]
              frame #0 {
                n954 = local read "设备索引号"() -> (w2487:u16)
                n955 = local read "CAN卡类型"() -> (w2488:u32)
                n956 = local read "工作方式"() -> (w2490:u8)
                n957 = local read "滤波方式"() -> (w2489:u8)
                n958 = local read "CAN端口"() -> (w2486:u16)
                n959 = call-by-ref "?"("CAN卡类型"=w2488, "设备索引号"=w2487, "CAN端口"=w2486, "操作类型"=enum16{"初始化CAN", "关闭CAN"}."关闭CAN", "滤波方式"=w2489, "簇"=T14 {"打开CAN"=FALSE, "初始化CAN"=FALSE, "开始CAN"=FALSE, "重启"=FALSE, "关闭CAN"=TRUE}, "工作方式"=w2490) -> ()  [unwired: 12 in, 5 out]
              }
              frame #1 {
                n960 = Quit LabVIEW(quit? (T)=w2493) -> ()
                n961 = local write "退出 2"(w2493) -> ()
                n962 = local write "退出"(w2493) -> ()
              }
            }
          }
          event Panel Close {
            w2494 = TRUE
            n963 = event-data() -> ()  [unwired: 5 out]
            n964 = stacked-sequence {
              tunnel: w2494 -> [_ w2502]
              frame #0 {
                n965 = local read "设备索引号"() -> (w2496:u16)
                n966 = local read "CAN卡类型"() -> (w2497:u32)
                n967 = local read "工作方式"() -> (w2499:u8)
                n968 = local read "滤波方式"() -> (w2498:u8)
                n969 = local read "CAN端口"() -> (w2495:u16)
                n970 = call "CAN_Init-8.6.vi"("CAN卡类型"=w2497, "设备索引号"=w2496, "CAN端口"=w2495, "操作类型"=enum16{"初始化CAN", "关闭CAN"}."关闭CAN", "滤波方式"=w2498, "簇"=T14 {"打开CAN"=FALSE, "初始化CAN"=FALSE, "开始CAN"=FALSE, "重启"=FALSE, "关闭CAN"=TRUE}, "工作方式"=w2499) -> ()  [unwired: 7 in, 6 out]
              }
              frame #1 {
                n971 = local write "退出 2"(w2502) -> ()
                n972 = local write "退出"(w2502) -> ()
              }
            }
          }
        }
      }
      n973 = while {
        tunnel: w114 -> [w271]
        tunnel: w113 -> [w272]
        stop <- w260 stop-if-true
        n974 = Dequeue Element(queue=w271, timeout in ms (-1)=200 ("超时毫秒(-1)"), error in (no error)=w272) -> (element=w256:T2, error out=w259:errorcluster)  [unwired: 2 out]
        n975 = local read "退出"() -> (w260:bool)
        n976 = local read "中英文选择"() -> (w257:enum32{"中文", "English"})
        n977 = Unbundle(w256) -> ("ID"=w270:u32, "Data1"=w268:u8, "Data2"=w267:u8, "Data3"=w266:u8, "Data4"=w265:u8, "Data5"=w264:u8, "Data6"=w263:u8, "Data7"=w262:u8, "Data8"=w261:u8)  [unwired: 9 out]
        n978 = call <vilib>:"Clear Errors.vi"("error in (no error)"=w259) -> ()  [unwired: 6 in, 1 out]
        n979 = call "ID解析.vi"("ID"=w270) -> ("SA(4)"=w258:i32, "PF(2)"=w269:i32)  [unwired: 6 in, 3 out]
        n980 = case shown="FF" w269 {
          tunnel: w258 -> [_ _ _ _ _ w476 _ _ w614]
          tunnel: w268 -> [w273 w358 w375 w411 w475 w484 w580 _ w612]
          tunnel: w267 -> [w274 _ w374 w410 w474 w483 w579 _ w611]
          tunnel: w266 -> [w301 w359 w373 w409 w473 w482 w578 _ w610]
          tunnel: w265 -> [w286 w360 w372 w408 w472 w481 w582 _ w609]
          tunnel: w264 -> [w300 w361 w371 w407 w471 w480 w577 _ w613]
          tunnel: w263 -> [w304 w362 w370 w406 w470 w479 w576 _ _]
          tunnel: w262 -> [w303 w363 w369 w405 w469 w478 w575 _ w608]
          tunnel: w261 -> [w299 w364 w368 w404 w468 w477 w574 _ w616]
          tunnel: w257 -> [_ _ _ _ _ _ w581 _ w615]
          tunnel: w256 -> [w290 _ _ _ _ _ _ _ _]
          frame 7 {
            n981 = call "输出分辨率计算.vi"("数值1"=w300, "分辨率"=0.2, "数值 4"=w299, "数值 3"=w303, "数值 2"=w304) -> ("输出4"=w297:dbl, "输出3"=w305:dbl, "输出2"=w302:dbl, "输出1"=w298:dbl)  [unwired: 1 in, 2 out]
            "CC" <- w298
            "CC2" <- w297
            "AI1" <- w302
            "AI2" <- w305
            n982 = global write "电池信息全局变量.vi" "CC2"(w297) -> ()
            n983 = global write "电池信息全局变量.vi" "AI2"(w305) -> ()
            n984 = global write "电池信息全局变量.vi" "AI1"(w302) -> ()
            n985 = global write "电池信息全局变量.vi" "CC"(w298) -> ()
            n986 = global write "电池信息全局变量.vi" "CP"(w301) -> ()
            n987 = call "二进制解析-8.6.vi"("索引"=4, "数值"=w274) -> ("低位子数组"=w281:i32[], "高位子数组"=w313:i32[])  [unwired: 2 out]
            n988 = global write "电池信息全局变量.vi" "Rly"(w273) -> ()
            n989 = Delete From Array(array=w313, length=2 ("长度"), index=0 ("索引")) -> (deleted portion=w315:i32[], array with subset deleted=w314:i32[])
            n990 = Delete From Array(array=w281, length=2 ("长度"), index=0 ("索引")) -> (deleted portion=w284:i32[], array with subset deleted=w285:i32[])
            n991 = call "二进制解析-8.6.vi"("索引"=8, "数值"=w286) -> ("低位子数组"=w289:i32[])  [unwired: 3 out]
            n992 = call "二进制解析-8.6.vi"("索引"=8, "数值"=w273) -> ("低位子数组"=w319:i32[])  [unwired: 3 out]
            n993 = for {
              N: 4 -> [_]
              tunnel: w289 -> [w327]
              i -> [w323]
              w324 = 2 ("y")
              n994 = Multiply(x=w323, y=w324) -> (x*y=w325:i32)
              n995 = Array Subset(array=w327, index=w325, length=w324) -> (w326:i32[])
              n996 = call "数值二进制转十进制-8.6.vi"("子数组"=w326) -> ("十进制数值"=w322:i32)  [unwired: 4 out]
              n997 = case shown="1" w323 {
                tunnel: w322 -> [w330 w332 w335 w338]
                frame 0, Default {
                  n998 = Equal?(x=w330, y=0) -> (x = y?=w328:bool)
                  n999 = local write "DI1"(w328) -> ()
                }
                frame 1 {
                  n1000 = Equal?(x=w332, y=0) -> (x = y?=w331:bool)
                  n1001 = local write "DI2"(w331) -> ()
                }
                frame 2 {
                  n1002 = Equal?(x=w335, y=0) -> (x = y?=w334:bool)
                  n1003 = local write "DI3"(w334) -> ()
                }
                frame 3 {
                  n1004 = Equal?(x=w338, y=0) -> (x = y?=w337:bool)
                  n1005 = local write "DI4"(w337) -> ()
                }
              }
            }
            n1006 = for {
              N: 4 -> [_]
              tunnel: w319 -> [w345]
              i -> [w341]
              w342 = 2 ("y")
              n1007 = Multiply(x=w341, y=w342) -> (x*y=w343:i32)
              n1008 = Array Subset(array=w345, index=w343, length=w342) -> (w344:i32[])
              n1009 = call "数值二进制转十进制-8.6.vi"("子数组"=w344) -> ("十进制数值"=w340:i32)  [unwired: 4 out]
              n1010 = case shown="2" w341 {
                tunnel: w340 -> [w346 w349 w352 w355]
                frame 0, Default {
                  n1011 = Equal?(x=w346, y=1) -> (x = y?=w347:bool)
                  n1012 = local write "总正"(w347) -> ()
                  n1013 = global write "电池信息全局变量.vi" "总正"(w346) -> ()
                }
                frame 1 {
                  n1014 = Equal?(x=w349, y=1) -> (x = y?=w350:bool)
                  n1015 = local write "总负"(w350) -> ()
                  n1016 = global write "电池信息全局变量.vi" "总负"(w349) -> ()
                }
                frame 2 {
                  n1017 = global write "电池信息全局变量.vi" "预充"(w352) -> ()
                  n1018 = Equal?(x=w352, y=1) -> (x = y?=w353:bool)
                  n1019 = local write "预充"(w353) -> ()
                }
                frame 3 {
                  n1020 = Equal?(x=w355, y=1) -> (x = y?=w356:bool)
                  n1021 = global write "电池信息全局变量.vi" "充电"(w355) -> ()
                  n1022 = local write "充电"(w356) -> ()
                }
              }
            }
            n1023 = call "数值二进制转十进制-8.6.vi"("子数组"=w314) -> ("十进制数值"=w291:i32)  [unwired: 4 out]
            n1024 = call "数值二进制转十进制-8.6.vi"("子数组"=w315) -> ("十进制数值"=w292:i32)  [unwired: 4 out]
            n1025 = call "数值二进制转十进制-8.6.vi"("子数组"=w285) -> ("十进制数值"=w279:i32)  [unwired: 4 out]
            n1026 = call "数值二进制转十进制-8.6.vi"("子数组"=w284) -> ("十进制数值"=w277:i32)  [unwired: 4 out]
            n1027 = global write "电池信息全局变量.vi" "辅助继电器B"(w291) -> ()
            n1028 = global write "电池信息全局变量.vi" "辅助继电器A"(w292) -> ()
            n1029 = Equal?(x=w277, y=1) -> (x = y?=w276:bool)
            n1030 = Equal?(x=w279, y=1) -> (x = y?=w275:bool)
            n1031 = call "各种状态子VI.vi"("状态输入"=string[][] [["Off", "On", "Fault", "Rsv"], ["Off", "On", "Fault", "Rsv"], ["DO_LOW", "DO_High", "Rsv", "Rsv"], ["DO_LOW", "DO_High", "Rsv", "Rsv"]], "几种类型"=4, "数值"=w274) -> ("状态"=w307:string[])  [unwired: 1 in, 1 out]
            n1032 = call "各种状态子VI.vi"("状态输入"=string[][] [["DI_LOW", "DI_High", "Rsv", "Rsv"], ["DI_LOW", "DI_High", "Rsv", "Rsv"], ["DI_LOW", "DI_High", "Rsv", "Rsv"], ["DI_LOW", "DI_High", "Rsv", "Rsv"]], "几种类型"=4, "数值"=w286) -> ("状态"=w306:string[])  [unwired: 1 in, 1 out]
            n1033 = local write "DO2"(w275) -> ()
            n1034 = local write "DO1"(w276) -> ()
            n1035 = global write "电池信息全局变量.vi" "DI"(w306) -> ()
            n1036 = global write "电池信息全局变量.vi" "DO"(w307) -> ()
            n1037 = Equal?(x=w292, y=1) -> (x = y?=w294:bool)
            n1038 = Equal?(x=w291, y=1) -> (x = y?=w293:bool)
            n1039 = local write "加热"(w293) -> ()
            n1040 = local write "风机"(w294) -> ()
            n1041 = global write "电池信息全局变量.vi" "DO_D"(w274) -> ()
            n1042 = global write "电池信息全局变量.vi" "DI_D"(w286) -> ()
            "VCI_Receive 2" <- w290
            "CP" <- w301
          }
          frame 8 {
            n1043 = global write "电池信息全局变量.vi" "07"(w358) -> ()
            n1044 = call "时间合并-8.6.vi"("年"=w359, "月"=w360, "日"=w361, "时"=w362, "分"=w363, "秒"=w364) -> ("时间"=w365:string)  [unwired: 13 out]
            n1045 = local write "BMS时间"(w365) -> ()
            n1046 = global write "EV05全局变量1.vi" "BMS时间"(w365) -> ()
          }
          frame 10 {
            n1047 = Compound Arithmetic op=ADD(w375, w374, w373, w372, w371, w370, w369, w368) -> (w366:u8)
            n1048 = call "故障数值解析.vi"("输入"=w369) -> ("结果"=w380:string[])  [unwired: 2 out]
            n1049 = call "故障数值解析.vi"("输入"=w368) -> ("结果"=w378:string[])  [unwired: 2 out]
            n1050 = call "故障数值解析.vi"("输入"=w375) -> ("结果"=w385:string[])  [unwired: 2 out]
            n1051 = call "故障数值解析.vi"("输入"=w374) -> ("结果"=w384:string[])  [unwired: 2 out]
            n1052 = call "故障数值解析.vi"("输入"=w373) -> ("结果"=w383:string[])  [unwired: 2 out]
            n1053 = call "故障数值解析.vi"("输入"=w372) -> ("结果"=w379:string[])  [unwired: 2 out]
            n1054 = call "故障数值解析.vi"("输入"=w371) -> ("结果"=w382:string[])  [unwired: 2 out]
            n1055 = call "故障数值解析.vi"("输入"=w370) -> ("结果"=w381:string[])  [unwired: 2 out]
            n1056 = local write "电池故障 5"(w366) -> ()
            n1057 = Number To Hexadecimal String(1:i16 2 ("宽度(-)"), 2:w375) -> (0:w394:string)
            n1058 = Number To Hexadecimal String(1:i16 2 ("宽度(-)"), 2:w374) -> (0:w393:string)
            n1059 = Number To Hexadecimal String(1:i16 2 ("宽度(-)"), 2:w373) -> (0:w392:string)
            n1060 = Number To Hexadecimal String(1:i16 2 ("宽度(-)"), 2:w372) -> (0:w391:string)
            n1061 = Number To Hexadecimal String(1:i16 2 ("宽度(-)"), 2:w371) -> (0:w390:string)
            n1062 = Number To Hexadecimal String(1:i16 2 ("宽度(-)"), 2:w370) -> (0:w389:string)
            n1063 = Number To Hexadecimal String(1:i16 2 ("宽度(-)"), 2:w369) -> (0:w388:string)
            n1064 = Number To Hexadecimal String(1:i16 2 ("宽度(-)"), 2:w368) -> (0:w387:string)
            n1065 = Build Array(w385, w384, w383, w379, w382, w381, w380, w378) -> (w376:string[][])
            n1066 = Concatenate Strings(w394, w393, w392, w391, w390, w389, w388, w387) -> (w386:string)
            "电池故障 19" <- w386
            n1067 = Reshape Array(w376, 32 ("维数大小")) -> (w367:string[])
            n1068 = global write "EV05全局变量1.vi" "电池故障"(w386) -> ()
            n1069 = global write "电池信息全局变量.vi" "电池故障"(w367) -> ()
          }
          frame 11 {
            n1070 = Compound Arithmetic op=ADD(w411, w410, w409, w408, w407, w406, w405, w404) -> (w403:u8)
            n1071 = local write "电池故障2 4"(w403) -> ()
            n1072 = call "故障数值解析.vi"("输入"=w411) -> ("结果"=w422:string[])  [unwired: 2 out]
            n1073 = call "故障数值解析.vi"("输入"=w410) -> ("结果"=w421:string[])  [unwired: 2 out]
            n1074 = call "故障数值解析.vi"("输入"=w409) -> ("结果"=w420:string[])  [unwired: 2 out]
            n1075 = call "故障数值解析.vi"("输入"=w408) -> ("结果"=w416:string[])  [unwired: 2 out]
            n1076 = call "故障数值解析.vi"("输入"=w407) -> ("结果"=w419:string[])  [unwired: 2 out]
            n1077 = call "故障数值解析.vi"("输入"=w406) -> ("结果"=w418:string[])  [unwired: 2 out]
            n1078 = call "故障数值解析.vi"("输入"=w405) -> ("结果"=w417:string[])  [unwired: 2 out]
            n1079 = call "故障数值解析.vi"("输入"=w404) -> ("结果"=w415:string[])  [unwired: 2 out]
            n1080 = Number To Hexadecimal String(1:i16 2 ("宽度(-)"), 2:w411) -> (0:w431:string)
            n1081 = Number To Hexadecimal String(1:i16 2 ("宽度(-)"), 2:w410) -> (0:w430:string)
            n1082 = Number To Hexadecimal String(1:i16 2 ("宽度(-)"), 2:w409) -> (0:w429:string)
            n1083 = Number To Hexadecimal String(1:i16 2 ("宽度(-)"), 2:w408) -> (0:w428:string)
            n1084 = Number To Hexadecimal String(1:i16 2 ("宽度(-)"), 2:w407) -> (0:w427:string)
            n1085 = Number To Hexadecimal String(1:i16 2 ("宽度(-)"), 2:w406) -> (0:w426:string)
            n1086 = Number To Hexadecimal String(1:i16 2 ("宽度(-)"), 2:w405) -> (0:w425:string)
            n1087 = Number To Hexadecimal String(1:i16 2 ("宽度(-)"), 2:w404) -> (0:w424:string)
            n1088 = Concatenate Strings(w431, w430, w429, w428, w427, w426, w425, w424) -> (w423:string)
            "电池故障 20" <- w423
            n1089 = Build Array(w422, w421, w420, w416, w419, w418, w417, w415) -> (w413:string[][])
            n1090 = global write "EV05全局变量1.vi" "电池系统故障"(w423) -> ()
            n1091 = Reshape Array(w413, 32 ("维数大小")) -> (w412:string[])
            n1092 = global write "电池信息全局变量.vi" "电池系统故障"(w412) -> ()
          }
          frame 12 {
            n1093 = Compound Arithmetic op=ADD(w475, w474, w473, w472, w471, w470, w469, w468) -> (w440:u8)
            n1094 = local write "电池故障3 4"(w440) -> ()
            n1095 = call "故障数值解析.vi"("输入"=w475) -> ("结果"=w451:string[])  [unwired: 2 out]
            n1096 = call "故障数值解析.vi"("输入"=w474) -> ("结果"=w450:string[])  [unwired: 2 out]
            n1097 = call "故障数值解析.vi"("输入"=w473) -> ("结果"=w449:string[])  [unwired: 2 out]
            n1098 = call "故障数值解析.vi"("输入"=w472) -> ("结果"=w445:string[])  [unwired: 2 out]
            n1099 = call "故障数值解析.vi"("输入"=w471) -> ("结果"=w448:string[])  [unwired: 2 out]
            n1100 = call "故障数值解析.vi"("输入"=w470) -> ("结果"=w447:string[])  [unwired: 2 out]
            n1101 = call "故障数值解析.vi"("输入"=w469) -> ("结果"=w446:string[])  [unwired: 2 out]
            n1102 = call "故障数值解析.vi"("输入"=w468) -> ("结果"=w444:string[])  [unwired: 2 out]
            n1103 = Number To Hexadecimal String(1:i16 2 ("宽度(-)"), 2:w475) -> (0:w460:string)
            n1104 = Number To Hexadecimal String(1:i16 2 ("宽度(-)"), 2:w474) -> (0:w459:string)
            n1105 = Number To Hexadecimal String(1:i16 2 ("宽度(-)"), 2:w473) -> (0:w458:string)
            n1106 = Number To Hexadecimal String(1:i16 2 ("宽度(-)"), 2:w472) -> (0:w457:string)
            n1107 = Number To Hexadecimal String(1:i16 2 ("宽度(-)"), 2:w471) -> (0:w456:string)
            n1108 = Number To Hexadecimal String(1:i16 2 ("宽度(-)"), 2:w470) -> (0:w455:string)
            n1109 = Number To Hexadecimal String(1:i16 2 ("宽度(-)"), 2:w469) -> (0:w454:string)
            n1110 = Number To Hexadecimal String(2:w468) -> (0:w453:string)  [unwired: 1 out]
            n1111 = Build Array(w451, w450, w449, w445, w448, w447, w446, w444) -> (w442:string[][])
            n1112 = Concatenate Strings(w460, w459, w458, w457, w456, w455, w454, w453) -> (w452:string)
            "电池故障 21" <- w452
            n1113 = global write "EV05全局变量1.vi" "其他故障"(w452) -> ()
            n1114 = Reshape Array(w442, 32 ("维数大小")) -> (w441:string[])
            n1115 = global write "电池信息全局变量.vi" "其他故障"(w441) -> ()
          }
          frame 13 {
            n1116 = case shown="0" w476 {
              selector: w476 -> [_ w525]
              tunnel: w484 -> [w494 w534]
              tunnel: w483 -> [w493 w533]
              tunnel: w482 -> [w492 w532]
              tunnel: w481 -> [w491 w531]
              tunnel: w480 -> [w490 w530]
              tunnel: w479 -> [w489 w529]
              tunnel: w478 -> [w488 w528]
              tunnel: w477 -> [w487 w527]
              frame 0 {
                n1117 = Compound Arithmetic op=ADD(w494, w493, w492, w491, w490, w489, w488, w487) -> (w485:u8)
                n1118 = local write "电池故障4 4"(w485) -> ()
                n1119 = call "故障数值解析.vi"("输入"=w494) -> ("结果"=w504:string[])  [unwired: 2 out]
                n1120 = call "故障数值解析.vi"("输入"=w493) -> ("结果"=w503:string[])  [unwired: 2 out]
                n1121 = call "故障数值解析.vi"("输入"=w492) -> ("结果"=w502:string[])  [unwired: 2 out]
                n1122 = call "故障数值解析.vi"("输入"=w491) -> ("结果"=w498:string[])  [unwired: 2 out]
                n1123 = call "故障数值解析.vi"("输入"=w490) -> ("结果"=w501:string[])  [unwired: 2 out]
                n1124 = call "故障数值解析.vi"("输入"=w489) -> ("结果"=w500:string[])  [unwired: 2 out]
                n1125 = call "故障数值解析.vi"("输入"=w488) -> ("结果"=w499:string[])  [unwired: 2 out]
                n1126 = call "故障数值解析.vi"("输入"=w487) -> ("结果"=w497:string[])  [unwired: 2 out]
                n1127 = Number To Hexadecimal String(1:i16 2 ("宽度(-)"), 2:w494) -> (0:w513:string)
                n1128 = Number To Hexadecimal String(1:i16 2 ("宽度(-)"), 2:w493) -> (0:w512:string)
                n1129 = Number To Hexadecimal String(1:i16 2 ("宽度(-)"), 2:w492) -> (0:w511:string)
                n1130 = Number To Hexadecimal String(1:i16 2 ("宽度(-)"), 2:w491) -> (0:w510:string)
                n1131 = Number To Hexadecimal String(1:i16 2 ("宽度(-)"), 2:w490) -> (0:w509:string)
                n1132 = Number To Hexadecimal String(1:i16 2 ("宽度(-)"), 2:w489) -> (0:w508:string)
                n1133 = Number To Hexadecimal String(1:i16 2 ("宽度(-)"), 2:w488) -> (0:w507:string)
                n1134 = Number To Hexadecimal String(1:i16 2 ("宽度(-)"), 2:w487) -> (0:w506:string)
                n1135 = Concatenate Strings(w513, w512, w511, w510, w509, w508, w507, w506) -> (w505:string)
                "电池故障 22" <- w505
                n1136 = Build Array(w504, w503, w502, w498, w501, w500, w499, w497) -> (w495:string[][])
                n1137 = global write "EV05全局变量1.vi" "硬件故障"(w505) -> ()
                n1138 = Reshape Array(w495, 32 ("维数大小")) -> (w486:string[])
                n1139 = global write "电池信息全局变量.vi" "硬件故障"(w486) -> ()
              }
              frame 1, Default {
                n1140 = Decrement(x=w525) -> (x-1=w522:i32)
                n1141 = Number To Hexadecimal String(1:i16 2 ("宽度(-)"), 2:w534) -> (0:w542:string)
                n1142 = Number To Hexadecimal String(1:i16 2 ("宽度(-)"), 2:w533) -> (0:w541:string)
                n1143 = Number To Hexadecimal String(1:i16 2 ("宽度(-)"), 2:w532) -> (0:w540:string)
                n1144 = Number To Hexadecimal String(1:i16 2 ("宽度(-)"), 2:w531) -> (0:w539:string)
                n1145 = Number To Hexadecimal String(1:i16 2 ("宽度(-)"), 2:w530) -> (0:w538:string)
                n1146 = Number To Hexadecimal String(1:i16 2 ("宽度(-)"), 2:w529) -> (0:w537:string)
                n1147 = Number To Hexadecimal String(1:i16 2 ("宽度(-)"), 2:w528) -> (0:w536:string)
                n1148 = Number To Hexadecimal String(1:i16 2 ("宽度(-)"), 2:w527) -> (0:w535:string)
                n1149 = global read "从板全局变量.vi" "故障信息"() -> (w526:string[])
                n1150 = Concatenate Strings(w542, w541, w540, w539, w538, w537, w536, w535) -> (w524:string)
                n1151 = Replace Array Subset(array=w526, new element=w524, index=w522) -> (w523:string[])
                n1152 = global write "从板全局变量.vi" "故障信息"(w523) -> ()
              }
            }
          }
          frame 15 {
            n1153 = Join Numbers(hi=w577, lo=w576) -> ((hi.lo)=w554:u16)
            n1154 = Join Numbers(hi=w575, lo=w574) -> ((hi.lo)=w553:u16)
            n1155 = call "二进制解析-8.6.vi"("索引"=6, "数值"=w582) -> ("高位子数组"=w572:i32[])  [unwired: 3 out]
            n1156 = Format Into String(format string="%#f" ("格式字符串"), w554) -> (resulting string=w566:string)  [unwired: 2 in, 1 out]
            n1157 = Format Into String(format string="%#f" ("格式字符串"), w553) -> (resulting string=w567:string)  [unwired: 2 in, 1 out]
            n1158 = call "数值二进制转十进制-8.6.vi"("子数组"=w572) -> ("十进制数值"=w571:i32)  [unwired: 4 out]
            n1159 = Build Array(w580, w579, w578, w554, w553) -> (w568:u16[])
            n1160 = case shown="\"中文\", 默认" w581 {
              tunnel: w571 -> [w586 w598]
              tunnel: [w585 w596] -> w569
              tunnel: [w584 w597] -> w570
              tunnel: [w583 w596] -> w551
              frame "中文", Default {
                n1161 = case shown="3" w586 {
                  tunnel: ["正常" "异常" "无效"] -> w585
                  tunnel: [u32 87470 u32 10241033 u32 10241033] -> w584
                  tunnel: ["Normal" "Abnormal" "Invalid"] -> w583
                  frame 0, Default {
                  }
                  frame 1 {
                  }
                  frame 3 {
                  }
                }
              }
              frame "English" {
                n1162 = case shown="0, 默认" w598 {
                  tunnel: ["Normal" "Abnormal" "Invalid"] -> w596
                  tunnel: [u32 87470 u32 10241033 u32 10241033] -> w597
                  frame 0, Default {
                  }
                  frame 1 {
                  }
                  frame 3 {
                  }
                }
              }
            }
            n1163 = global write "电池信息全局变量.vi" "电池信息解析"(w568) -> ()
            n1164 = global write "EV05全局变量1.vi" "电池系统绝缘状态"(w551) -> ()
            n1165 = local write "电池系统绝缘状态"(w569) -> ()
            n1166 = property on="电池系统绝缘状态" class="Str"("Text.TextColor"=w570) -> ()  [unwired: 2 in, 2 out]
            n1167 = call "各种状态子VI.vi"("状态输入"=string[][] [["Rsv", "Rsv", "Rsv"], ["Normal", "Achieve Conditions", "Don't trust status"], ["Normal", "Manual Stop", "Don't trust status"], ["Normal", "Fault Stop", "Don't trust status"]], "几种类型"=4, "数值"=w578) -> ("状态"=w563:string[])  [unwired: 1 in, 1 out]
            n1168 = call "各种状态子VI.vi"("状态输入"=string[][] [["Normal", "Abnormal", "Invalid"], ["Normal", "Abnormal", "Invalid"], ["Normal", "Abnormal", "Invalid"], ["Normal", "Abnormal", "Invalid"]], "几种类型"=4, "数值"=w579) -> ("状态"=w562:string[])  [unwired: 1 in, 1 out]
            n1169 = call "各种状态子VI.vi"("状态输入"=string[][] [["Normal", "Abnormal", "Invalid", "Rsv"], ["Close", "Open", "Fault", "Invalid"], ["Close", "Open", "Fault", "Invalid"], ["Close", "Open", "Fault", "Invalid"]], "几种类型"=4, "数值"=w580) -> ("状态"=w561:string[])  [unwired: 1 in, 1 out]
            n1170 = Build Array (concatenate)(w561, w562, w563, w566, w567) -> (w552:string[])
            n1171 = global write "电池信息全局变量.vi" "电池信息解析2"(w552) -> ()
          }
          frame 153, Default {
          }
          frame 255 {
            n1172 = case shown="0" w614 {
              selector: w614 -> [_ w648]
              tunnel: w616 -> [w623 w641]
              tunnel: w615 -> [w639 w668]
              tunnel: w613 -> [w637 w667]
              tunnel: w612 -> [w635 w665]
              tunnel: w611 -> [w634 w664]
              tunnel: w610 -> [w633 w663]
              tunnel: w609 -> [w632 w662]
              tunnel: w608 -> [w620 _]
              frame 0 {
                n1173 = global write "电池信息全局变量.vi" "从板个数"(w620) -> ()
                n1174 = Build Array(w635, w634, w633, w632) -> (w629:u8[])
                n1175 = call "运行模式解析.vi"("中英文选择"=w639, "输入值"=w637) -> ("输出值"=w638:string)
                n1176 = local write "系统运行模式"(w638) -> ()
                n1177 = call "电池组信息解析.vi"("电池组信息?"=FALSE, "Protocol_Version"=w629) -> ("协议版本号"=w628:T17)  [unwired: 3 in, 6 out]
                n1178 = Number To Decimal String(number=w623) -> (decimal integer string=→"Life":string)  [unwired: 1 out]
                n1179 = global write "EV05全局变量1.vi" "life"(w623) -> ()
                n1180 = Unbundle(w628) -> ("版本号"=w626:string, "应用类型"=w627:string, "波特率"=w625:string, "协议是否公开"=w624:string)
                n1181 = global write "EV05全局变量1.vi" "应用类型"(w627) -> ()
                n1182 = global write "EV05全局变量1.vi" "协议版本号"(w626) -> ()
                n1183 = global write "EV05全局变量1.vi" "波特率22"(w625) -> ()
                n1184 = global write "EV05全局变量1.vi" "协议是否公开"(w624) -> ()
                n1185 = local read "次要参数"() -> (w631:T5)
                n1186 = Bundle By Name(cluster=w631, "协议版本号"=w626, "应用类型"=w627, "波特率"=w625, "协议是否公开"=w624) -> (w630:T5)
                n1187 = local write "次要参数"(w630) -> ()
                n1188 = local write "Life超时"(1 ("Life超时")) -> ()
                "从板个数" <- w620
              }
              frame 1, Default {
                n1189 = Decrement(x=w648) -> (x-1=w640:i32)
                n1190 = Build Array(w665, w664, w663, w662) -> (w661:u8[])
                n1191 = call "运行模式解析.vi"("中英文选择"=w668, "输入值"=w667) -> ("输出值"=w657:string)
                n1192 = call "电池组信息解析.vi"("电池组信息?"=FALSE, "Protocol_Version"=w661) -> ("协议版本号"=w660:T17)  [unwired: 3 in, 6 out]
                n1193 = global read "从板全局变量.vi" "电池运行状态"() -> (w658:string[])
                n1194 = global read "从板全局变量.vi" "协议是否公开"() -> (w651:string[])
                n1195 = Unbundle(w660) -> ("版本号"=w655:string, "应用类型"=w654:string, "波特率"=w650:string, "协议是否公开"=w649:string)
                n1196 = global read "从板全局变量.vi" "应用类型"() -> (w653:string[])
                n1197 = global read "从板全局变量.vi" "版本号"() -> (w656:string[])
                n1198 = global read "从板全局变量.vi" "波特率"() -> (w652:string[])
                n1199 = global read "从板全局变量.vi" "Life"() -> (w659:dbl[])
                n1200 = Replace Array Subset(array=w659, new element=w641, index=w640) -> (w647:dbl[])
                n1201 = Replace Array Subset(array=w658, new element=w657, index=w640) -> (w646:string[])
                n1202 = Replace Array Subset(array=w656, new element=w655, index=w640) -> (w645:string[])
                n1203 = Replace Array Subset(array=w653, new element=w654, index=w640) -> (w644:string[])
                n1204 = Replace Array Subset(array=w652, new element=w650, index=w640) -> (w643:string[])
                n1205 = Replace Array Subset(array=w651, new element=w649, index=w640) -> (w642:string[])
                n1206 = global write "从板全局变量.vi" "版本号"(w645) -> ()
                n1207 = global write "从板全局变量.vi" "波特率"(w643) -> ()
                n1208 = global write "从板全局变量.vi" "应用类型"(w644) -> ()
                n1209 = global write "从板全局变量.vi" "电池运行状态"(w646) -> ()
                n1210 = global write "从板全局变量.vi" "协议是否公开"(w642) -> ()
                n1211 = global write "从板全局变量.vi" "Life"(w647) -> ()
              }
            }
            n1212 = case shown="1..1E" w614 {
              selector: w614 -> [w669 w670]
              tunnel: [w669 w670] -> w605
              frame 0, Default {
              }
              frame 1..30 {
              }
            }
            n1213 = local read "上电状态"() -> (w619:bool[])
            n1214 = Replace Array Subset(array=w619, new element=TRUE ("新元素/子数组"), index=w605) -> (w617:bool[])
            n1215 = local write "上电状态"(w617) -> ()
            n1216 = local read "数值"() -> (w606:i32)
            n1217 = Max & Min(x=w606, y=w605) -> (max(x,y)=w607:i32)  [unwired: 1 out]
            n1218 = local write "数值"(w607) -> ()
          }
        }
      }
      n1219 = while {
        tunnel: w121 -> [w685]
        tunnel: w120 -> [w686]
        stop <- w674 stop-if-true
        n1220 = local read "中英文选择"() -> (w689:enum32{"中文", "English"})
        n1221 = Dequeue Element(queue=w685, timeout in ms (-1)=200 ("超时毫秒(-1)"), error in (no error)=w686) -> (element=w684:T2, error out=w673:errorcluster)  [unwired: 2 out]
        n1222 = local read "退出"() -> (w674:bool)
        n1223 = Unbundle(w684) -> ("ID"=w683:u32, "Data1"=w682:u8, "Data2"=w681:u8, "Data3"=w680:u8, "Data4"=w679:u8, "Data5"=w678:u8, "Data6"=w677:u8, "Data7"=w676:u8, "Data8"=w675:u8)  [unwired: 9 out]
        n1224 = call <vilib>:"Clear Errors.vi"("error in (no error)"=w673) -> ()  [unwired: 6 in, 1 out]
        n1225 = call "ID解析.vi"("ID"=w683) -> ("SA(4)"=w688:i32, "PS(3)"=w672:i32, "PF(2)"=w690:i32, "PDU(1)"=w687:i32)  [unwired: 6 in, 1 out]
        n1226 = case shown="8" w687 {
          tunnel: w690 -> [_ w699 _ _ _]
          tunnel: w689 -> [_ _ _ _ _]
          tunnel: w682 -> [_ w698 w1328 w1350 w1364]
          tunnel: w681 -> [_ w697 w1327 w1349 w1363]
          tunnel: w680 -> [_ w696 w1326 w1348 w1362]
          tunnel: w679 -> [_ w695 w1325 w1347 w1360]
          tunnel: w678 -> [_ w694 w1324 w1346 w1359]
          tunnel: w677 -> [_ w693 w1323 w1345 w1358]
          tunnel: w676 -> [_ w692 w1322 w1344 w1357]
          tunnel: w675 -> [_ w691 w1321 w1343 w1356]
          tunnel: w688 -> [_ w700 _ _ _]
          tunnel: w683 -> [_ _ w1329 w1351 w1361]
          tunnel: w672 -> [_ _ w1320 _ _]
          frame 0, Default {
          }
          frame 4 {
            n1227 = case shown="4" w699 {
              tunnel: w700 -> [w703 w777 w847 w951 _ w1040 _ w1101 w1146 w1203 w1248 _ _ _ _ _]
              tunnel: w698 -> [w709 w784 w855 w958 w1039 w1048 w1093 w1107 w1154 w1211 w1257 w1268 w1281 w1298 w1313 _]
              tunnel: w697 -> [w708 w783 w854 w957 w1038 w1047 _ w1106 w1153 w1210 w1255 w1267 w1280 w1297 w1312 _]
              tunnel: w696 -> [w705 w781 w853 w955 w1037 w1046 w1094 w1105 w1152 w1209 _ w1266 w1279 w1296 w1311 _]
              tunnel: w695 -> [w704 w782 w852 w956 w1036 w1045 w1095 w1104 w1151 w1208 _ w1265 w1278 w1295 w1310 _]
              tunnel: w694 -> [w707 w780 w851 w954 w1035 w1044 w1096 w1103 w1150 w1207 _ w1264 w1277 w1294 w1309 _]
              tunnel: w693 -> [w706 w779 w850 w953 w1034 w1043 w1097 w1102 w1149 w1206 w1250 w1263 w1276 w1293 w1308 _]
              tunnel: w692 -> [w702 w778 w849 w952 w1029 w1042 w1098 _ w1148 w1205 _ w1262 w1275 w1292 _ _]
              tunnel: w691 -> [w701 _ w848 w950 w1028 w1041 w1099 _ w1147 w1204 _ w1261 w1274 _ _ _]
              frame 1 {
                n1228 = case shown="1, 默认" w703 {
                  selector: w703 -> [_ w753]
                  tunnel: w709 -> [w739 w776]
                  tunnel: w708 -> [w738 w775]
                  tunnel: w707 -> [w734 w771]
                  tunnel: w706 -> [w733 w770]
                  tunnel: w705 -> [w732 w769]
                  tunnel: w704 -> [w731 w768]
                  tunnel: w702 -> [w727 w764]
                  tunnel: w701 -> [w726 w763]
                  frame 0 {
                    n1229 = Join Numbers(hi=w739, lo=w738) -> ((hi.lo)=w735:u16)
                    n1230 = Join Numbers(hi=w732, lo=w731) -> ((hi.lo)=w730:u16)
                    n1231 = Join Numbers(hi=w734, lo=w733) -> ((hi.lo)=w729:u16)
                    n1232 = Join Numbers(hi=w727, lo=w726) -> ((hi.lo)=w725:u16)
                    n1233 = local read "计数1"() -> (w723:i32)
                    n1234 = call "输出分辨率计算.vi"("分辨率"=0.1, "数值 3"=w729, "数值 2"=w735) -> ("输出3"=w724:dbl, "输出2"=w719:dbl)  [unwired: 3 in, 4 out]
                    "外总压" <- w724
                    n1235 = call "输出分辨率计算.vi"("偏移量"=sgl -3000.0, "分辨率"=0.1, "数值 3"=w725, "数值 2"=w730) -> ("输出3"=w713:dbl, "输出2"=w712:dbl)  [unwired: 2 in, 4 out]
                    "平均电流" <- w713
                    n1236 = local write "总电压(V)"(w719) -> ()
                    n1237 = local write "总电流(A)"(w712) -> ()
                    n1238 = Increment(x=w723) -> (x+1=w722:i32)
                    n1239 = Absolute Value(x=w712) -> (abs(x)=w711:dbl)
                    n1240 = global write "EV05全局变量1.vi" "总电压"(w719) -> ()
                    n1241 = global write "电池信息全局变量.vi" "外总压"(w724) -> ()
                    n1242 = local write "计数1"(w722) -> ()
                    n1243 = global write "电池信息全局变量.vi" "平均电流"(w713) -> ()
                    n1244 = global write "EV05全局变量1.vi" "总电流"(w712) -> ()
                    n1245 = In Range and Coerce(upper limit=40.0 ("上限"), x=w719, lower limit=5.0 ("下限")) -> (In Range?=w718:bool)  [unwired: 1 out]
                    n1246 = In Range and Coerce(upper limit=40.0 ("上限"), x=w711, lower limit=10.0 ("下限")) -> (In Range?=w716:bool)  [unwired: 1 out]
                    n1247 = case shown="假" w718 {
                      tunnel: w719 -> [w745 _]
                      tunnel: [w744 1.0] -> w717
                      frame False {
                        n1248 = Quotient & Remainder(x=w745, y=40.0) -> (floor(x/y)=w744:dbl)  [unwired: 1 out]
                      }
                      frame True {
                      }
                    }
                    n1249 = case shown="假" w716 {
                      tunnel: w711 -> [w741 _]
                      tunnel: [w740 1.0] -> w710
                      frame False {
                        n1250 = Quotient & Remainder(x=w741, y=40.0) -> (floor(x/y)=w740:dbl)  [unwired: 1 out]
                      }
                      frame True {
                      }
                    }
                    n1251 = local write "总电压进度"(w717) -> ()
                    n1252 = local write "总电流进度"(w710) -> ()
                  }
                  frame 1, Default {
                    n1253 = Join Numbers(hi=w776, lo=w775) -> ((hi.lo)=w772:u16)
                    n1254 = Join Numbers(hi=w769, lo=w768) -> ((hi.lo)=w767:u16)
                    n1255 = Join Numbers(hi=w771, lo=w770) -> ((hi.lo)=w766:u16)
                    n1256 = Join Numbers(hi=w764, lo=w763) -> ((hi.lo)=w762:u16)
                    n1257 = Decrement(x=w753) -> (x-1=w749:i32)
                    n1258 = call "输出分辨率计算.vi"("分辨率"=0.1, "数值 3"=w766, "数值 2"=w772) -> ("输出3"=w758:dbl, "输出2"=w748:dbl)  [unwired: 3 in, 4 out]
                    n1259 = call "输出分辨率计算.vi"("偏移量"=sgl -3000.0, "分辨率"=0.1, "数值 3"=w762, "数值 2"=w767) -> ("输出3"=w751:dbl, "输出2"=w755:dbl)  [unwired: 2 in, 4 out]
                    n1260 = global read "从板全局变量.vi" "总电压"() -> (w761:dbl[])
                    n1261 = global read "从板全局变量.vi" "总电流"() -> (w756:dbl[])
                    n1262 = global read "从板全局变量.vi" "平均电流"() -> (w752:dbl[])
                    n1263 = global read "从板全局变量.vi" "外总压"() -> (w759:dbl[])
                    n1264 = Replace Array Subset(array=w752, new element=w751, index=w749) -> (w750:dbl[])
                    n1265 = Replace Array Subset(array=w761, new element=w748, index=w749) -> (w760:dbl[])
                    n1266 = Replace Array Subset(array=w759, new element=w758, index=w749) -> (w757:dbl[])
                    n1267 = Replace Array Subset(array=w756, new element=w755, index=w749) -> (w754:dbl[])
                    n1268 = global write "从板全局变量.vi" "平均电流"(w750) -> ()
                    n1269 = global write "从板全局变量.vi" "总电压"(w760) -> ()
                    n1270 = global write "从板全局变量.vi" "外总压"(w757) -> ()
                    n1271 = global write "从板全局变量.vi" "总电流"(w754) -> ()
                  }
                }
              }
              frame 2 {
                n1272 = case shown="0" w777 {
                  selector: w777 -> [_ w818]
                  tunnel: w784 -> [w810 w846]
                  tunnel: w783 -> [w809 w845]
                  tunnel: w782 -> [w808 w844]
                  tunnel: w781 -> [w807 w843]
                  tunnel: w780 -> [w806 w842]
                  tunnel: w779 -> [w805 w841]
                  tunnel: w778 -> [w804 w840]
                  frame 0 {
                    n1273 = Join Numbers(hi=w810, lo=w809) -> ((hi.lo)=w794:u16)
                    n1274 = Join Numbers(hi=w807, lo=w808) -> ((hi.lo)=w793:u16)
                    n1275 = call "二进制解析-8.6.vi"("索引"=8, "数值"=w806) -> ("低位子数组"=w800:i32[])  [unwired: 3 out]
                    n1276 = call "二进制解析-8.6.vi"("索引"=4, "数值"=w805) -> ("低位子数组"=w797:i32[], "高位子数组"=w799:i32[])  [unwired: 2 out]
                    n1277 = call "二进制解析-8.6.vi"("索引"=8, "数值"=w804) -> ("低位子数组"=w796:i32[])  [unwired: 3 out]
                    n1278 = call "输出分辨率计算.vi"("分辨率"=0.001, "数值 3"=w793, "数值 2"=w794) -> ("输出3"=w785:dbl, "输出2"=w786:dbl)  [unwired: 3 in, 4 out]
                    n1279 = Insert Into Array(array=w800, new element=w799) -> (w798:i32[])  [unwired: 1 in]
                    n1280 = Insert Into Array(array=w797, new element=w796) -> (w795:i32[])  [unwired: 1 in]
                    n1281 = call "数值二进制转十进制-8.6.vi"("子数组"=w798) -> ("十进制数值"=w789:i32)  [unwired: 4 out]
                    n1282 = call "数值二进制转十进制-8.6.vi"("子数组"=w795) -> ("十进制数值"=w788:i32)  [unwired: 4 out]
                    n1283 = Subtract(x=w786, y=w785) -> (x-y=w787:dbl)
                    n1284 = local read "次要参数"() -> (w791:T5)
                    n1285 = Bundle By Name(cluster=w791, "压差"=w787, "最高单体电压"=w786, "最高电压位置"=w789, "最低单体电压"=w785, "最低电压位置"=w788) -> (w790:T5)
                    n1286 = global write "EV05全局变量1.vi" "单体最高电压"(w786) -> ()
                    n1287 = global write "EV05全局变量1.vi" "单体最低电压"(w785) -> ()
                    n1288 = global write "EV05全局变量1.vi" "位置1"(w789) -> ()
                    n1289 = global write "EV05全局变量1.vi" "位置2"(w788) -> ()
                    n1290 = global write "EV05全局变量1.vi" "压差"(w787) -> ()
                    n1291 = local write "次要参数"(w790) -> ()
                  }
                  frame 1, Default {
                    n1292 = Join Numbers(hi=w846, lo=w845) -> ((hi.lo)=w830:u16)
                    n1293 = Join Numbers(hi=w843, lo=w844) -> ((hi.lo)=w829:u16)
                    n1294 = call "二进制解析-8.6.vi"("索引"=8, "数值"=w842) -> ("低位子数组"=w836:i32[])  [unwired: 3 out]
                    n1295 = call "二进制解析-8.6.vi"("索引"=4, "数值"=w841) -> ("低位子数组"=w833:i32[], "高位子数组"=w835:i32[])  [unwired: 2 out]
                    n1296 = call "二进制解析-8.6.vi"("索引"=8, "数值"=w840) -> ("低位子数组"=w832:i32[])  [unwired: 3 out]
                    n1297 = call "输出分辨率计算.vi"("分辨率"=0.001, "数值 3"=w829, "数值 2"=w830) -> ("输出3"=w814:dbl, "输出2"=w816:dbl)  [unwired: 3 in, 4 out]
                    n1298 = Insert Into Array(array=w836, new element=w835) -> (w834:i32[])  [unwired: 1 in]
                    n1299 = Insert Into Array(array=w833, new element=w832) -> (w831:i32[])  [unwired: 1 in]
                    n1300 = Decrement(x=w818) -> (x-1=w811:i32)
                    n1301 = call "数值二进制转十进制-8.6.vi"("子数组"=w834) -> ("十进制数值"=w815:i32)  [unwired: 4 out]
                    n1302 = call "数值二进制转十进制-8.6.vi"("子数组"=w831) -> ("十进制数值"=w812:i32)  [unwired: 4 out]
                    n1303 = Subtract(x=w816, y=w814) -> (x-y=w813:dbl)
                    n1304 = global read "从板全局变量.vi" "最低电压位置"() -> (w821:dbl[])
                    n1305 = global read "从板全局变量.vi" "最高电压位置"() -> (w825:dbl[])
                    n1306 = global read "从板全局变量.vi" "最高电压"() -> (w827:dbl[])
                    n1307 = global read "从板全局变量.vi" "最低电压"() -> (w823:dbl[])
                    n1308 = global read "从板全局变量.vi" "压差"() -> (w819:dbl[])
                    n1309 = Replace Array Subset(array=w825, new element=w815, index=w811) -> (w824:dbl[])
                    n1310 = Replace Array Subset(array=w821, new element=w812, index=w811) -> (w820:dbl[])
                    n1311 = Replace Array Subset(array=w827, new element=w816, index=w811) -> (w826:dbl[])
                    n1312 = Replace Array Subset(array=w823, new element=w814, index=w811) -> (w822:dbl[])
                    n1313 = Replace Array Subset(array=w819, new element=w813, index=w811) -> (w817:dbl[])
                    n1314 = global write "从板全局变量.vi" "最低电压位置"(w820) -> ()
                    n1315 = global write "从板全局变量.vi" "最高电压"(w826) -> ()
                    n1316 = global write "从板全局变量.vi" "最低电压"(w822) -> ()
                    n1317 = global write "从板全局变量.vi" "最高电压位置"(w824) -> ()
                    n1318 = global write "从板全局变量.vi" "压差"(w817) -> ()
                  }
                }
              }
              frame 3 {
                n1319 = case shown="1, 默认" w847 {
                  selector: w847 -> [_ w918]
                  tunnel: w855 -> [w892 w941]
                  tunnel: w854 -> [w891 w940]
                  tunnel: w853 -> [w878 w936]
                  tunnel: w852 -> [w877 w935]
                  tunnel: w851 -> [w876 w934]
                  tunnel: w850 -> [w875 w914]
                  tunnel: w849 -> [w874 _]
                  tunnel: w848 -> [w873 _]
                  frame 0 {
                    n1320 = call "二进制解析-8.6.vi"("索引"=8, "数值"=w875) -> ("低位子数组"=w883:i32[])  [unwired: 3 out]
                    n1321 = call "二进制解析-8.6.vi"("索引"=4, "数值"=w874) -> ("低位子数组"=w886:i32[], "高位子数组"=w884:i32[])  [unwired: 2 out]
                    n1322 = call "二进制解析-8.6.vi"("索引"=8, "数值"=w873) -> ("低位子数组"=w887:i32[])  [unwired: 3 out]
                    n1323 = call "二进制解析-8.6.vi"("索引"=8, "数值"=w878) -> ("低位子数组"=w898:i32[])  [unwired: 3 out]
                    n1324 = call "二进制解析-8.6.vi"("索引"=4, "数值"=w877) -> ("低位子数组"=w895:i32[], "高位子数组"=w897:i32[])  [unwired: 2 out]
                    n1325 = call "二进制解析-8.6.vi"("索引"=8, "数值"=w876) -> ("低位子数组"=w894:i32[])  [unwired: 3 out]
                    n1326 = call "输出分辨率计算.vi"("偏移量"=sgl -40.0, "分辨率"=1.0, "数值 3"=w891, "数值 2"=w892) -> ("输出3"=w863:dbl, "输出2"=w864:dbl)  [unwired: 2 in, 4 out]
                    n1327 = Insert Into Array(array=w883, new element=w884) -> (w885:i32[])  [unwired: 1 in]
                    n1328 = Insert Into Array(array=w898, new element=w897) -> (w896:i32[])  [unwired: 1 in]
                    n1329 = Insert Into Array(array=w886, new element=w887) -> (w888:i32[])  [unwired: 1 in]
                    n1330 = Insert Into Array(array=w895, new element=w894) -> (w893:i32[])  [unwired: 1 in]
                    n1331 = global write "EV05全局变量1.vi" "单体最高温度"(w864) -> ()
                    n1332 = global write "EV05全局变量1.vi" "单体最低温度"(w863) -> ()
                    n1333 = Subtract(x=w864, y=w863) -> (x-y=w862:dbl)
                    n1334 = call "数值二进制转十进制-8.6.vi"("子数组"=w885) -> ("十进制数值"=w872:i32)  [unwired: 4 out]
                    n1335 = call "数值二进制转十进制-8.6.vi"("子数组"=w888) -> ("十进制数值"=w871:i32)  [unwired: 4 out]
                    n1336 = call "数值二进制转十进制-8.6.vi"("子数组"=w896) -> ("十进制数值"=w857:i32)  [unwired: 4 out]
                    n1337 = call "数值二进制转十进制-8.6.vi"("子数组"=w893) -> ("十进制数值"=w856:i32)  [unwired: 4 out]
                    n1338 = global write "EV05全局变量1.vi" "温差"(w862) -> ()
                    n1339 = call "输出分辨率计算.vi"("分辨率"=0.1, "数值 3"=w871, "数值 2"=w872) -> ("输出3"=w859:dbl, "输出2"=w860:dbl)  [unwired: 3 in, 4 out]
                    n1340 = case shown="1..10" w860 {
                      tunnel: [FALSE FALSE TRUE] -> w869
                      tunnel: [FALSE TRUE FALSE] -> w868
                      tunnel: [TRUE FALSE FALSE] -> w867
                      frame 1..10 {
                      }
                      frame 11..20 {
                      }
                      frame 21.., Default {
                      }
                    }
                    n1341 = global write "EV05全局变量1.vi" "位置3"(w857) -> ()
                    n1342 = global write "EV05全局变量1.vi" "位置4"(w856) -> ()
                    n1343 = local read "次要参数"() -> (w865:T5)
                    n1344 = Bundle By Name(cluster=w865, "温差"=w862, "最高单体温度"=w864, "最高温度位置"=w857, "最低单体温度"=w863, "最低温度位置"=w856) -> (w866:T5)
                    n1345 = local write "次要参数"(w866) -> ()
                    n1346 = property on="SOC" class="Slide (严格)"("Visible"=w869) -> ()  [unwired: 2 in, 2 out]
                    n1347 = property on="SOC(黄)" class="Slide (严格)"("Visible"=w868) -> ()  [unwired: 2 in, 2 out]
                    n1348 = property on="SOC(红)" class="Slide (严格)"("Visible"=w867) -> ()  [unwired: 2 in, 2 out]
                    n1349 = case shown="101.." w860 {
                      tunnel: [w903 100.0 ("输出2")] -> w861
                      tunnel: w860 -> [w903 _]
                      frame 0, Default {
                      }
                      frame 101.. {
                      }
                    }
                    n1350 = case shown="101.." w859 {
                      tunnel: [w901 100.0 ("输出2")] -> w858
                      tunnel: w859 -> [w901 _]
                      frame 0, Default {
                      }
                      frame 101.. {
                      }
                    }
                    n1351 = local write "SOH"(w858) -> ()
                    n1352 = global write "EV05全局变量1.vi" "SOH"(w858) -> ()
                    n1353 = local write "SOC"(w861) -> ()
                    n1354 = global write "EV05全局变量1.vi" "SOC"(w861) -> ()
                    n1355 = local write "SOC(黄)"(w861) -> ()
                    n1356 = local write "SOC(红)"(w861) -> ()
                  }
                  frame 1, Default {
                    n1357 = call "二进制解析-8.6.vi"("索引"=8, "数值"=w936) -> ("低位子数组"=w947:i32[])  [unwired: 3 out]
                    n1358 = call "二进制解析-8.6.vi"("索引"=4, "数值"=w935) -> ("低位子数组"=w944:i32[], "高位子数组"=w946:i32[])  [unwired: 2 out]
                    n1359 = call "二进制解析-8.6.vi"("索引"=8, "数值"=w934) -> ("低位子数组"=w943:i32[])  [unwired: 3 out]
                    n1360 = Decrement(x=w918) -> (x-1=w915:i32)
                    n1361 = call "输出分辨率计算.vi"("偏移量"=sgl -40.0, "分辨率"=1.0, "数值 3"=w940, "数值 2"=w941) -> ("输出3"=w926:dbl, "输出2"=w932:dbl)  [unwired: 2 in, 4 out]
                    n1362 = Insert Into Array(array=w947, new element=w946) -> (w945:i32[])  [unwired: 1 in]
                    n1363 = Insert Into Array(array=w944, new element=w943) -> (w942:i32[])  [unwired: 1 in]
                    n1364 = Subtract(x=w932, y=w926) -> (x-y=w920:dbl)
                    n1365 = call "数值二进制转十进制-8.6.vi"("子数组"=w945) -> ("十进制数值"=w929:i32)  [unwired: 4 out]
                    n1366 = call "数值二进制转十进制-8.6.vi"("子数组"=w942) -> ("十进制数值"=w923:i32)  [unwired: 4 out]
                    n1367 = global read "从板全局变量.vi" "温度个数"() -> (w916:u8[])
                    n1368 = global read "从板全局变量.vi" "最高温度"() -> (w933:dbl[])
                    n1369 = global read "从板全局变量.vi" "最高温度位置"() -> (w930:dbl[])
                    n1370 = global read "从板全局变量.vi" "最低温度"() -> (w927:dbl[])
                    n1371 = global read "从板全局变量.vi" "最低温度位置"() -> (w924:dbl[])
                    n1372 = global read "从板全局变量.vi" "温差"() -> (w921:dbl[])
                    n1373 = Replace Array Subset(array=w933, new element=w932, index=w915) -> (w931:dbl[])
                    n1374 = Array Subset(array=w921, index=w915, length=w920) -> (w919:dbl[])
                    n1375 = Replace Array Subset(array=w930, new element=w929, index=w915) -> (w928:dbl[])
                    n1376 = Replace Array Subset(array=w927, new element=w926, index=w915) -> (w925:dbl[])
                    n1377 = Replace Array Subset(array=w916, new element=w914, index=w915) -> (w917:u8[])
                    n1378 = Replace Array Subset(array=w924, new element=w923, index=w915) -> (w922:dbl[])
                    n1379 = global write "从板全局变量.vi" "温度个数"(w917) -> ()
                    n1380 = global write "从板全局变量.vi" "最高温度"(w931) -> ()
                    n1381 = global write "从板全局变量.vi" "最高温度位置"(w928) -> ()
                    n1382 = global write "从板全局变量.vi" "最低温度"(w925) -> ()
                    n1383 = global write "从板全局变量.vi" "温差"(w919) -> ()
                    n1384 = global write "从板全局变量.vi" "最低温度位置"(w922) -> ()
                  }
                }
              }
              frame 4 {
                n1385 = case shown="1, 默认" w951 {
                  selector: w951 -> [_ w1002]
                  tunnel: w958 -> [w973 w1011]
                  tunnel: w957 -> [w972 w1010]
                  tunnel: w956 -> [w970 w1008]
                  tunnel: w955 -> [w971 w1009]
                  tunnel: w954 -> [w969 w1007]
                  tunnel: w953 -> [w968 w1006]
                  tunnel: w952 -> [w967 w1005]
                  tunnel: w950 -> [_ w985]
                  frame 0 {
                    n1386 = Join Numbers(hi=w968, lo=w967) -> ((hi.lo)=w966:u16)
                    n1387 = call "二进制解析-8.6.vi"("索引"=8, "数值"=w971) -> ("低位子数组"=w980:i32[])  [unwired: 3 out]
                    n1388 = call "二进制解析-8.6.vi"("索引"=4, "数值"=w970) -> ("低位子数组"=w977:i32[], "高位子数组"=w979:i32[])  [unwired: 2 out]
                    n1389 = call "二进制解析-8.6.vi"("索引"=8, "数值"=w969) -> ("低位子数组"=w976:i32[])  [unwired: 3 out]
                    n1390 = call "输出分辨率计算.vi"("分辨率"=0.1, "数值 4"=w966, "数值 3"=w972, "数值 2"=w973) -> ("输出4"=w959:dbl, "输出3"=w961:dbl, "输出2"=w960:dbl)  [unwired: 2 in, 3 out]
                    n1391 = Insert Into Array(array=w980, new element=w979) -> (w978:i32[])  [unwired: 1 in]
                    n1392 = Insert Into Array(array=w977, new element=w976) -> (w975:i32[])  [unwired: 1 in]
                    n1393 = local read "次要参数"() -> (w965:T5)
                    n1394 = call "数值二进制转十进制-8.6.vi"("子数组"=w978) -> ("十进制数值"=w962:i32)  [unwired: 4 out]
                    n1395 = call "数值二进制转十进制-8.6.vi"("子数组"=w975) -> ("十进制数值"=w963:i32)  [unwired: 4 out]
                    n1396 = Bundle By Name(cluster=w965, "总内阻"=w959, "最高单体内阻"=w960, "最高内阻位置"=w962, "最低单体内阻"=w961, "最低内阻位置"=w963) -> (w964:T5)
                    n1397 = global write "EV05全局变量1.vi" "单体最低内阻"(w961) -> ()
                    n1398 = global write "EV05全局变量1.vi" "单体最高内阻"(w960) -> ()
                    n1399 = global write "EV05全局变量1.vi" "总内阻"(w959) -> ()
                    n1400 = global write "EV05全局变量1.vi" "位置5"(w962) -> ()
                    n1401 = global write "EV05全局变量1.vi" "位置6"(w963) -> ()
                    n1402 = local write "次要参数"(w964) -> ()
                  }
                  frame 1, Default {
                    n1403 = Decrement(x=w1002) -> (x-1=w986:i32)
                    n1404 = Join Numbers(hi=w1006, lo=w1005) -> ((hi.lo)=w1004:u16)
                    n1405 = call "二进制解析-8.6.vi"("索引"=8, "数值"=w1009) -> ("低位子数组"=w1018:i32[])  [unwired: 3 out]
                    n1406 = call "二进制解析-8.6.vi"("索引"=4, "数值"=w1008) -> ("低位子数组"=w1015:i32[], "高位子数组"=w1017:i32[])  [unwired: 2 out]
                    n1407 = call "二进制解析-8.6.vi"("索引"=8, "数值"=w1007) -> ("低位子数组"=w1014:i32[])  [unwired: 3 out]
                    n1408 = call "输出分辨率计算.vi"("分辨率"=0.1, "数值 4"=w1004, "数值 3"=w1010, "数值 2"=w1011) -> ("输出4"=w990:dbl, "输出3"=w988:dbl, "输出2"=w1001:dbl)  [unwired: 2 in, 3 out]
                    n1409 = Insert Into Array(array=w1018, new element=w1017) -> (w1016:i32[])  [unwired: 1 in]
                    n1410 = Insert Into Array(array=w1015, new element=w1014) -> (w1013:i32[])  [unwired: 1 in]
                    n1411 = call "数值二进制转十进制-8.6.vi"("子数组"=w1016) -> ("十进制数值"=w998:i32)  [unwired: 4 out]
                    n1412 = call "数值二进制转十进制-8.6.vi"("子数组"=w1013) -> ("十进制数值"=w989:i32)  [unwired: 4 out]
                    n1413 = global read "从板全局变量.vi" "最小内阻位置"() -> (w994:dbl[])
                    n1414 = global read "从板全局变量.vi" "最大内阻位置"() -> (w999:dbl[])
                    n1415 = global read "从板全局变量.vi" "最大内阻"() -> (w1003:dbl[])
                    n1416 = global read "从板全局变量.vi" "最小内阻"() -> (w997:dbl[])
                    n1417 = global read "从板全局变量.vi" "总内阻"() -> (w991:dbl[])
                    n1418 = global read "从板全局变量.vi" "电池节数"() -> (w987:u8[])
                    n1419 = Replace Array Subset(array=w991, new element=w990, index=w986) -> (w992:dbl[])
                    n1420 = Replace Array Subset(array=w997, new element=w988, index=w986) -> (w995:dbl[])
                    n1421 = Replace Array Subset(array=w999, new element=w998, index=w986) -> (w996:dbl[])
                    n1422 = Replace Array Subset(array=w994, new element=w989, index=w986) -> (w993:dbl[])
                    n1423 = Replace Array Subset(array=w1003, new element=w1001, index=w986) -> (w1000:dbl[])
                    n1424 = Replace Array Subset(array=w987, new element=w985, index=w986) -> (w984:u8[])
                    n1425 = global write "从板全局变量.vi" "最大内阻"(w1000) -> ()
                    n1426 = global write "从板全局变量.vi" "电池节数"(w984) -> ()
                    n1427 = global write "从板全局变量.vi" "最小内阻"(w995) -> ()
                    n1428 = global write "从板全局变量.vi" "最大内阻位置"(w996) -> ()
                    n1429 = global write "从板全局变量.vi" "总内阻"(w992) -> ()
                    n1430 = global write "从板全局变量.vi" "最小内阻位置"(w993) -> ()
                  }
                }
              }
              frame 5 {
                n1431 = Join Numbers(hi=w1029, lo=w1028) -> ((hi.lo)=w1027:u16)
                n1432 = Join Numbers(hi=w1035, lo=w1034) -> ((hi.lo)=w1026:u16)
                n1433 = Join Numbers(hi=w1026, lo=w1027) -> ((hi.lo)=w1025:u32)
                n1434 = call "输出分辨率计算.vi"("分辨率"=0.001, "数值 3"=w1025) -> ("输出3"=w1022:dbl)  [unwired: 4 in, 5 out]
                n1435 = Join Numbers(hi=w1039, lo=w1038) -> ((hi.lo)=w1033:u16)
                n1436 = Join Numbers(hi=w1037, lo=w1036) -> ((hi.lo)=w1032:u16)
                n1437 = global write "电池信息全局变量.vi" "实际容量"(w1022) -> ()
                n1438 = call "输出分辨率计算.vi"("分辨率"=0.1, "数值 3"=w1032, "数值 2"=w1033) -> ("输出3"=w1030:dbl, "输出2"=w1031:dbl)  [unwired: 3 in, 4 out]
                n1439 = global write "电池信息全局变量.vi" "最大充电电流"(w1031) -> ()
                n1440 = global write "电池信息全局变量.vi" "最大放电电流"(w1030) -> ()
              }
              frame 6 {
                n1441 = case shown="1, 默认" w1040 {
                  selector: w1040 -> [_ w1071]
                  tunnel: w1048 -> [w1058 w1083]
                  tunnel: w1047 -> [w1057 w1082]
                  tunnel: w1046 -> [w1056 w1081]
                  tunnel: w1045 -> [w1055 w1080]
                  tunnel: w1044 -> [w1054 w1079]
                  tunnel: w1043 -> [w1053 w1078]
                  tunnel: w1042 -> [w1052 w1077]
                  tunnel: w1041 -> [w1051 w1076]
                  frame 0 {
                    n1442 = Join Numbers(hi=w1054, lo=w1053) -> ((hi.lo)=w1063:u16)
                    n1443 = Join Numbers(hi=w1052, lo=w1051) -> ((hi.lo)=w1062:u16)
                    n1444 = Join Numbers(hi=w1058, lo=w1057) -> ((hi.lo)=w1065:u16)
                    n1445 = Join Numbers(hi=w1056, lo=w1055) -> ((hi.lo)=w1066:u16)
                    n1446 = Join Numbers(hi=w1063, lo=w1062) -> ((hi.lo)=w1061:u32)
                    n1447 = Join Numbers(hi=w1065, lo=w1066) -> ((hi.lo)=w1064:u32)
                    n1448 = To Double Precision Float(number=w1064) -> (double precision float=w1060:dbl)
                    n1449 = To Double Precision Float(number=w1061) -> (double precision float=w1059:dbl)
                    n1450 = call "输出分辨率计算.vi"("分辨率"=0.001, "数值 3"=w1059, "数值 2"=w1060) -> ("输出3"=w1049:dbl, "输出2"=w1050:dbl)  [unwired: 3 in, 4 out]
                    n1451 = global write "电池信息全局变量.vi" "充电总安时"(w1050) -> ()
                    n1452 = global write "电池信息全局变量.vi" "放电总安时"(w1049) -> ()
                  }
                  frame 1, Default {
                    n1453 = Join Numbers(hi=w1079, lo=w1078) -> ((hi.lo)=w1088:u16)
                    n1454 = Join Numbers(hi=w1077, lo=w1076) -> ((hi.lo)=w1087:u16)
                    n1455 = Join Numbers(hi=w1083, lo=w1082) -> ((hi.lo)=w1090:u16)
                    n1456 = Join Numbers(hi=w1081, lo=w1080) -> ((hi.lo)=w1091:u16)
                    n1457 = Join Numbers(hi=w1088, lo=w1087) -> ((hi.lo)=w1086:u32)
                    n1458 = Join Numbers(hi=w1090, lo=w1091) -> ((hi.lo)=w1089:u32)
                    n1459 = Decrement(x=w1071) -> (x-1=w1068:i32)
                    n1460 = To Double Precision Float(number=w1089) -> (double precision float=w1085:dbl)
                    n1461 = To Double Precision Float(number=w1086) -> (double precision float=w1084:dbl)
                    n1462 = global read "从板全局变量.vi" "充电总安时"() -> (w1074:dbl[])
                    n1463 = global read "从板全局变量.vi" "放电总安时"() -> (w1073:dbl[])
                    n1464 = call "输出分辨率计算.vi"("分辨率"=0.001, "数值 3"=w1084, "数值 2"=w1085) -> ("输出3"=w1069:dbl, "输出2"=w1070:dbl)  [unwired: 3 in, 4 out]
                    n1465 = Replace Array Subset(array=w1073, new element=w1069, index=w1068) -> (w1072:dbl[])
                    n1466 = Replace Array Subset(array=w1074, new element=w1070, index=w1068) -> (w1075:dbl[])
                    n1467 = global write "从板全局变量.vi" "放电总安时"(w1072) -> ()
                    n1468 = global write "从板全局变量.vi" "充电总安时"(w1075) -> ()
                  }
                }
              }
              frame 8 {
                n1469 = global write "电池信息全局变量.vi" "07"(w1093) -> ()
                n1470 = call "时间合并-8.6.vi"("年"=w1094, "月"=w1095, "日"=w1096, "时"=w1097, "分"=w1098, "秒"=w1099) -> ("时间"=w1100:string)  [unwired: 13 out]
                n1471 = local write "BMS时间"(w1100) -> ()
                n1472 = global write "EV05全局变量1.vi" "BMS时间"(w1100) -> ()
              }
              frame 9 {
                n1473 = case shown="1, 默认" w1101 {
                  selector: w1101 -> [_ w1128]
                  tunnel: w1107 -> [w1117 w1140]
                  tunnel: w1106 -> [w1116 w1139]
                  tunnel: w1105 -> [w1115 w1138]
                  tunnel: w1104 -> [w1114 w1137]
                  tunnel: w1103 -> [w1113 w1136]
                  tunnel: w1102 -> [w1112 w1135]
                  frame 0 {
                    n1474 = Join Numbers(hi=w1117, lo=w1116) -> ((hi.lo)=w1121:u16)
                    n1475 = Join Numbers(hi=w1115, lo=w1114) -> ((hi.lo)=w1120:u16)
                    n1476 = Join Numbers(hi=w1113, lo=w1112) -> ((hi.lo)=w1119:u16)
                    n1477 = call "输出分辨率计算.vi"("偏移量"=sgl -3000.0, "分辨率"=0.1, "数值 2"=w1119) -> ("输出2"=w1109:dbl)  [unwired: 3 in, 5 out]
                    n1478 = call "输出分辨率计算.vi"("分辨率"=0.5, "数值 3"=w1120, "数值 2"=w1121) -> ("输出3"=w1110:dbl, "输出2"=w1111:dbl)  [unwired: 3 in, 4 out]
                    n1479 = global write "电池信息全局变量.vi" "正绝缘"(w1111) -> ()
                    n1480 = global write "电池信息全局变量.vi" "负绝缘"(w1110) -> ()
                    n1481 = global write "电池信息全局变量.vi" "功率"(w1109) -> ()
                  }
                  frame 1, Default {
                    n1482 = Join Numbers(hi=w1140, lo=w1139) -> ((hi.lo)=w1144:u16)
                    n1483 = Join Numbers(hi=w1138, lo=w1137) -> ((hi.lo)=w1143:u16)
                    n1484 = Join Numbers(hi=w1136, lo=w1135) -> ((hi.lo)=w1142:u16)
                    n1485 = Decrement(x=w1128) -> (x-1=w1124:i32)
                    n1486 = call "输出分辨率计算.vi"("偏移量"=sgl -3000.0, "分辨率"=0.1, "数值 2"=w1142) -> ("输出2"=w1125:dbl)  [unwired: 3 in, 5 out]
                    n1487 = call "输出分辨率计算.vi"("分辨率"=0.5, "数值 3"=w1143, "数值 2"=w1144) -> ("输出3"=w1126:dbl, "输出2"=w1127:dbl)  [unwired: 3 in, 4 out]
                    n1488 = global read "从板全局变量.vi" "正绝缘"() -> (w1134:dbl[])
                    n1489 = global read "从板全局变量.vi" "负绝缘"() -> (w1133:dbl[])
                    n1490 = global read "从板全局变量.vi" "功率"() -> (w1131:dbl[])
                    n1491 = Replace Array Subset(array=w1134, new element=w1127, index=w1124) -> (w1132:dbl[])
                    n1492 = Replace Array Subset(array=w1133, new element=w1126, index=w1124) -> (w1129:dbl[])
                    n1493 = Replace Array Subset(array=w1131, new element=w1125, index=w1124) -> (w1130:dbl[])
                    n1494 = global write "从板全局变量.vi" "正绝缘"(w1132) -> ()
                    n1495 = global write "从板全局变量.vi" "负绝缘"(w1129) -> ()
                    n1496 = global write "从板全局变量.vi" "功率"(w1130) -> ()
                  }
                }
              }
              frame 16 {
                n1497 = case shown="1, 默认" w1146 {
                  selector: w1146 -> [_ w1172]
                  tunnel: w1154 -> [w1164 w1171]
                  tunnel: w1153 -> [w1163 w1178]
                  tunnel: w1152 -> [w1162 w1177]
                  tunnel: w1151 -> [w1156 w1170]
                  tunnel: w1150 -> [w1161 w1176]
                  tunnel: w1149 -> [w1160 w1175]
                  tunnel: w1148 -> [w1159 w1174]
                  tunnel: w1147 -> [w1158 w1173]
                  frame 0 {
                    n1498 = Join Numbers(hi=w1161, lo=w1160) -> ((hi.lo)=w1166:u16)
                    n1499 = Join Numbers(hi=w1159, lo=w1158) -> ((hi.lo)=w1169:u16)
                    n1500 = call "输出分辨率计算.vi"("分辨率"=0.1, "数值 2"=w1169) -> ("输出2"=w1155:dbl)  [unwired: 4 in, 5 out]
                    "BMS供电电压" <- w1155
                    n1501 = global write "电池信息全局变量.vi" "BMS_Volt"(w1155) -> ()
                    n1502 = call "输出分辨率计算.vi"("分辨率"=0.1, "数值 2"=w1166) -> ("输出2"=w1167:dbl)  [unwired: 4 in, 5 out]
                    n1503 = Build Array(w1164, w1163, w1162, w1156, w1167, w1155) -> (w1157:dbl[])
                    n1504 = global write "电池信息全局变量.vi" "F"(w1157) -> ()
                  }
                  frame 1, Default {
                    n1505 = disable-structure shown="禁用" {
                      disable-tunnel: w1178 -> [w1196 _]
                      disable-tunnel: w1177 -> [w1195 _]
                      disable-tunnel: w1176 -> [w1194 _]
                      disable-tunnel: w1175 -> [w1193 _]
                      disable-tunnel: w1174 -> [w1192 _]
                      disable-tunnel: w1173 -> [w1191 _]
                      disable-tunnel: w1172 -> [w1189 _]
                      disable-tunnel: w1171 -> [w1184 _]
                      disable-tunnel: w1170 -> [w1179 _]
                      frame Disabled {
                        n1506 = Join Numbers(hi=w1194, lo=w1193) -> ((hi.lo)=w1198:u16)
                        n1507 = Join Numbers(hi=w1192, lo=w1191) -> ((hi.lo)=w1201:u16)
                        n1508 = call "输出分辨率计算.vi"("分辨率"=0.1, "数值 2"=w1201) -> ("输出2"=w1202:dbl)  [unwired: 4 in, 5 out]
                        n1509 = Decrement(x=w1189) -> (x-1=w1181:i32)
                        n1510 = global read "从板全局变量.vi" "均衡标记"() -> (w1183:dbl[])
                        n1511 = call "二进制解析-8.6.vi"("索引"=6, "数值"=w1179) -> ("高位子数组"=w1186:i32[])  [unwired: 3 out]
                        n1512 = call "输出分辨率计算.vi"("分辨率"=0.1, "数值 2"=w1198) -> ("输出2"=w1199:dbl)  [unwired: 4 in, 5 out]
                        n1513 = call "数值二进制转十进制-8.6.vi"("子数组"=w1186) -> ("十进制数值"=w1182:i32)  [unwired: 4 out]
                        n1514 = Build Array(w1184, w1196, w1195, w1179, w1199, w1202) -> (w1187:dbl[])
                        n1515 = Replace Array Subset(array=w1183, new element=w1182, index=w1181) -> (w1180:dbl[])
                        n1516 = global read "从板全局变量.vi" "F"() -> (w1190:dbl[][])
                        n1517 = global write "从板全局变量.vi" "均衡标记"(w1180) -> ()
                        n1518 = Replace Array Subset(array=w1190, new element=w1187, index (row)=w1181) -> (w1188:dbl[][])  [unwired: 1 in]
                        n1519 = global write "从板全局变量.vi" "F"(w1188) -> ()
                      }
                      frame Enabled {
                      }
                    }
                  }
                }
              }
              frame 17 {
                n1520 = case shown="1" w1203 {
                  selector: w1203 -> [_ w1233]
                  tunnel: w1211 -> [w1224 w1232]
                  tunnel: w1210 -> [w1223 w1231]
                  tunnel: w1209 -> [w1222 w1230]
                  tunnel: w1208 -> [w1221 w1229]
                  tunnel: w1207 -> [w1220 w1228]
                  tunnel: w1206 -> [w1219 w1227]
                  tunnel: w1205 -> [w1218 w1226]
                  tunnel: w1204 -> [w1217 w1225]
                  frame 0, Default {
                    w1215 = "%#f" ("格式字符串")
                    n1521 = call "时间合并-8.6.vi"("年"=w1222, "月"=w1221, "日"=w1220, "时"=w1219, "分"=w1218, "秒"=w1217) -> ("时间"=w1216:string)  [unwired: 13 out]
                    n1522 = Format Into String(format string=w1215, w1224) -> (resulting string=w1214:string)  [unwired: 2 in, 1 out]
                    n1523 = Format Into String(format string=w1215, w1223) -> (resulting string=w1213:string)  [unwired: 2 in, 1 out]
                    n1524 = Build Array(w1214, w1213, w1216) -> (w1212:string[])
                    n1525 = global write "电池信息全局变量.vi" "10"(w1212) -> ()
                  }
                  frame 1 {
                    (unwired) 0.1 ("分辨率")
                    n1526 = Join Numbers(hi=w1228, lo=w1227) -> ((hi.lo)=w1244:u16)
                    n1527 = Join Numbers(hi=w1226, lo=w1225) -> ((hi.lo)=w1246:u16)
                    n1528 = call "输出分辨率计算.vi"("数值 2"=w1246) -> ("输出2"=w1247:dbl)  [unwired: 5 in, 5 out]
                    n1529 = Decrement(x=w1233) -> (x-1=w1235:i32)
                    n1530 = global read "从板全局变量.vi" "均衡标记"() -> (w1237:dbl[])
                    n1531 = call "二进制解析-8.6.vi"("索引"=6, "数值"=w1229) -> ("高位子数组"=w1239:i32[])  [unwired: 3 out]
                    n1532 = call "输出分辨率计算.vi"("分辨率"=0.1, "数值 2"=w1244) -> ("输出2"=w1245:dbl)  [unwired: 4 in, 5 out]
                    n1533 = call "数值二进制转十进制-8.6.vi"("子数组"=w1239) -> ("十进制数值"=w1236:i32)  [unwired: 4 out]
                    n1534 = Build Array(w1232, w1231, w1230, w1229, w1245, w1247) -> (w1240:dbl[])
                    n1535 = Replace Array Subset(array=w1237, new element=w1236, index=w1235) -> (w1234:dbl[])
                    n1536 = global read "从板全局变量.vi" "F"() -> (w1242:dbl[][])
                    n1537 = global write "从板全局变量.vi" "均衡标记"(w1234) -> ()
                    n1538 = Replace Array Subset(array=w1242, new element=w1240, index (row)=w1235) -> (w1241:dbl[][])  [unwired: 1 in]
                    n1539 = global write "从板全局变量.vi" "F"(w1241) -> ()
                  }
                }
              }
              frame 80 {
                n1540 = global read "从板全局变量.vi" "继电器2"() -> (w1256:dbl[])
                n1541 = global read "从板全局变量.vi" "满标志"() -> (w1252:dbl[])
                n1542 = global read "从板全局变量.vi" "继电器1"() -> (w1258:dbl[])
                n1543 = Decrement(x=w1248) -> (x-1=w1249:i32)
                n1544 = Replace Array Subset(array=w1252, new element=w1250, index=w1249) -> (w1251:dbl[])
                n1545 = Replace Array Subset(array=w1256, new element=w1255, index=w1249) -> (w1253:dbl[])
                n1546 = Replace Array Subset(array=w1258, new element=w1257, index=w1249) -> (w1254:dbl[])
                n1547 = global write "从板全局变量.vi" "满标志"(w1251) -> ()
                n1548 = global write "从板全局变量.vi" "继电器1"(w1254) -> ()
                n1549 = global write "从板全局变量.vi" "继电器2"(w1253) -> ()
              }
              frame 129 {
                n1550 = Build Array(w1268, w1267, w1266, w1265, w1264, w1263, w1262, w1261) -> (w1260:u8[])
                n1551 = global write "电池信息全局变量.vi" "列1"(w1260) -> ()
                n1552 = local write "充电超时1"(1 ("充电超时1")) -> ()
              }
              frame 130 {
                n1553 = Join Numbers(hi=w1277, lo=w1276) -> ((hi.lo)=w1285:u16)
                n1554 = Join Numbers(hi=w1275, lo=w1274) -> ((hi.lo)=w1282:u16)
                n1555 = Join Numbers(hi=w1279, lo=w1278) -> ((hi.lo)=w1271:u16)
                n1556 = Join Numbers(hi=w1281, lo=w1280) -> ((hi.lo)=w1270:u16)
                n1557 = global write "电池信息全局变量.vi" "累计充电时间"(w1270) -> ()
                n1558 = global write "电池信息全局变量.vi" "剩余充电时间"(w1271) -> ()
                n1559 = call "输出分辨率计算.vi"("分辨率"=0.1, "数值 2"=w1285) -> ("输出2"=w1273:dbl)  [unwired: 4 in, 5 out]
                n1560 = call "输出分辨率计算.vi"("分辨率"=0.001, "数值 2"=w1282) -> ("输出2"=w1272:dbl)  [unwired: 4 in, 5 out]
                n1561 = global write "电池信息全局变量.vi" "最高允许充电单体电压"(w1272) -> ()
                n1562 = global write "电池信息全局变量.vi" "最高允许充电总电压"(w1273) -> ()
                n1563 = local write "充电超时2"(1 ("充电超时1")) -> ()
              }
              frame 131 {
                n1564 = Join Numbers(hi=w1298, lo=w1297) -> ((hi.lo)=w1301:u16)
                n1565 = Join Numbers(hi=w1296, lo=w1295) -> ((hi.lo)=w1302:u16)
                n1566 = Join Numbers(hi=w1294, lo=w1293) -> ((hi.lo)=w1288:u16)
                n1567 = call "输出分辨率计算.vi"("偏移量"=sgl -40.0, "分辨率"=1.0, "数值 2"=w1292) -> ("输出2"=w1289:dbl)  [unwired: 3 in, 5 out]
                n1568 = call "输出分辨率计算.vi"("分辨率"=0.1, "数值 4"=w1288, "数值 3"=w1302, "数值 2"=w1301) -> ("输出4"=w1287:dbl, "输出3"=w1290:dbl, "输出2"=w1291:dbl)  [unwired: 2 in, 3 out]
                n1569 = global write "电池信息全局变量.vi" "最高允许充电温度"(w1289) -> ()
                n1570 = global write "电池信息全局变量.vi" "最小允许充电电流"(w1290) -> ()
                n1571 = global write "电池信息全局变量.vi" "充电电流步长"(w1287) -> ()
                n1572 = global write "电池信息全局变量.vi" "最大允许充电电流"(w1291) -> ()
                n1573 = local write "充电超时3"(1 ("充电超时1")) -> ()
              }
              frame 132 {
                n1574 = Join Numbers(hi=w1313, lo=w1312) -> ((hi.lo)=w1315:u16)
                n1575 = Join Numbers(hi=w1311, lo=w1310) -> ((hi.lo)=w1316:u16)
                n1576 = Join Numbers(hi=w1309, lo=w1308) -> ((hi.lo)=w1317:u16)
                n1577 = call "输出分辨率计算.vi"("分辨率"=0.1, "数值 4"=w1317, "数值 3"=w1316, "数值 2"=w1315) -> ("输出4"=w1307:dbl, "输出3"=w1306:dbl, "输出2"=w1305:dbl)  [unwired: 2 in, 3 out]
                n1578 = global write "电池信息全局变量.vi" "充电机累计输出能量"(w1307) -> ()
                n1579 = global write "电池信息全局变量.vi" "充电机输出电流"(w1306) -> ()
                n1580 = global write "电池信息全局变量.vi" "充电机输出电压"(w1305) -> ()
                n1581 = local write "充电超时4"(1 ("充电超时4")) -> ()
              }
              frame 153, Default {
              }
            }
          }
          frame 8 {
            n1582 = Equal?(x=145, y=w1320) -> (x = y?=w1318:bool)
            n1583 = case shown="真" w1318 {
              tunnel: w1329 -> [_ w1338]
              tunnel: w1328 -> [_ w1337]
              tunnel: w1327 -> [_ w1336]
              tunnel: w1326 -> [_ w1335]
              tunnel: w1325 -> [_ w1334]
              tunnel: w1324 -> [_ w1333]
              tunnel: w1323 -> [_ w1332]
              tunnel: w1322 -> [_ w1331]
              tunnel: w1321 -> [_ w1330]
              frame False {
              }
              frame True {
                n1584 = call-by-ref "?"("Data1"=w1337, "Data2"=w1336, "Data3"=w1335, "Data4"=w1334, "Data5"=w1333, "Data6"=w1332, "Data7"=w1331, "Data8"=w1330, "ID"=w1338, "选项卡数值"=enum32{"单体电压", "单体温度", "单体内阻", "单体SOC"}."单体电压") -> ("位置"=w1340:i32[], "数据"=w1339:dbl[], "PF"=w1341:i32)  [unwired: 14 in, 5 out]
                n1585 = global write "单体信息全局.vi" "位置"(w1340) -> ()
                n1586 = global write "单体信息全局.vi" "数据"(w1339) -> ()
                n1587 = global write "单体信息全局.vi" "PF"(w1341) -> ()
              }
            }
          }
          frame 16 {
            n1588 = call-by-ref "?"("Data1"=w1350, "Data2"=w1349, "Data3"=w1348, "Data4"=w1347, "Data5"=w1346, "Data6"=w1345, "Data7"=w1344, "Data8"=w1343, "ID"=w1351, "选项卡数值"=enum32{"单体电压", "单体温度", "单体内阻", "单体SOC"}."单体温度") -> ("位置"=w1353:i32[], "数据"=w1352:dbl[], "PF"=w1354:i32)  [unwired: 14 in, 5 out]
            n1589 = global write "单体信息全局.vi" "数据 2"(w1352) -> ()
            n1590 = global write "单体信息全局.vi" "位置 2"(w1353) -> ()
            n1591 = global write "单体信息全局.vi" "PF2"(w1354) -> ()
          }
          frame 20 {
            n1592 = call-by-ref "?"("Data1"=w1364, "Data2"=w1363, "Data3"=w1362, "Data4"=w1360, "Data5"=w1359, "Data6"=w1358, "Data7"=w1357, "Data8"=w1356, "ID"=w1361, "选项卡数值"=enum32{"单体电压", "单体温度", "单体内阻", "单体SOC"}."单体SOC") -> ("放电均衡"=w1367:i32[], "充电均衡"=w1368:i32[], "PF"=w1365:i32, "均衡故障"=w1369:dbl[])  [unwired: 14 in, 4 out]
            n1593 = global write "单体信息全局.vi" "放电均衡"(w1367) -> ()
            n1594 = global write "单体信息全局.vi" "充电均衡"(w1368) -> ()
            n1595 = global write "单体信息全局.vi" "均衡故障"(w1369) -> ()
            n1596 = global write "单体信息全局.vi" "均衡PF"(w1365) -> ()
          }
        }
      }
      n1597 = while {
        stop <- w1372 stop-if-true
        n1598 = local read "CAN初始化成功"() -> (w1370:bool)
        n1599 = case shown="真" w1370 {
          frame False {
            n1600 = Wait Until Next ms Multiple(millisecond multiple=u32 200 ("毫秒倍数")) -> ()  [unwired: 1 out]
          }
          frame True {
            n1601 = stacked-sequence {
              frame #0 {
                n1602 = local read "上电状态"() -> (w1391:bool[])
                n1603 = local read "中英文选择"() -> (w1387:enum32{"中文", "English"})
                n1604 = Index Array(array=w1391, index #1=0 ("索引")) -> (element #1=w1390:bool)  [unwired: 1 in, 1 out]
                n1605 = Array Subset(array=w1391, index=1 ("索引"), length=30 ("长度")) -> (w1397:bool[])
                n1606 = Or Array Elements(Boolean array=w1397) -> (logical OR=w1396:bool)
                n1607 = case shown="\"中文\", 默认" w1387 {
                  tunnel: [w1405 w1431] -> w1399
                  tunnel: w1397 -> [w1404 w1430]
                  tunnel: w1396 -> [w1403 w1429]
                  tunnel: [w1402 w1428] -> w1395
                  tunnel: [" " " "] -> w1392
                  tunnel: w1390 -> [w1400 w1426]
                  frame "中文", Default {
                    n1608 = case shown="真" w1400 {
                      tunnel: ["" "主板连接"] -> w1405
                      frame False {
                      }
                      frame True {
                      }
                    }
                    n1609 = case shown="真" w1403 {
                      tunnel: w1404 -> [_ w1412]
                      tunnel: ["" ("trimmed string") w1408] -> w1402
                      frame False {
                      }
                      frame True {
                        n1610 = for {
                          tunnel: w1412 -> [w1416] mode=indexing
                          shift-right: [w1414] -> w1410
                          shift-left: "从板" ("字符串") -> [w1415]
                          i -> [w1413]
                          n1611 = case shown="真" w1416 {
                            tunnel: w1415 -> [w1417 w1423]
                            tunnel: [w1417 w1422] -> w1414
                            tunnel: w1413 -> [_ w1421]
                            frame False {
                            }
                            frame True {
                              n1612 = Increment(x=w1421) -> (x+1=w1420:i32)
                              n1613 = Number To Decimal String(number=w1420) -> (decimal integer string=w1419:string)  [unwired: 1 out]
                              n1614 = Concatenate Strings(w1423, w1419, " " ("字符串")) -> (w1422:string)
                            }
                          }
                        }
                        n1615 = call <vilib>:"Trim Whitespace.vi"("string"=w1410) -> ("trimmed string"=w1409:string)  [unwired: 1 in]
                        n1616 = Concatenate Strings(w1409, "连接" ("字符串")) -> (w1408:string)
                      }
                    }
                  }
                  frame "English" {
                    n1617 = case shown="真" w1426 {
                      tunnel: ["" "BMU_Connect"] -> w1431
                      frame False {
                      }
                      frame True {
                      }
                    }
                    n1618 = case shown="真" w1429 {
                      tunnel: w1430 -> [_ w1438]
                      tunnel: ["" ("trimmed string") w1434] -> w1428
                      frame False {
                      }
                      frame True {
                        n1619 = for {
                          tunnel: w1438 -> [w1442] mode=indexing
                          shift-right: [w1440] -> w1436
                          shift-left: "BCU" ("字符串") -> [w1441]
                          i -> [w1439]
                          n1620 = case shown="真" w1442 {
                            tunnel: w1441 -> [w1443 w1449]
                            tunnel: [w1443 w1448] -> w1440
                            tunnel: w1439 -> [_ w1447]
                            frame False {
                            }
                            frame True {
                              n1621 = Increment(x=w1447) -> (x+1=w1446:i32)
                              n1622 = Number To Decimal String(number=w1446) -> (decimal integer string=w1445:string)  [unwired: 1 out]
                              n1623 = Concatenate Strings(w1449, w1445, " " ("字符串")) -> (w1448:string)
                            }
                          }
                        }
                        n1624 = call <vilib>:"Trim Whitespace.vi"("string"=w1436) -> ("trimmed string"=w1435:string)  [unwired: 1 in]
                        n1625 = Concatenate Strings(w1435, "Connect" ("字符串")) -> (w1434:string)
                      }
                    }
                  }
                }
                n1626 = Concatenate Strings(w1399, w1392, w1395) -> (w1394:string)
                n1627 = call <vilib>:"Trim Whitespace.vi"("string"=w1394) -> ("trimmed string"=→"状态":string)  [unwired: 1 in]
              }
              frame #1 {
                n1628 = call "已用时间2"() -> ("Time has Elapsed"=w1452:bool)  [unwired: 5 in, 14 out]
                n1629 = case shown="真" w1452 {
                  frame False {
                  }
                  frame True {
                    n1630 = local write "上电状态"(bool[] [FALSE, FALSE, FALSE, FALSE, FALSE, FALSE, FALSE, FALSE, FALSE, FALSE, FALSE, FALSE, FALSE, FALSE, FALSE, FALSE, FALSE, FALSE, FALSE, FALSE, FALSE, FALSE, FALSE, FALSE, FALSE, FALSE, FALSE, FALSE, FALSE, FALSE, FALSE] ("上电状态")) -> ()
                  }
                }
              }
              frame #2 {
                n1631 = local read "图表选项卡"() -> (w1454:enum32{"次要参数", "单体电压", "单体温度", "单体内阻"})
                n1632 = case shown="\"单体电压\"" w1454 {
                  frame "次要参数", Default {
                    n1633 = Wait (ms)(milliseconds to wait=u32 900 ("等待时间（毫秒）")) -> ()  [unwired: 1 out]
                  }
                  frame "单体电压" {
                    n1634 = Wait (ms)(milliseconds to wait=u32 900 ("等待时间（毫秒）")) -> ()  [unwired: 1 out]
                    n1635 = global read "从板全局变量.vi" "电池节数"() -> (w1457:u8[])
                    n1636 = global read "单体信息全局.vi" "单体数据"() -> (w1459:dbl[][])
                    n1637 = Add Array Elements(numeric array=w1457) -> (sum=w1456:u8)
                    n1638 = for {
                      tunnel: w1457 -> [w1469] mode=indexing
                      tunnel: w1459 -> [w1472]
                      shift-right: [w1467] -> w1458
                      shift-left: dbl[] [] -> [w1468]
                      tunnel: w1457 -> [w1466]
                      i -> [w1471]
                      n1639 = Greater Than 0?(x=w1469) -> (x > 0?=w1470:bool)
                      n1640 = case shown="真" w1470 {
                        tunnel: w1472 -> [_ w1483]
                        tunnel: w1471 -> [_ w1475]
                        tunnel: w1469 -> [_ w1474]
                        tunnel: w1468 -> [w1473 w1480]
                        tunnel: [w1473 w1481] -> w1467
                        tunnel: w1466 -> [_ w1478]
                        frame False {
                        }
                        frame True {
                          n1641 = Index Array(array=w1483, index (row)=w1475) -> (element=w1482:dbl[])  [unwired: 1 in]
                          n1642 = Array Subset(array=w1482, length=w1474) -> (w1479:dbl[])  [unwired: 1 in]
                          n1643 = Array Subset(array=w1478, length=w1475) -> (w1477:u8[])  [unwired: 1 in]
                          n1644 = Add Array Elements(numeric array=w1477) -> (sum=w1476:u8)
                          n1645 = Insert Into Array(array=w1480, index=w1476, new element=w1479) -> (w1481:dbl[])
                        }
                      }
                    }
                    n1646 = Array Subset(array=w1458, length=w1456) -> (w1462:dbl[])  [unwired: 1 in]
                    n1647 = for {
                      N: w1456 -> [_]
                      tunnel: [w1484] -> w1463 mode=indexing
                      i -> [w1485]
                      n1648 = Increment(x=w1485) -> (x+1=w1484:i32)
                    }
                    n1649 = Bundle(w1463, w1462) -> (→"System XY Graph":cluster{i32[], dbl[]})  [unwired: 1 out]
                    n1650 = Array Size(array=w1462) -> (size(s)=→"大小":i32)
                  }
                  frame "单体温度" {
                    n1651 = global read "从板全局变量.vi" "温度个数"() -> (w1487:u8[])
                    n1652 = global read "单体信息全局.vi" "温度数据"() -> (w1490:sgl[][])
                    n1653 = for {
                      tunnel: w1487 -> [w1505] mode=indexing
                      tunnel: w1490 -> [w1508]
                      shift-right: [w1503] -> w1488
                      shift-left: dbl[] [] -> [w1504]
                      tunnel: w1487 -> [w1502]
                      i -> [w1507]
                      n1654 = Greater Than 0?(x=w1505) -> (x > 0?=w1506:bool)
                      n1655 = case shown="假" w1506 {
                        tunnel: w1508 -> [_ w1519]
                        tunnel: w1507 -> [_ w1511]
                        tunnel: w1505 -> [_ w1510]
                        tunnel: w1504 -> [w1509 w1516]
                        tunnel: [w1509 w1517] -> w1503
                        tunnel: w1502 -> [_ w1514]
                        frame False {
                        }
                        frame True {
                          n1656 = Index Array(array=w1519, index (row)=w1511) -> (element=w1518:sgl[])  [unwired: 1 in]
                          n1657 = Array Subset(array=w1518, length=w1510) -> (w1515:sgl[])  [unwired: 1 in]
                          n1658 = Array Subset(array=w1514, length=w1511) -> (w1513:u8[])  [unwired: 1 in]
                          n1659 = Add Array Elements(numeric array=w1513) -> (sum=w1512:u8)
                          n1660 = Insert Into Array(array=w1516, index=w1512, new element=w1515) -> (w1517:dbl[])
                        }
                      }
                    }
                    n1661 = Wait (ms)(milliseconds to wait=u32 900 ("等待时间（毫秒）")) -> ()  [unwired: 1 out]
                    n1662 = Add Array Elements(numeric array=w1487) -> (sum=w1486:u8)
                    n1663 = Array Subset(array=w1488, length=w1486) -> (w1491:dbl[])  [unwired: 1 in]
                    n1664 = for {
                      N: w1486 -> [_]
                      tunnel: [w1520] -> w1499 mode=indexing
                      i -> [w1521]
                      n1665 = Increment(x=w1521) -> (x+1=w1520:i32)
                    }
                    n1666 = Array Size(array=w1499) -> (size(s)=w1498:i32)
                    n1667 = Bundle(w1499, w1491) -> (→"System XY Graph 3":cluster{i32[], dbl[]})  [unwired: 1 out]
                    n1668 = Greater Or Equal?(x=w1498, y=20) -> (x >= y?=w1496:bool)
                    n1669 = Array Size(array=w1491) -> (size(s)=→"温度个数":i32)
                    n1670 = Select(t=u8 2 ("X标尺.标尺调节"), s=w1496, f=u8 0) -> (s? t:f=w1493:u8)
                    n1671 = property on="System XY Graph 3" class="XYGraph (严格)"("XScale.ScaleFit"=w1493) -> ()  [unwired: 2 in, 2 out]
                  }
                }
              }
            }
            n1672 = local read "电池故障2 4"() -> (w1378:u8)
            n1673 = local read "电池故障3 4"() -> (w1377:u8)
            n1674 = local read "电池故障4 4"() -> (w1376:u8)
            n1675 = local read "电池故障 5"() -> (w1379:u8)
            n1676 = local read "中英文选择"() -> (w1374:enum32{"中文", "English"})
            n1677 = Equal To 0?(x=w1377) -> (x = 0?=w1384:bool)
            n1678 = Equal To 0?(x=w1376) -> (x = 0?=w1383:bool)
            n1679 = Equal To 0?(x=w1379) -> (x = 0?=w1386:bool)
            n1680 = Equal To 0?(x=w1378) -> (x = 0?=w1385:bool)
            n1681 = Build Array(w1386, w1385, w1384, w1383) -> (w1382:bool[])
            n1682 = And Array Elements(Boolean array=w1382) -> (logical AND=w1381:bool)
            n1683 = case shown="\"中文\", 默认" w1374 {
              tunnel: w1381 -> [w1536 w1545]
              tunnel: [w1535 w1544] -> _
              tunnel: [w1534 w1543] -> w1380
              frame "中文", Default {
                n1684 = case shown="真" w1536 {
                  tunnel: [u32 10241033 u32 87470] -> w1535
                  tunnel: ["故障模式!" "无故障"] -> w1534
                  frame False {
                    n1685 = property on="故障信息概况" class="Str"("Visible"=TRUE ("可见")) -> ()  [unwired: 2 in, 2 out]
                  }
                  frame True {
                    n1686 = property on="故障信息概况" class="Str"("Visible"=FALSE ("可见")) -> ()  [unwired: 2 in, 2 out]
                  }
                }
              }
              frame "English" {
                n1687 = case shown="真" w1545 {
                  tunnel: [u32 10241033 u32 87470] -> w1544
                  tunnel: ["Fault" "No_Fault"] -> w1543
                  frame False {
                  }
                  frame True {
                  }
                }
              }
            }
            n1688 = local write "故障信息概况"(w1380) -> ()
            n1689 = call "已用时间5"() -> ("Time has Elapsed"=w1375:bool)  [unwired: 12 in, 7 out]
            n1690 = case shown="真" w1375 {
              frame False {
              }
              frame True {
                n1691 = stacked-sequence {
                  frame #0 {
                    w1527 = 0.0 ("外总压")
                    n1692 = local read "充电超时4"() -> (w1523:i32)
                    n1693 = local read "充电超时3"() -> (w1524:i32)
                    n1694 = local read "Life超时"() -> (w1522:i32)
                    n1695 = local read "充电超时2"() -> (w1525:i32)
                    n1696 = local read "充电超时1"() -> (w1526:i32)
                    n1697 = case shown="0, 默认" w1522 {
                      frame 0, Default {
                        n1698 = global write "EV05全局变量1.vi" "life"(0.0 ("life")) -> ()
                      }
                      frame 1 {
                      }
                    }
                    n1699 = case shown="0, 默认" w1525 {
                      tunnel: w1527 -> [w1531 _]
                      frame 0, Default {
                        n1700 = global write "电池信息全局变量.vi" "累计充电时间"(w1531) -> ()
                        n1701 = global write "电池信息全局变量.vi" "剩余充电时间"(w1531) -> ()
                        n1702 = global write "电池信息全局变量.vi" "最高允许充电总电压"(w1531) -> ()
                        n1703 = global write "电池信息全局变量.vi" "最高允许充电单体电压"(w1531) -> ()
                      }
                      frame 1 {
                      }
                    }
                    n1704 = case shown="0, 默认" w1524 {
                      tunnel: w1527 -> [w1530 _]
                      frame 0, Default {
                        n1705 = global write "电池信息全局变量.vi" "充电电流步长"(w1530) -> ()
                        n1706 = global write "电池信息全局变量.vi" "最大允许充电电流"(w1530) -> ()
                        n1707 = global write "电池信息全局变量.vi" "最小允许充电电流"(w1530) -> ()
                        n1708 = global write "电池信息全局变量.vi" "最高允许充电温度"(w1530) -> ()
                      }
                      frame 1 {
                      }
                    }
                    n1709 = case shown="0, 默认" w1523 {
                      tunnel: w1527 -> [w1529 _]
                      frame 0, Default {
                        n1710 = global write "电池信息全局变量.vi" "充电机输出电压"(w1529) -> ()
                        n1711 = global write "电池信息全局变量.vi" "充电机输出电流"(w1529) -> ()
                        n1712 = global write "电池信息全局变量.vi" "充电机累计输出能量"(w1529) -> ()
                      }
                      frame 1 {
                      }
                    }
                    n1713 = case shown="0, 默认" w1526 {
                      frame 0, Default {
                        n1714 = global write "电池信息全局变量.vi" "列1"(dbl[] [] ("列1")) -> ()
                      }
                      frame 1 {
                      }
                    }
                  }
                  frame #1 {
                    w1533 = 0 ("充电超时1")
                    n1715 = local write "充电超时3"(w1533) -> ()
                    n1716 = local write "充电超时1"(w1533) -> ()
                    n1717 = local write "充电超时2"(w1533) -> ()
                    n1718 = local write "充电超时4"(w1533) -> ()
                    n1719 = local write "数值"(w1533) -> ()
                    n1720 = local write "Life超时"(w1533) -> ()
                  }
                }
              }
            }
          }
        }
        n1721 = Wait (ms)(milliseconds to wait=u32 100 ("等待时间（毫秒）")) -> ()  [unwired: 1 out]
        n1722 = local read "退出"() -> (w1372:bool)
      }
      n1723 = while {
        tunnel: w114 -> [w2516]
        tunnel: w113 -> [w2515]
        tunnel: [w2514] -> w122
        tunnel: [w2513] -> w118
        tunnel: w121 -> [w2511]
        tunnel: w106 -> [w2510]
        tunnel: [w2509] -> w116
        tunnel: [w2508] -> w119
        tunnel: w112 -> [w2507]
        tunnel: w106 -> [w2506]
        stop <- w2512 stop-if-true
        n1724 = local read "退出"() -> (w2512:bool)
        n1725 = Dequeue Element(queue=w2507, timeout in ms (-1)=200 ("超时毫秒(-1)"), error in (no error)=w2506) -> (element=w2504:T8, error out=w2505:errorcluster)  [unwired: 2 out]
        n1726 = case shown="无错误" w2505 {
          tunnel: w2516 -> [w2524 w2570]
          tunnel: w2515 -> [w2527 w2569]
          tunnel: [w2523 w2570] -> w2514
          tunnel: [w2522 w2569] -> w2513
          tunnel: w2511 -> [w2525 w2567]
          tunnel: w2510 -> [w2526 w2566]
          tunnel: [w2521 w2567] -> w2509
          tunnel: [w2520 w2566] -> w2508
          tunnel: w2504 -> [w2519 _]
          frame No Error {
            n1727 = Unbundle(w2519) -> ("return type"=w2518:u32, "pReceive"=w2517:T18)
            n1728 = for {
              N: w2518 -> [_]
              tunnel: w2527 -> [w2544]
              tunnel: w2526 -> [w2543]
              tunnel: w2525 -> [w2542]
              tunnel: w2524 -> [w2541]
              tunnel: [w2528] -> w2523
              tunnel: [w2529] -> w2522
              tunnel: [w2530] -> w2521
              tunnel: [w2531] -> w2520
              tunnel: w2517 -> [w2540] mode=indexing
              n1729 = Unbundle By Name(w2540) -> ("ID"=w2539:u32)
              n1730 = local read "计数 2"() -> (w2534:i32)
              n1731 = call "ID解析.vi"("ID"=w2539) -> ("PDU(1)"=w2538:i32)  [unwired: 6 in, 4 out]
              n1732 = Greater Or Equal?(x=w2534, y=1000000) -> (x >= y?=w2536:bool)
              n1733 = case shown="0, 默认" w2538 {
                tunnel: w2541 -> [w2548 w2555 w2559]
                tunnel: w2544 -> [w2547 w2557 w2558]
                tunnel: [w2548 w2554 w2559] -> w2528
                tunnel: [w2547 w2556 w2558] -> w2529
                tunnel: w2540 -> [_ w2552 w2563]
                tunnel: w2542 -> [w2546 w2553 w2564]
                tunnel: w2543 -> [w2545 w2551 w2562]
                tunnel: [w2546 w2550 w2561] -> w2530
                tunnel: [w2545 w2549 w2560] -> w2531
                frame 0, Default {
                }
                frame 4 {
                  n1734 = Enqueue Element(queue=w2553, element=w2552, error in (no error)=w2551) -> (queue out=w2550:refnum<queue>, error out=w2549:errorcluster)  [unwired: 2 out]
                  n1735 = Enqueue Element(queue=w2555, element=w2552, error in (no error)=w2557) -> (queue out=w2554:refnum<queue>, error out=w2556:errorcluster)  [unwired: 2 out]
                }
                frame 8, 16, 20 {
                  n1736 = Enqueue Element(queue=w2564, element=w2563, error in (no error)=w2562) -> (queue out=w2561:refnum<queue>, error out=w2560:errorcluster)  [unwired: 2 out]
                }
              }
              n1737 = Increment(x=w2534) -> (x+1=w2533:i32)
              n1738 = Select(t=0 ("y"), s=w2536, f=w2533) -> (s? t:f=w2532:i32)
              n1739 = local write "计数 2"(w2532) -> ()
            }
          }
          frame Error {
            n1740 = local write "计数 2"(0 ("计数 2")) -> ()
            n1741 = Wait Until Next ms Multiple(millisecond multiple=u32 50) -> ()  [unwired: 1 out]
          }
        }
      }
      n1742 = while {
        tunnel: w112 -> [w217]
        tunnel: w106 -> [w216]
        tunnel: [w215] -> w109
        tunnel: [w214] -> w110
        stop <- w218 stop-if-true
        n1743 = local read "CAN初始化成功"() -> (w219:bool)
        n1744 = local read "退出"() -> (w218:bool)
        n1745 = case shown="真" w219 {
          tunnel: w217 -> [w221 w228]
          tunnel: w216 -> [w220 w224]
          tunnel: [w221 w227] -> w215
          tunnel: [w220 w226] -> w214
          frame False {
            n1746 = Wait Until Next ms Multiple(millisecond multiple=u32 50) -> ()  [unwired: 1 out]
          }
          frame True {
            n1747 = local read "设备索引号"() -> (w230:u16)
            n1748 = local read "CAN端口"() -> (w229:u16)
            n1749 = local read "CAN卡类型"() -> (w231:u32)
            n1750 = call "receiver-8.6.vi"("错误输入（无错误）"=w224, "CAN端口"=w229, "设备索引号"=w230, "CAN卡类型"=w231) -> ("错误输出"=w232:errorcluster, "输出簇"=w225:T19, "接收成功"=w233:bool)  [unwired: 3 out]
            n1751 = call <vilib>:"Clear Errors.vi"("error in (no error)"=w232) -> ("error out"=w223:errorcluster)  [unwired: 6 out]
            n1752 = local write "状态"(w233) -> ()
            n1753 = case shown="真" w233 {
              tunnel: w228 -> [w235 w244]
              tunnel: w223 -> [w234 w243]
              tunnel: [w235 w238] -> w227
              tunnel: [w234 w237] -> w226
              tunnel: w225 -> [_ w236]
              frame False {
              }
              frame True {
                n1754 = call "已用时间4"("Time Target (s)"=0.5) -> ("Time has Elapsed"=w239:bool)  [unwired: 4 in, 14 out]
                n1755 = Enqueue Element(queue=w244, element=w236, error in (no error)=w243) -> (queue out=w241:refnum<queue>, error out=w240:errorcluster)  [unwired: 2 out]
                n1756 = case shown="真" w239 {
                  tunnel: w241 -> [w246 w254]
                  tunnel: [w246 w253] -> w238
                  tunnel: w240 -> [w245 w248]
                  tunnel: [w245 w247] -> w237
                  frame False {
                  }
                  frame True {
                    n1757 = local read "设备索引号"() -> (w251:u16)
                    n1758 = local read "CAN端口"() -> (w250:u16)
                    n1759 = local read "CAN卡类型"() -> (w252:u32)
                    n1760 = dll-call lib="PTH1labs FBluewave New EnergySVN_Work\tBHN01_BMStrunkBMS_Monitor_优化内存 - 1dataControlCAN.dll" fn="VCI_ClearBuffer"(error in=w248, "DeviceType"=w252, "DeviceInd"=w251, "CANInd"=w250) -> (error out=w249:errorcluster)  [unwired: 3 in, 4 out]
                    n1761 = Flush Queue(queue=w254, error in (no error)=w248) -> (queue out=w253:refnum<queue>, error out=w247:errorcluster)  [unwired: 1 out]
                    n1762 = call <vilib>:"Clear Errors.vi"("error in (no error)"=w249) -> ()  [unwired: 6 in, 1 out]
                  }
                }
              }
            }
          }
        }
      }
      n1763 = property on="故障信息概况" class="Str"("Visible"=FALSE ("可见"), "Blinking"=FALSE ("闪烁")) -> ()  [unwired: 2 in, 2 out]
      n1764 = Merge Errors(w118, w119) -> (w115:errorcluster)
      n1765 = Release Queue(queue=w109, force destroy? (F)=FALSE ("强制销毁？(F)"), error in (no error)=w110) -> (error out=w111:errorcluster)  [unwired: 2 out]
      n1766 = Release Queue(queue=w122, force destroy? (F)=w108, error in (no error)=w115) -> (error out=w123:errorcluster)  [unwired: 2 out]
      n1767 = Release Queue(queue=w116, force destroy? (F)=w108, error in (no error)=w115) -> (error out=w117:errorcluster)  [unwired: 2 out]
      n1768 = call <vilib>:"Clear Errors.vi"("error in (no error)"=w111) -> ()  [unwired: 7 out]
      n1769 = while {
        stop <- w124 stop-if-true
        n1770 = local read "模拟发送"() -> (w125:bool)
        n1771 = local read "退出"() -> (w124:bool)
        n1772 = case shown="真" w125 {
          frame False {
          }
          frame True {
            n1773 = stacked-sequence {
              frame #0 {
                n1774 = call-by-ref "?"() -> ()  [unwired: 14 in, 2 out]
              }
              frame #1 {
                n1775 = local write "模拟发送"(FALSE ("模拟发送")) -> ()
              }
            }
          }
        }
        n1776 = Wait (ms)(milliseconds to wait=u32 1000 ("等待时间（毫秒）")) -> ()  [unwired: 1 out]
      }
      n1777 = call <vilib>:"Clear Errors.vi"("error in (no error)"=w123) -> ()  [unwired: 7 out]
      n1778 = call <vilib>:"Clear Errors.vi"("error in (no error)"=w117) -> ()  [unwired: 7 out]
      n1779 = Quit LabVIEW(quit? (T)=w97) -> ()
    }
  }
  n1780 = property on="电压温度" class="Bool (严格)"("Disabled"=T11."Enabled" ("禁用"), "Visible"=TRUE ("可见")) -> ()  [unwired: 2 in, 2 out]
  n1781 = local write "模拟发送"(FALSE ("模拟发送")) -> ()
  n1782 = local write "dup path"(path "" ("dup path")) -> ()
  "加热" <- w49
  "风机" <- w49
  "充电" <- w49
  "预充" <- w49
  "总负" <- w49
  "总正" <- w49
  "开始保存" <- FALSE ("开始保存")
